vi "Omniax_mDrive_XYZR_2012.vi"() -> ()   [LabVIEW 2015]
uses:
  <vilib>/Utility/file.llb/Read From Spreadsheet File (I64).vi
  <vilib>/Utility/file.llb/Read From Spreadsheet File (string).vi
  <vilib>/Instr/_visa.llb/VISA Configure Serial Port (Instr).vi
  <vilib>/Utility/file.llb/Write To Spreadsheet File (I64).vi
  <vilib>/Utility/file.llb/Write To Spreadsheet File (string).vi
panel:
  in  "Submit":bool
  in  "ELOG":string
  out "Z max step":i32
  in  "V5 position 15360000":i32
  out "IV5CL":bool
  out "IV5OP":bool
  out "R Velocity MVdeg/sec":dbl format="%.3f"
  out "R Position MV deg":dbl
  out "Z Velocity MV mm/sec":dbl format="%.3f"
  out "Z Position MV mm":dbl
  out "Y Velocity MV mm/sec":dbl format="%.3f"
  out "Y Position MV mm":dbl
  out "X Velocity MV mm/sec":dbl format="%.3f"
  out "X Position MV mm":dbl
  out "Presets":i32[][](array[numeric])
  in  "stop":bool
  in  "Tab Control 3":enum32{"Status", "Reset"}(tab)
  out "Y in Range":bool
  out "Y Scan":bool
  out "Y in Motion":bool
  out "Y Backlash corr":bool
  out "X  in Range":bool
  out "X Scan":bool
  out "X  in Motion":bool
  out "X Backlash corr":bool
  out "Z in Range":bool
  out "Z Scan":bool
  out "Z in Motion":bool
  out "Z Backlash corr":bool
  out "R in Range":bool
  out "R Scan":bool
  out "R in Motion":bool
  out "R Backlash corr":bool
  out "X Ready":bool
  out "Y Ready":bool
  out "Z Ready":bool
  out "R Ready":bool
  in  "Reset Y Position mm":dbl
  out "Reset Y Motor Steps":i32
  in  "Reset X Position mm":dbl
  out "Reset X Motor Steps":i32
  in  "Reset Z Position mm":dbl
  out "Reset Z Motor Steps":i32
  in  "Reset R Position deg":dbl
  out "Reset R Motor Steps":i32
  in  "Reset":bool
  in  "Tab Control 2":enum32{"mm", "step"}(tab)
  in  "X Scan Length SP mm":dbl
  in  "X Scan Velocity SP mm/sec":dbl
  in  "X Scan set":bool
  in  "Y Scan Length SP mm":dbl
  in  "Y Scan Velocity SP mm/sec":dbl
  in  "Y Scan set":bool
  in  "Z Scan Length SP mm":dbl
  in  "Z Scan Velocity SP mm/sec":dbl
  in  "Z Scan set":bool
  in  "R Scan Length SP deg":dbl
  in  "R Scan Velocity SP deg/sec":dbl
  in  "R Scan set":bool
  in  "X Scan Velocity SP steps/sec":i32=1 min=1 max=102400 step=1
  in  "X Scan Length SP steps":i32 min=-2816000 max=1792000 step=100
  out "X Scan length MV mm":dbl
  out "X Scan velocity MV mm/sec":dbl format="%#_6f"
  in  "Y Scan Velocity SP steps/sec":i32=1 min=1 max=102400 step=1
  in  "Y Scan Length SP steps":i32 min=-1930240 max=2677760 step=100
  out "Y Scan length MV mm":dbl
  out "Y Scan velocity MV mm/sec":dbl format="%#_6f"
  in  "Z Scan Velocity SP steps/sec":i32=1 min=1 max=102400 step=1
  in  "Z Scan Length SP steps":i32 min=-91980800 max=10419200 step=100
  out "Z Scan length MV mm":dbl
  out "Z Scan velocity MV mm/sec":dbl format="%#_6f"
  in  "R Scan Velocity SP steps/sec":i32=1 min=1 max=102400 step=1
  in  "R Scan Length SP steps":i32 min=-1501867 max=10786133 step=100
  out "R Scan length MV deg":dbl
  out "R Scan velocity MV deg/sec":dbl format="%#_6f"
  out "atan Y/Z":dbl
  in  "Tab Control":enum32{"mm", "preset", "step"}(tab)
  in  "X Position SP mm":dbl
  in  "X Velocity SP mm/sec":dbl
  in  "X Move Set":bool
  in  "Y Move Set":bool
  in  "Y Position SP mm":dbl
  in  "Y Velocity SP mm/sec":dbl
  in  "Z Position SP mm":dbl
  in  "Z Velocity SP mm/sec":dbl
  in  "Z Move Set":bool
  in  "R Position SP deg":dbl
  in  "R Velocity SP deg/sec":dbl
  in  "R Move Set":bool
  in  "Add Button":bool
  in  "String":string
  in  "Delete Button":bool
  in  "Preset positions":i32(ring) items=["ZERO", "Default", "CDOSE", "QMS", "test", "test2", "test3", "yag position", "Sample Long Edge  ", "SPUTTER POS"]
  in  "Set Button":bool
  in  "X Velocity SP step/sec":i32 min=1 max=128000
  in  "Y Velocity SP step/sec":i32 min=1 max=128000
  in  "Z Velocity SP step/sec":i32 min=1 max=204800
  in  "R Velocity SP step/sec":i32 min=1 max=10000
  in  "Y Step SP":i32=-20000 min=-2304000 max=2304000 step=500
  in  "X Step SP":i32=-20000 min=-2304000 max=2304000 step=500
  in  "Z Step SP":i32=-20000 min=0 max=102400000 step=500
  in  "R Step SP":i32=-20000 min=-6144000 max=6144000 step=500
  out "X Step PV":i32 max=2000
  out "Y Step PV":i32 max=2000
  out "Z Step PV":i32 max=2000
  out "R Step PV":i32 max=2000
  in  "Clear ZY":bool
  out "ZY Graph":cluster{"Y":dbl[], "Y":dbl[]}[](graph)
  out "ZR Graph":cluster{"Y":dbl[], "Y":dbl[]}[](graph)
  out "XY Graph":cluster{"Y":dbl[], "Y":dbl[]}[](graph)
  out "X Scan Duration":dbl
  out "Y Scan Duration":dbl
  out "Z Scan Duration":dbl
  out "R Scan Duration":dbl
  out "R Backlash steps/sec":i32
  out "R Backlash":i32
  out "R Holding Current %":i32
  out "R Run Current %":i32
  out "R offset deg":dbl
  out "R deg/rev":dbl
  out "R steps/rev":u32
  out "R velocity PV step/sec":i32
  out "R MINPOS":i32=-94296
  out "R MAXPOS":i32=-34296
  out "R COM PORT":refnum<visa-resource-name>="COM5"
  in  "R Scan OK":bool
  in  "R Go":bool
  out "R Position deg PV":dbl
  out "Z COM PORT":refnum<visa-resource-name>="COM5"
  out "Z Backlash steps/sec":i32
  out "Z Backlash":i32
  out "Z Holding Current %":i32
  out "Z Run Current %":i32
  out "Z offset mm":dbl
  out "Z mm/rev":dbl
  out "Z steps/rev":u32
  out "Z  velocity PV step/sec":i32
  out "Z MINPOS":i32=-94296
  out "Z MAXPOS":i32=-34296
  in  "Z Scan OK":bool
  in  "Z Go":bool
  out "Z Position mm PV":dbl
  out "X Position mm PV":dbl
  out "X velocity PV step/sec":i32
  in  "X Scan OK":bool
  in  "X Go":bool
  out "X Backlash steps/sec":i32
  out "X Backlash":i32
  out "X Holding Current %":i32
  out "X Run Current %":i32
  out "X offset mm":dbl
  out "X mm/rev":dbl
  out "X steps/rev":u32
  out "X MAXPOS":i32=-34296
  out "X MINPOS":i32=-94296
  out "X COM PORT":refnum<visa-resource-name>="COM5"
  out "Y Backlash steps/sec":i32
  out "Y Backlash":i32
  out "Y Holding Current %":i32
  out "Y Run Current %":i32
  in  "Scan Cancel":bool
  out "Y Position mm PV":dbl
  out "Y offset mm":dbl
  out "Y mm/rev":dbl
  out "Y steps/rev":u32
  out "Y velocity PV step/sec":i32
  in  "Y Scan OK":bool
  in  "Scan Go":bool
  in  "Stop":bool
  in  "Y Go":bool
  out "Y MINPOS":i32=-94296
  out "Y MAXPOS":i32=-34296
  out "Y COM PORT":refnum<visa-resource-name>="COM5"
  # "12-15"
  # "Current position"
  # "Goto position"
  # "MX"
  # "MY"
  # "V5"
  # "MZ"
  # "MR"
  # "L"
  # "M"
  # "B"
  # "S"
  # "R"
  # "Preset position"
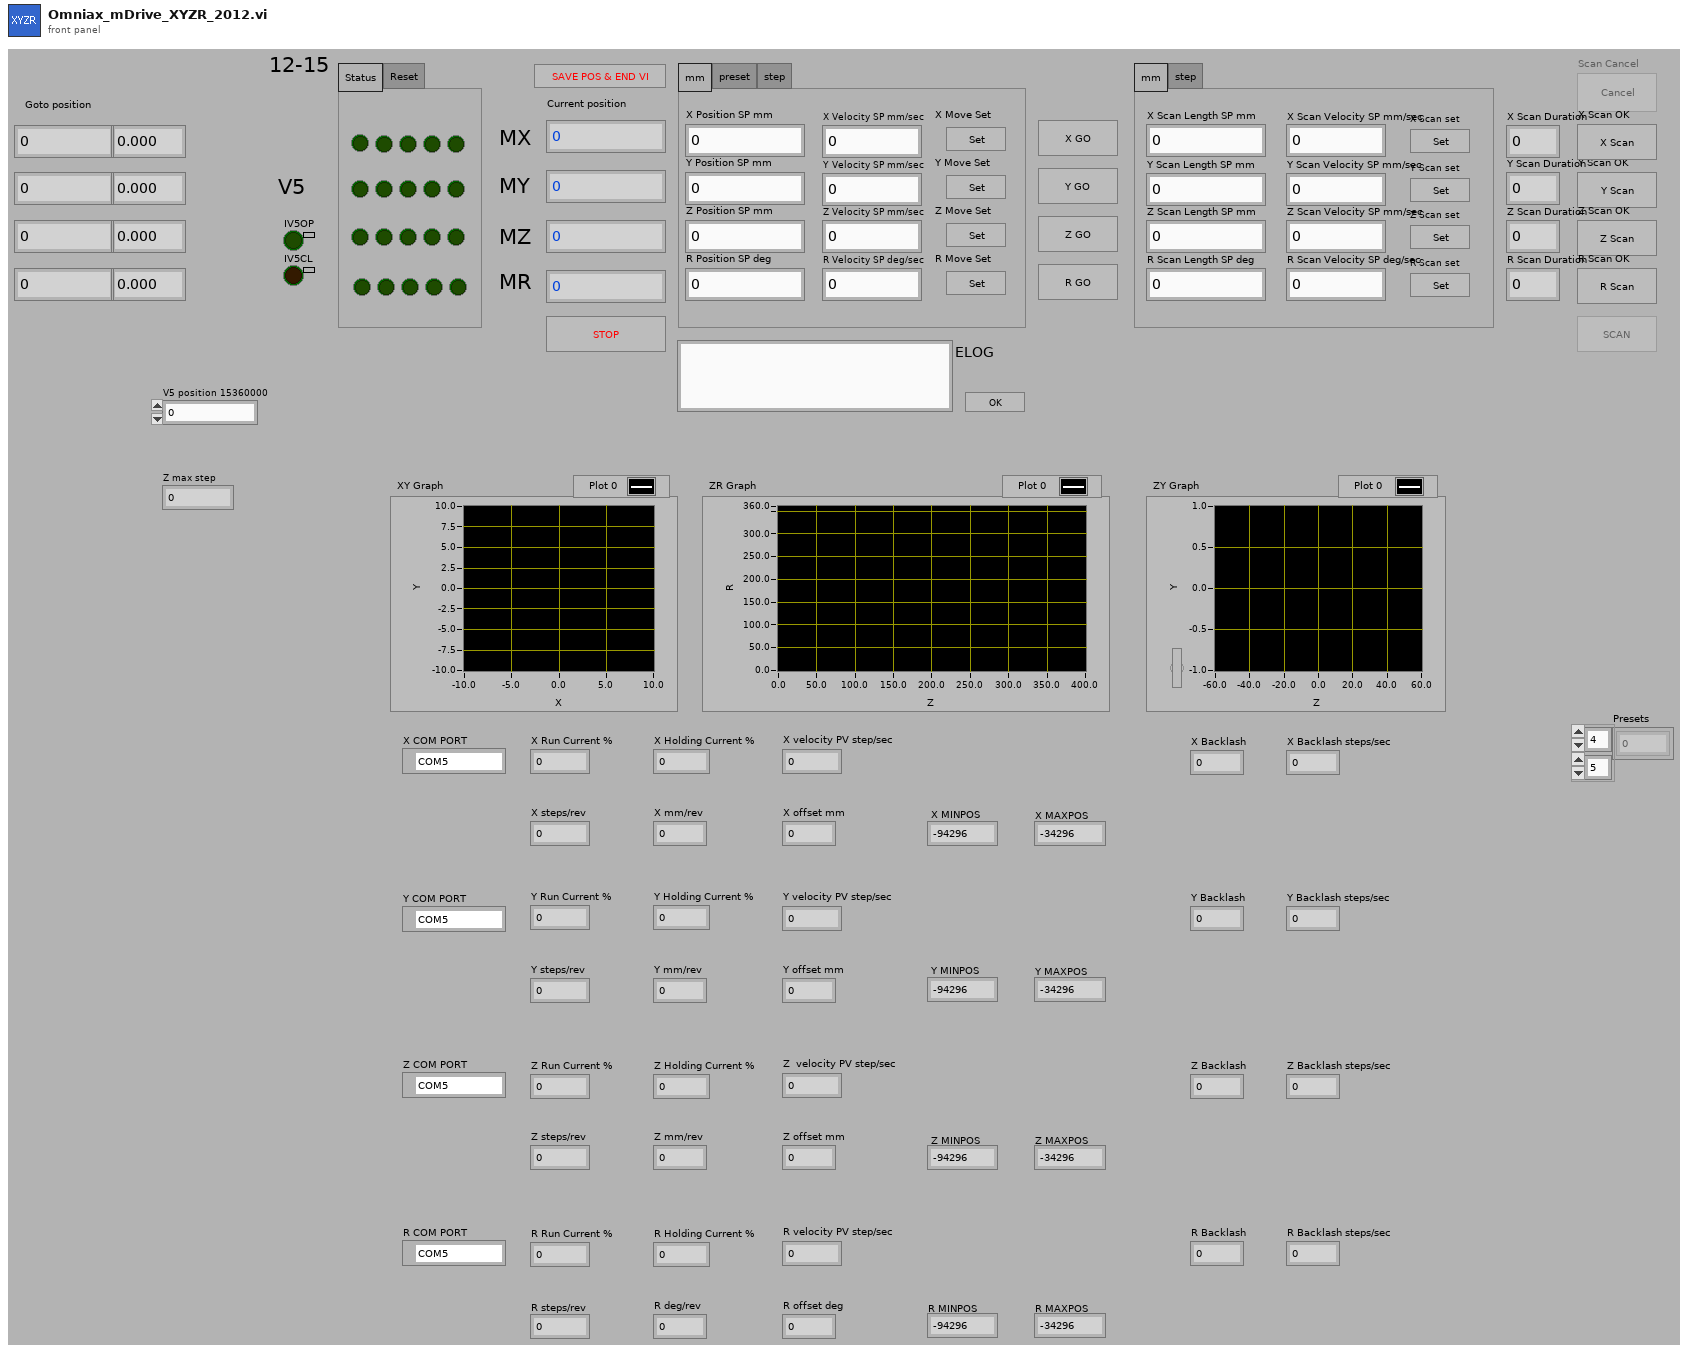
[diagram p1: front panel]
types:
  T1 = enum16{"Stop", "Reset", "Run Current", "Holding Current", "Accel Rate", "Decel Rate", "Move to Relative Position", "Move to Absolute Position", "Echo Mode", "Print Parameter", "Send String", "Microstep Resolution", "Set Current Position", "Max Velocity"}
  T2 = enum8{"Enabled", "Disabled", "Disabled and Grayed Out"}
  T3 = cluster{"first row[0]":i64, "first row[1]":i64, "first row[2]":i64, "first row[3]":i64, "first row[4]":i64, "first row[5]":i64, "first row[6]":i64, "first row[7]":i64, "first row[8]":i64}
  T4 = enum16{"open", "replace", "create", "open or create", "replace or create", "replace or create with confirmation"}
  T5 = cluster{"Value[0]":i32, "Value[1]":i32, "Value[2]":i32, "Value[3]":i32, "Value[4]":i32, "Value[5]":i32, "Value[6]":i32, "Value[7]":i32, "Value[8]":i32}
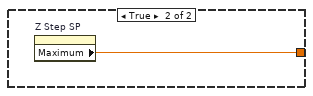
[diagram p6: hidden frame]
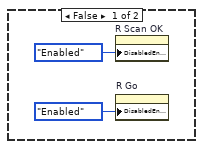
[diagram p7: hidden frame]
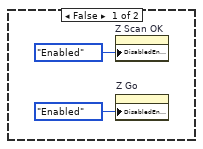
[diagram p10: hidden frame]
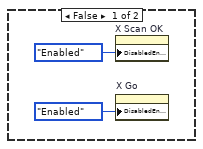
[diagram p13: hidden frame]
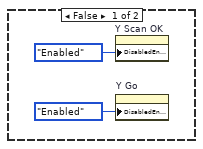
[diagram p16: hidden frame]
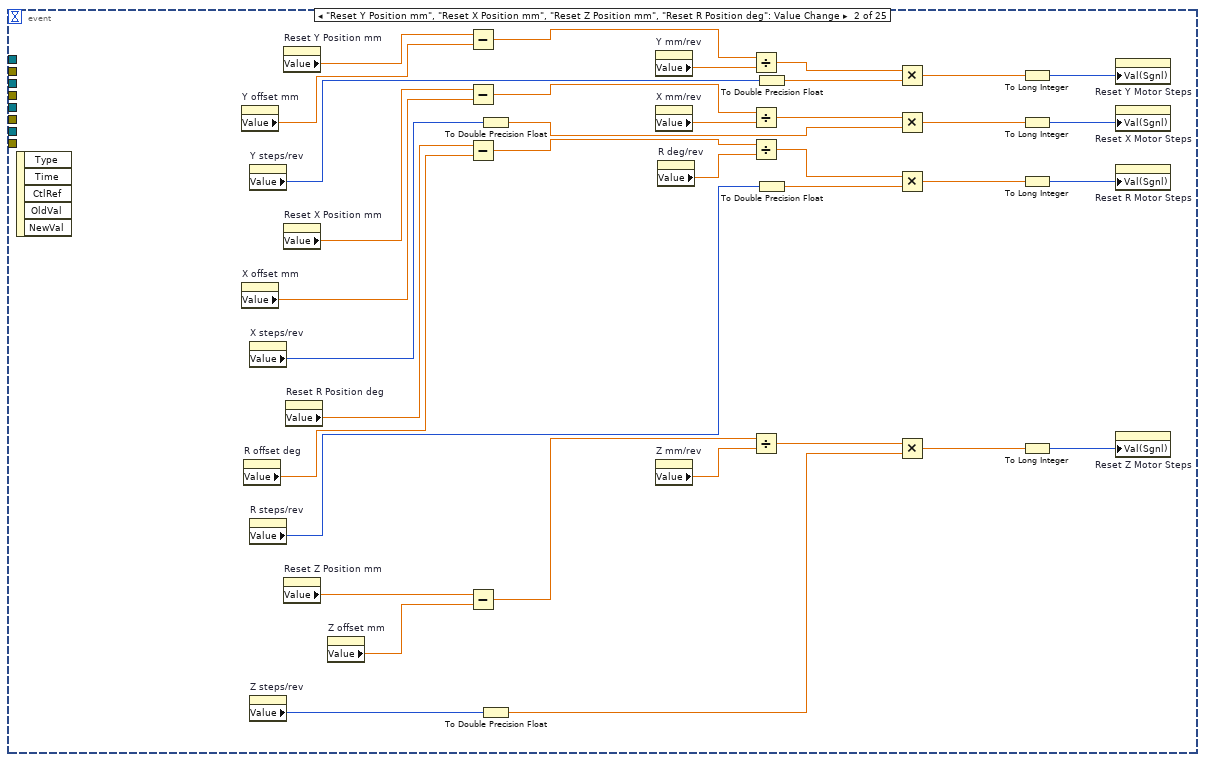
[diagram p19: hidden frame]
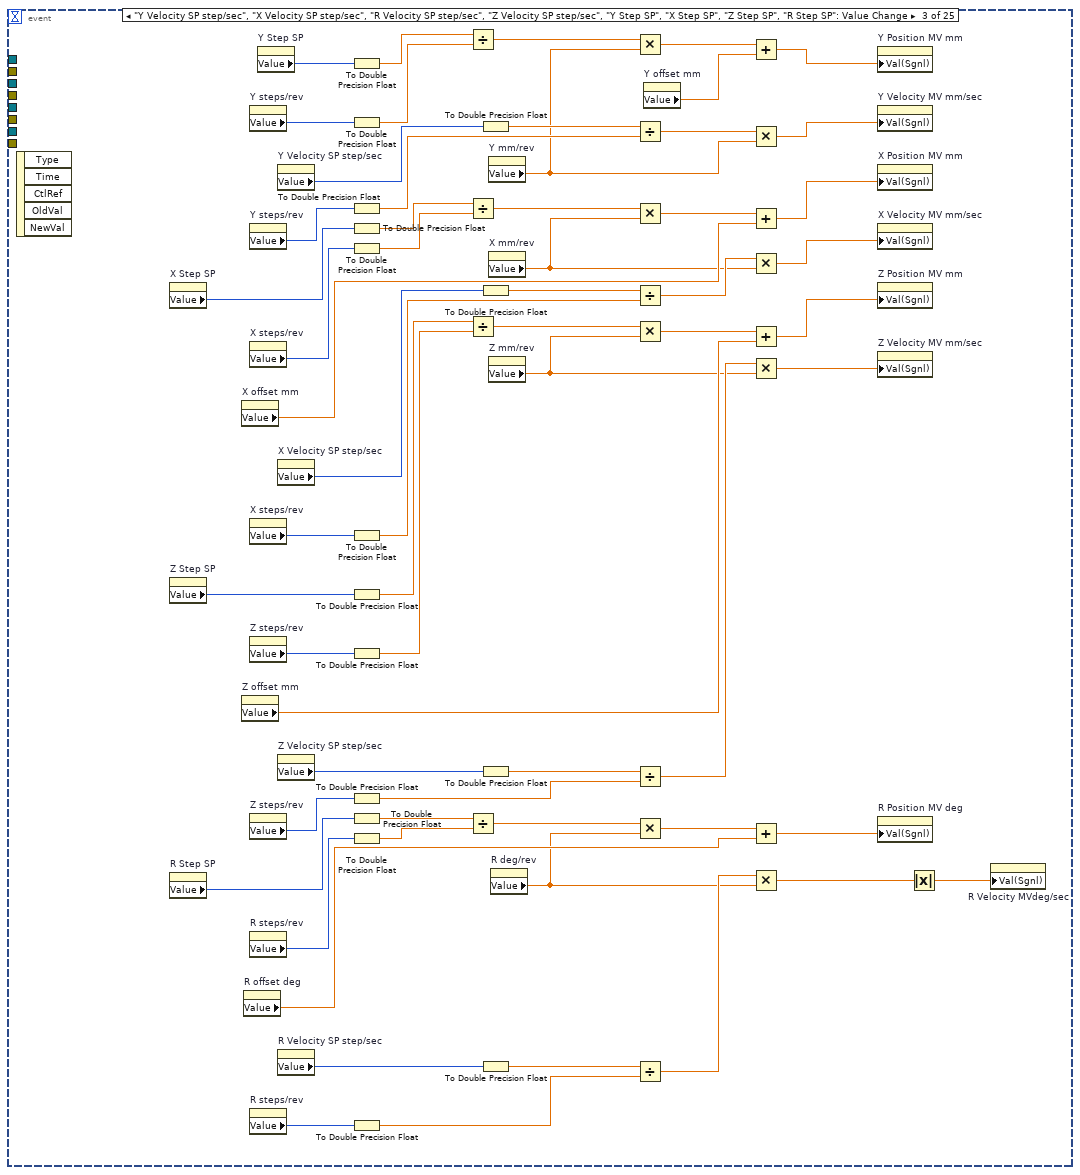
[diagram p20: hidden frame]
diagram:
  w4 = 0 ("dimension size")
  n1 = call "DigitalIO_sub_V5_MON.vi"() -> ("CL"=→"IV5CL":bool, "OP"=→"IV5OP":bool)  [unwired: 8 in]
  n2 = flat-sequence {
    tunnel: [w108] -> w36
    tunnel: [w107] -> w35
    tunnel: [w118] -> w52
    tunnel: [w116] -> w50
    tunnel: w36 -> [w119]
    tunnel: w35 -> [w117]
    tunnel: w52 -> [w125]
    tunnel: [w126] -> w51
    tunnel: w50 -> [w122]
    tunnel: [w124] -> w49
    tunnel: [w135] -> w102
    tunnel: [w137] -> w100
    tunnel: w51 -> [w136]
    tunnel: w49 -> [w138]
    tunnel: w102 -> [w145]
    tunnel: [w144] -> w101
    tunnel: w100 -> [w142]
    tunnel: [w143] -> w99
    tunnel: [w155] -> w104
    tunnel: [w156] -> w103
    tunnel: w101 -> [w154]
    tunnel: w99 -> [w153]
    tunnel: w104 -> [w166]
    tunnel: w103 -> [w165]
    tunnel: [w168] -> w88
    tunnel: [w167] -> w87
    tunnel: [w162] -> w86
    tunnel: [w173] -> w105
    tunnel: [w174] -> w106
    tunnel: w88 -> [w174]
    tunnel: w87 -> [w173]
    tunnel: w86 -> [w169]
    frame #0 {
      w115 = refnum<visa-resource-name> "COM13" ("COM PORT")
      w113 = u16 0 items=["None", "XON/XOFF", "RTS/CTS", "XON/XOFF & RTS/CTS", "DTR/DSR", "XON/XOFF & DTR/DSR"] ("flow control (0:none)")
      w112 = u16 10 items=["1.0"=10, "1.5"=15, "2.0"=20] ("stop bits (10: 1 bit)")
      # "Stop bits"
      n3 = call-poly "VISA Configure Serial Port"("VISA resource name"=w115, "timeout (10sec)"=u32 10000, "baud rate (9600)"=u32 9600, "data bits (8)"=u16 8, "parity (0:none)"=enum16{"None", "Odd", "Even", "Mark", "Space"}."None", "stop bits (10: 1 bit)"=w112, "flow control (0:none)"=w113) -> ("VISA resource name out"=w108:refnum<visa-resource-name>, "error out"=w107:errorcluster)  [unwired: 7 in]
      "Y COM PORT" <- w115
    }
    frame #1 {
      n4 = call "mDrive Send Command.vi"("error in (no error)"=w117, "Extra"="EM=2", "Command"=T1."Send String", "VISA resource name"=w119) -> ("error out"=w116:errorcluster, "VISA resource name out"=w118:refnum<visa-resource-name>)  [unwired: 3 in, 1 out]
    }
    frame #2 {
      n5 = Number To Decimal String(number=1000000) -> (decimal integer string=w127:string)  [unwired: 1 in]
      n6 = call "mDrive Send Command.vi"("error in (no error)"=w122, "Extra"=w127, "Command"=T1."Accel Rate", "VISA resource name"=w125) -> ("error out"=w123:errorcluster, "VISA resource name out"=w131:refnum<visa-resource-name>)  [unwired: 3 in, 1 out]
      n7 = call "mDrive Send Command.vi"("error in (no error)"=w123, "Extra"=w127, "Command"=T1."Decel Rate", "VISA resource name"=w131) -> ("error out"=w124:errorcluster, "VISA resource name out"=w126:refnum<visa-resource-name>)  [unwired: 3 in, 1 out]
    }
    frame #3 {
      # "Run Current %"
      n8 = property on="Y Run Current %" class="DigNum (strict)"() -> ("Value"=w133:i32)  [unwired: 2 in, 2 out]
      n9 = Number To Decimal String(number=w133) -> (decimal integer string=w134:string)  [unwired: 1 in]
      n10 = call "mDrive Send Command.vi"("error in (no error)"=w138, "Extra"=w134, "Command"=T1."Run Current", "VISA resource name"=w136) -> ("error out"=w137:errorcluster, "VISA resource name out"=w135:refnum<visa-resource-name>)  [unwired: 3 in, 1 out]
    }
    frame #4 {
      # "Holding Current %"
      n11 = property on="Y Holding Current %" class="DigNum (strict)"() -> ("Value"=w140:i32)  [unwired: 2 in, 2 out]
      n12 = Number To Decimal String(number=w140) -> (decimal integer string=w141:string)  [unwired: 1 in]
      n13 = call "mDrive Send Command.vi"("error in (no error)"=w142, "Extra"=w141, "Command"=T1."Holding Current", "VISA resource name"=w145) -> ("error out"=w143:errorcluster, "VISA resource name out"=w144:refnum<visa-resource-name>)  [unwired: 3 in, 1 out]
    }
    frame #5 {
      # "Velocity Max"
      n14 = property on="Y Velocity SP step/sec" class="DigNum (strict)"() -> ("Value"=w152:i32)  [unwired: 2 in, 2 out]
      n15 = Number To Decimal String(number=w152) -> (decimal integer string=w151:string)  [unwired: 1 in]
      n16 = call "mDrive Send Command.vi"("error in (no error)"=w153, "Extra"=w151, "Command"=T1."Max Velocity", "VISA resource name"=w154) -> ("error out"=w149:errorcluster, "VISA resource name out"=w159:refnum<visa-resource-name>)  [unwired: 3 in, 1 out]
      n17 = call "mDrive Send Command.vi"("error in (no error)"=w149, "Extra"="VM", "Command"=T1."Print Parameter", "VISA resource name"=w159) -> ("error out"=w156:errorcluster, "read buffer"=w157:string, "VISA resource name out"=w155:refnum<visa-resource-name>)  [unwired: 3 in]
      n18 = Decimal String To Number(string=w157, offset=0) -> (number=w150:i32)  [unwired: 1 in, 1 out]
      n19 = property on="Y scan velocity MV step/sec" class="DigNum (strict)"("Val(Sgnl)"=w150) -> ()  [unwired: 2 in, 2 out]
    }
    frame #6 {
      # "PRINT POSITION"
      n20 = call "mDrive Send Command.vi"("error in (no error)"=w165, "Extra"="P", "Command"=T1."Print Parameter", "VISA resource name"=w166) -> ("error out"=w167:errorcluster, "read buffer"=w164:string, "VISA resource name out"=w168:refnum<visa-resource-name>)  [unwired: 3 in]
      n21 = Decimal String To Number(string=w164, offset=0) -> (number=w162:i32)  [unwired: 1 in, 1 out]
    }
    frame #7 {
      w171 = -2304000 ("lower limit")
      w172 = 2304000 ("upper limit")
      n22 = property on="Y Step SP" class="DigNum (strict)"("Val(Sgnl)"=w169) -> ()  [unwired: 2 in, 2 out]
      n23 = property on="Y Step SP" class="DigNum (strict)"("Maximum"=w172) -> ()  [unwired: 2 in, 2 out]
      n24 = In Range and Coerce(upper limit=w172, x=w169, lower limit=w171) -> (In Range?=w170:bool)  [unwired: 1 out]
      n25 = property on="Y Step SP" class="DigNum (strict)"("Minimum"=w171) -> ()  [unwired: 2 in, 2 out]
      n26 = property on="Y in Range" class="Bool (strict)"("Val(Sgnl)"=w170) -> ()  [unwired: 2 in, 2 out]
      "Y MINPOS" <- w171
      "Y MAXPOS" <- w172
    }
  }
  n27 = flat-sequence {
    tunnel: [w176] -> w38
    tunnel: [w175] -> w37
    tunnel: [w184] -> w56
    tunnel: [w186] -> w54
    tunnel: w38 -> [w185]
    tunnel: w37 -> [w187]
    tunnel: w56 -> [w191]
    tunnel: [w192] -> w55
    tunnel: w54 -> [w190]
    tunnel: [w193] -> w53
    tunnel: [w204] -> w73
    tunnel: [w206] -> w72
    tunnel: w55 -> [w205]
    tunnel: w53 -> [w200]
    tunnel: w73 -> [w213]
    tunnel: [w212] -> w71
    tunnel: w72 -> [w210]
    tunnel: [w211] -> w70
    tunnel: [w223] -> w69
    tunnel: [w224] -> w68
    tunnel: w71 -> [w222]
    tunnel: w70 -> [w221]
    tunnel: w69 -> [w234]
    tunnel: w68 -> [w233]
    tunnel: [w236] -> w67
    tunnel: [w235] -> w66
    tunnel: [w230] -> w65
    tunnel: [w243] -> w61
    tunnel: [w244] -> w62
    tunnel: w67 -> [w244]
    tunnel: w66 -> [w243]
    tunnel: w65 -> [w241]
    frame #0 {
      w183 = refnum<visa-resource-name> "COM15" ("COM PORT")
      w181 = u16 0 items=["None", "XON/XOFF", "RTS/CTS", "XON/XOFF & RTS/CTS", "DTR/DSR", "XON/XOFF & DTR/DSR"] ("flow control (0:none)")
      w180 = u16 10 items=["1.0"=10, "1.5"=15, "2.0"=20] ("stop bits (10: 1 bit)")
      # "Stop bits"
      n28 = call-poly "VISA Configure Serial Port"("VISA resource name"=w183, "timeout (10sec)"=u32 10000, "baud rate (9600)"=u32 9600, "data bits (8)"=u16 8, "parity (0:none)"=enum16{"None", "Odd", "Even", "Mark", "Space"}."None", "stop bits (10: 1 bit)"=w180, "flow control (0:none)"=w181) -> ("VISA resource name out"=w176:refnum<visa-resource-name>, "error out"=w175:errorcluster)  [unwired: 7 in]
      "R COM PORT" <- w183
    }
    frame #1 {
      n29 = call "mDrive Send Command.vi"("error in (no error)"=w187, "Extra"="EM=2", "Command"=T1."Send String", "VISA resource name"=w185) -> ("error out"=w186:errorcluster, "VISA resource name out"=w184:refnum<visa-resource-name>)  [unwired: 3 in, 1 out]
    }
    frame #2 {
      # "pr=1000000"
      n30 = Number To Decimal String(number=100000) -> (decimal integer string=w195:string)  [unwired: 1 in]
      n31 = call "mDrive Send Command.vi"("error in (no error)"=w190, "Extra"=w195, "Command"=T1."Accel Rate", "VISA resource name"=w191) -> ("error out"=w194:errorcluster, "VISA resource name out"=w199:refnum<visa-resource-name>)  [unwired: 3 in, 1 out]
      n32 = call "mDrive Send Command.vi"("error in (no error)"=w194, "Extra"=w195, "Command"=T1."Decel Rate", "VISA resource name"=w199) -> ("error out"=w193:errorcluster, "VISA resource name out"=w192:refnum<visa-resource-name>)  [unwired: 3 in, 1 out]
    }
    frame #3 {
      # "Run Current %"
      n33 = property on="R Run Current %" class="DigNum (strict)"() -> ("Value"=w202:i32)  [unwired: 2 in, 2 out]
      n34 = Number To Decimal String(number=w202) -> (decimal integer string=w203:string)  [unwired: 1 in]
      n35 = call "mDrive Send Command.vi"("error in (no error)"=w200, "Extra"=w203, "Command"=T1."Run Current", "VISA resource name"=w205) -> ("error out"=w206:errorcluster, "VISA resource name out"=w204:refnum<visa-resource-name>)  [unwired: 3 in, 1 out]
    }
    frame #4 {
      # "Holding Current %"
      n36 = property on="R Holding Current %" class="DigNum (strict)"() -> ("Value"=w208:i32)  [unwired: 2 in, 2 out]
      n37 = Number To Decimal String(number=w208) -> (decimal integer string=w209:string)  [unwired: 1 in]
      n38 = call "mDrive Send Command.vi"("error in (no error)"=w210, "Extra"=w209, "Command"=T1."Holding Current", "VISA resource name"=w213) -> ("error out"=w211:errorcluster, "VISA resource name out"=w212:refnum<visa-resource-name>)  [unwired: 3 in, 1 out]
    }
    frame #5 {
      # "Print Velocity Max"
      # "Velocity Max"
      n39 = property on="R Velocity SP step/sec" class="DigNum (strict)"() -> ("Value"=w220:i32)  [unwired: 2 in, 2 out]
      n40 = Number To Decimal String(number=w220) -> (decimal integer string=w219:string)  [unwired: 1 in]
      n41 = call "mDrive Send Command.vi"("error in (no error)"=w221, "Extra"=w219, "Command"=T1."Max Velocity", "VISA resource name"=w222) -> ("error out"=w217:errorcluster, "VISA resource name out"=w227:refnum<visa-resource-name>)  [unwired: 3 in, 1 out]
      n42 = call "mDrive Send Command.vi"("error in (no error)"=w217, "Extra"="VM", "Command"=T1."Print Parameter", "VISA resource name"=w227) -> ("error out"=w224:errorcluster, "read buffer"=w225:string, "VISA resource name out"=w223:refnum<visa-resource-name>)  [unwired: 3 in]
      n43 = Decimal String To Number(string=w225, offset=0) -> (number=w218:i32)  [unwired: 1 in, 1 out]
      n44 = property on="R velocity PV step/sec" class="DigNum (strict)"("Val(Sgnl)"=w218) -> ()  [unwired: 2 in, 2 out]
    }
    frame #6 {
      # "PRINT POSITION"
      n45 = call "mDrive Send Command.vi"("error in (no error)"=w233, "Extra"="P", "Command"=T1."Print Parameter", "VISA resource name"=w234) -> ("error out"=w235:errorcluster, "read buffer"=w232:string, "VISA resource name out"=w236:refnum<visa-resource-name>)  [unwired: 3 in]
      n46 = Decimal String To Number(string=w232, offset=0) -> (number=w230:i32)  [unwired: 1 in, 1 out]
    }
    frame #7 {
      n47 = property on="R Step SP" class="DigNum (strict)"("Val(Sgnl)"=w241) -> ()  [unwired: 2 in, 2 out]
      n48 = property on="R Step SP" class="DigNum (strict)"() -> ("Maximum"=w240:dbl)  [unwired: 2 in, 2 out]
      n49 = property on="R Step SP" class="DigNum (strict)"() -> ("Minimum"=w239:dbl)  [unwired: 2 in, 2 out]
      n50 = To Long Integer(number=w240) -> (32bit integer=w237:i32)
      "R MAXPOS" <- w237
      n51 = To Long Integer(number=w239) -> (32bit integer=w238:i32)
      "R MINPOS" <- w238
      n52 = In Range and Coerce(upper limit=w237, x=w241, lower limit=w238) -> (In Range?=w242:bool)  [unwired: 1 out]
      n53 = property on="R in Range" class="Bool (strict)"("Val(Sgnl)"=w242) -> ()  [unwired: 2 in, 2 out]
    }
  }
  n54 = flat-sequence {
    frame #0 {
      w250 = -3.0 ("R deg/rev")
      w248 = u32 51200 ("step/rev")
      w252 = 10000 ("Value (Signaling)")
      n55 = To Double Precision Float(number=w252) -> (double precision float=w254:dbl)
      n56 = To Double Precision Float(number=w248) -> (double precision float=w249:dbl)
      n57 = property on="R Velocity SP step/sec" class="DigNum (strict)"("Val(Sgnl)"=w252) -> ()  [unwired: 2 in, 2 out]
      n58 = property on="R Velocity SP step/sec" class="DigNum (strict)"("Minimum"=1.0 ("Data Entry Limits:Minimum")) -> ()  [unwired: 2 in, 2 out]
      n59 = Divide(x=w254, y=w249) -> (x/y=w253:dbl)
      n60 = property on="R Velocity SP step/sec" class="DigNum (strict)"("Maximum"=w254) -> ()  [unwired: 2 in, 2 out]
      n61 = Multiply(x=w253, y=w250) -> (x*y=w251:dbl)
      n62 = Absolute Value(x=w251) -> (abs(x)=w245:dbl)
      n63 = property on="R Velocity SP deg/sec" class="DigNum (strict)"("Val(Sgnl)"=w245) -> ()  [unwired: 2 in, 2 out]
      "R offset deg" <- 0.0 ("R offset deg")
      "R deg/rev" <- w250
      "R steps/rev" <- w248
    }
  }
  n64 = flat-sequence {
    frame #0 {
      w256 = 0.2 ("Z mm/rev")
      w255 = u32 51200 ("step/rev")
      w257 = 204800 ("Value (Signaling)")
      n65 = To Double Precision Float(number=w257) -> (double precision float=w261:dbl)
      n66 = To Double Precision Float(number=w255) -> (double precision float=w260:dbl)
      n67 = property on="Z Velocity SP step/sec" class="DigNum (strict)"("Val(Sgnl)"=w257) -> ()  [unwired: 2 in, 2 out]
      n68 = property on="Z Velocity SP step/sec" class="DigNum (strict)"("Minimum"=1.0 ("Data Entry Limits:Minimum")) -> ()  [unwired: 2 in, 2 out]
      n69 = Divide(x=w261, y=w260) -> (x/y=w258:dbl)
      n70 = property on="Z Velocity SP step/sec" class="DigNum (strict)"("Maximum"=w261) -> ()  [unwired: 2 in, 2 out]
      n71 = Multiply(x=w258, y=w256) -> (x*y=w259:dbl)
      n72 = property on="Z Velocity SP mm/sec" class="DigNum (strict)"("Val(Sgnl)"=w259) -> ()  [unwired: 2 in, 2 out]
      "Z offset mm" <- 0.0 ("Z offset mm")
      "Z mm/rev" <- w256
      "Z steps/rev" <- w255
    }
  }
  n73 = flat-sequence {
    frame #0 {
      n74 = property on="X Backlash corr" class="Bool (strict)"("Val(Sgnl)"=FALSE ("Value (Signaling)")) -> ()  [unwired: 2 in, 2 out]
      n75 = property on="Z Backlash corr" class="Bool (strict)"("Val(Sgnl)"=FALSE ("Value (Signaling)")) -> ()  [unwired: 2 in, 2 out]
      n76 = property on="R Backlash corr" class="Bool (strict)"("Val(Sgnl)"=FALSE ("Value (Signaling)")) -> ()  [unwired: 2 in, 2 out]
      n77 = property on="Y Backlash corr" class="Bool (strict)"("Val(Sgnl)"=FALSE ("Value (Signaling)")) -> ()  [unwired: 2 in, 2 out]
      "Z Backlash steps/sec" <- 25600 ("Z Backlash steps/sec")
      "Z Backlash" <- -51200 ("Z Backlash")
      "X Backlash steps/sec" <- 25600 ("Value (Signaling)")
      "X Backlash" <- 10240 ("Backlash2")
      "Y Backlash" <- -10240 ("Backlash2")
      "Y Backlash steps/sec" <- 25600 ("Value (Signaling)")
      "R Backlash steps/sec" <- 6400 ("R Backlash steps/sec")
      "R Backlash" <- -12800 ("R Backlash")
    }
  }
  n78 = flat-sequence {
    frame #0 {
      "Z Holding Current %" <- 20 ("Z Holding Current %")
      "Z Run Current %" <- 40 ("Z Run Current %")
      "X Run Current %" <- 40 ("Run Current %")
      "X Holding Current %" <- 20 ("Holding Current %")
      "Y Run Current %" <- 40 ("Run Current %")
      "Y Holding Current %" <- 20 ("Holding Current %")
      "R Holding Current %" <- 15 ("R Holding Current %")
      "R Run Current %" <- 80 ("R Run Current %")
    }
  }
  n79 = flat-sequence {
    frame #0 {
      n80 = property on="X Scan" class="Bool (strict)"("Val(Sgnl)"=FALSE ("Value (Signaling)")) -> ()  [unwired: 2 in, 2 out]
      n81 = property on="Y Scan Velocity SP mm/sec" class="DigNum (strict)"("Val(Sgnl)"=0.1 ("Value (Signaling)")) -> ()  [unwired: 2 in, 2 out]
      n82 = property on="Z Scan" class="Bool (strict)"("Val(Sgnl)"=FALSE ("Value (Signaling)")) -> ()  [unwired: 2 in, 2 out]
      n83 = property on="R Scan" class="Bool (strict)"("Val(Sgnl)"=FALSE ("Value (Signaling)")) -> ()  [unwired: 2 in, 2 out]
      n84 = property on="R Velocity SP deg/sec" class="DigNum (strict)"("Val(Sgnl)"=0.1 ("Value (Signaling)")) -> ()  [unwired: 2 in, 2 out]
      n85 = property on="Z Scan Velocity SP mm/sec" class="DigNum (strict)"("Val(Sgnl)"=0.1 ("Value (Signaling)")) -> ()  [unwired: 2 in, 2 out]
      n86 = property on="Y Scan" class="Bool (strict)"("Val(Sgnl)"=FALSE ("Value (Signaling)")) -> ()  [unwired: 2 in, 2 out]
      n87 = property on="X Scan Velocity SP mm/sec" class="DigNum (strict)"("Val(Sgnl)"=0.1 ("Value (Signaling)")) -> ()  [unwired: 2 in, 2 out]
      n88 = property on="Scan Cancel" class="Bool"("DisabledEnum"=T2."Disabled and Grayed Out" ("Disabled")) -> ()  [unwired: 2 in, 2 out]
      n89 = property on="Scan Go" class="Bool"("DisabledEnum"=T2."Disabled and Grayed Out" ("Disabled")) -> ()  [unwired: 2 in, 2 out]
    }
  }
  n90 = flat-sequence {
    frame #0 {
      w296 = 0.2 ("MM/rev")
      w299 = u32 51200 ("step/rev")
      w294 = 128000 ("Value (Signaling)")
      # "a=1000000"
      n91 = property on="X Velocity SP step/sec" class="DigNum (strict)"("Minimum"=1.0 ("Data Entry Limits:Minimum")) -> ()  [unwired: 2 in, 2 out]
      n92 = To Double Precision Float(number=w294) -> (double precision float=w300:dbl)
      n93 = To Double Precision Float(number=w299) -> (double precision float=w298:dbl)
      n94 = property on="X Velocity SP step/sec" class="DigNum (strict)"("Val(Sgnl)"=w294) -> ()  [unwired: 2 in, 2 out]
      n95 = property on="X Velocity SP step/sec" class="DigNum (strict)"("Maximum"=w300) -> ()  [unwired: 2 in, 2 out]
      n96 = Divide(x=w300, y=w298) -> (x/y=w295:dbl)
      n97 = Multiply(x=w295, y=w296) -> (x*y=w297:dbl)
      n98 = property on="X Velocity SP mm/sec" class="DigNum (strict)"("Val(Sgnl)"=w297) -> ()  [unwired: 2 in, 2 out]
      "X offset mm" <- 0.0 ("offset")
      "X steps/rev" <- w299
      "X mm/rev" <- w296
    }
  }
  n99 = flat-sequence {
    frame #0 {
      w305 = 0.2 ("MM/rev")
      w308 = u32 51200 ("step/rev")
      w303 = 128000 ("Value (Signaling)")
      n100 = To Double Precision Float(number=w303) -> (double precision float=w309:dbl)
      n101 = To Double Precision Float(number=w308) -> (double precision float=w307:dbl)
      n102 = property on="Y Velocity SP step/sec" class="DigNum (strict)"("Val(Sgnl)"=w303) -> ()  [unwired: 2 in, 2 out]
      n103 = property on="Y Velocity SP step/sec" class="DigNum (strict)"("Minimum"=1.0 ("Data Entry Limits:Minimum")) -> ()  [unwired: 2 in, 2 out]
      n104 = Divide(x=w309, y=w307) -> (x/y=w304:dbl)
      n105 = property on="Y Velocity SP step/sec" class="DigNum (strict)"("Maximum"=w309) -> ()  [unwired: 2 in, 2 out]
      n106 = Multiply(x=w304, y=w305) -> (x*y=w306:dbl)
      n107 = property on="Y Velocity SP mm/sec" class="DigNum (strict)"("Val(Sgnl)"=w306) -> ()  [unwired: 2 in, 2 out]
      "Y offset mm" <- 0.0 ("offset")
      "Y steps/rev" <- w308
      "Y mm/rev" <- w305
    }
  }
  n108 = property on="Z Step SP" class="DigNum (strict)"("Minimum"=0 ("lower limit")) -> ()  [unwired: 2 in, 2 out]
  n109 = flat-sequence {
    tunnel: [w312] -> w42
    tunnel: [w313] -> w41
    tunnel: [w323] -> w48
    tunnel: [w322] -> w46
    tunnel: w42 -> [w324]
    tunnel: w41 -> [w321]
    tunnel: w48 -> [w334]
    tunnel: [w329] -> w47
    tunnel: w46 -> [w333]
    tunnel: [w333] -> w45
    tunnel: [w338] -> w82
    tunnel: [w340] -> w81
    tunnel: w47 -> [w339]
    tunnel: w45 -> [w341]
    tunnel: w82 -> [w348]
    tunnel: [w347] -> w80
    tunnel: w81 -> [w345]
    tunnel: [w346] -> w79
    tunnel: [w358] -> w78
    tunnel: [w359] -> w77
    tunnel: w80 -> [w357]
    tunnel: w79 -> [w356]
    tunnel: w78 -> [w369]
    tunnel: w77 -> [w368]
    tunnel: [w371] -> w76
    tunnel: [w370] -> w75
    tunnel: [w365] -> w74
    tunnel: [w378] -> w63
    tunnel: [w379] -> w64
    tunnel: w76 -> [w379]
    tunnel: w75 -> [w378]
    tunnel: w74 -> [w376]
    frame #0 {
      w320 = refnum<visa-resource-name> "COM14" ("COM PORT")
      w318 = u16 0 items=["None", "XON/XOFF", "RTS/CTS", "XON/XOFF & RTS/CTS", "DTR/DSR", "XON/XOFF & DTR/DSR"] ("flow control (0:none)")
      w317 = u16 10 items=["1.0"=10, "1.5"=15, "2.0"=20] ("stop bits (10: 1 bit)")
      # "Stop bits"
      n110 = call-poly "VISA Configure Serial Port"("VISA resource name"=w320, "timeout (10sec)"=u32 10000, "baud rate (9600)"=u32 9600, "data bits (8)"=u16 8, "parity (0:none)"=enum16{"None", "Odd", "Even", "Mark", "Space"}."None", "stop bits (10: 1 bit)"=w317, "flow control (0:none)"=w318) -> ("VISA resource name out"=w312:refnum<visa-resource-name>, "error out"=w313:errorcluster)  [unwired: 7 in]
      "Z COM PORT" <- w320
    }
    frame #1 {
      n111 = call "mDrive Send Command.vi"("error in (no error)"=w321, "Extra"="EM=2", "Command"=T1."Send String", "VISA resource name"=w324) -> ("error out"=w322:errorcluster, "VISA resource name out"=w323:refnum<visa-resource-name>)  [unwired: 3 in, 1 out]
    }
    frame #2 {
      n112 = Number To Decimal String(number=1000000) -> (decimal integer string=w327:string)  [unwired: 1 in]
      n113 = call "mDrive Send Command.vi"("Extra"=w327, "Command"=T1."Accel Rate", "VISA resource name"=w334) -> ("VISA resource name out"=w332:refnum<visa-resource-name>)  [unwired: 4 in, 2 out]
      n114 = call "mDrive Send Command.vi"("Extra"=w327, "Command"=T1."Decel Rate", "VISA resource name"=w332) -> ("VISA resource name out"=w329:refnum<visa-resource-name>)  [unwired: 4 in, 2 out]
    }
    frame #3 {
      # "Run Current %"
      n115 = property on="Z Run Current %" class="DigNum (strict)"() -> ("Value"=w336:i32)  [unwired: 2 in, 2 out]
      n116 = Number To Decimal String(number=w336) -> (decimal integer string=w337:string)  [unwired: 1 in]
      n117 = call "mDrive Send Command.vi"("error in (no error)"=w341, "Extra"=w337, "Command"=T1."Run Current", "VISA resource name"=w339) -> ("error out"=w340:errorcluster, "VISA resource name out"=w338:refnum<visa-resource-name>)  [unwired: 3 in, 1 out]
    }
    frame #4 {
      # "Holding Current %"
      n118 = property on="Z Run Current %" class="DigNum (strict)"() -> ("Value"=w343:i32)  [unwired: 2 in, 2 out]
      n119 = Number To Decimal String(number=w343) -> (decimal integer string=w344:string)  [unwired: 1 in]
      n120 = call "mDrive Send Command.vi"("error in (no error)"=w345, "Extra"=w344, "Command"=T1."Holding Current", "VISA resource name"=w348) -> ("error out"=w346:errorcluster, "VISA resource name out"=w347:refnum<visa-resource-name>)  [unwired: 3 in, 1 out]
    }
    frame #5 {
      # "Velocity Max"
      n121 = property on="Z Velocity SP step/sec" class="DigNum (strict)"() -> ("Value"=w355:i32)  [unwired: 2 in, 2 out]
      n122 = Number To Decimal String(number=w355) -> (decimal integer string=w354:string)  [unwired: 1 in]
      n123 = call "mDrive Send Command.vi"("error in (no error)"=w356, "Extra"=w354, "Command"=T1."Max Velocity", "VISA resource name"=w357) -> ("error out"=w352:errorcluster, "VISA resource name out"=w362:refnum<visa-resource-name>)  [unwired: 3 in, 1 out]
      n124 = call "mDrive Send Command.vi"("error in (no error)"=w352, "Extra"="VM", "Command"=T1."Print Parameter", "VISA resource name"=w362) -> ("error out"=w359:errorcluster, "read buffer"=w360:string, "VISA resource name out"=w358:refnum<visa-resource-name>)  [unwired: 3 in]
      n125 = Decimal String To Number(string=w360, offset=0) -> (number=w353:i32)  [unwired: 1 in, 1 out]
      n126 = property on="Z  velocity PV step/sec" class="DigNum (strict)"("Val(Sgnl)"=w353) -> ()  [unwired: 2 in, 2 out]
    }
    frame #6 {
      # "PRINT POSITION"
      n127 = call "mDrive Send Command.vi"("error in (no error)"=w368, "Extra"="P", "Command"=T1."Print Parameter", "VISA resource name"=w369) -> ("error out"=w370:errorcluster, "read buffer"=w367:string, "VISA resource name out"=w371:refnum<visa-resource-name>)  [unwired: 3 in]
      n128 = Decimal String To Number(string=w367, offset=0) -> (number=w365:i32)  [unwired: 1 in, 1 out]
    }
    frame #7 {
      n129 = property on="Z Step SP" class="DigNum (strict)"("Val(Sgnl)"=w376) -> ()  [unwired: 2 in, 2 out]
      n130 = property on="Z Step SP" class="DigNum (strict)"() -> ("Maximum"=w373:dbl)  [unwired: 2 in, 2 out]
      n131 = property on="Z Step SP" class="DigNum (strict)"() -> ("Minimum"=w375:dbl)  [unwired: 2 in, 2 out]
      n132 = To Long Integer(number=w373) -> (32bit integer=w374:i32)
      "Z MAXPOS" <- w374
      n133 = To Long Integer(number=w375) -> (32bit integer=w372:i32)
      "Z MINPOS" <- w372
      n134 = In Range and Coerce(upper limit=w374, x=w376, lower limit=w372) -> (In Range?=w377:bool)  [unwired: 1 out]
      n135 = property on="Z in Range" class="Bool (strict)"("Val(Sgnl)"=w377) -> ()  [unwired: 2 in, 2 out]
    }
  }
  n136 = property on="R Step SP" class="DigNum (strict)"("Maximum"=6144000 ("upper limit")) -> ()  [unwired: 2 in, 2 out]
  n137 = property on="R Step SP" class="DigNum (strict)"("Minimum"=-6144000 ("lower limit")) -> ()  [unwired: 2 in, 2 out]
  n138 = property on="V5 position 15360000" class="DigNum (strict)"("Value"=15360000 ("V5 position 15360000")) -> ()  [unwired: 2 in, 2 out]
  n139 = property on="Z Step SP" class="DigNum (strict)"("Maximum"=102400000 ("upper limit")) -> ()  [unwired: 2 in, 2 out]
  n140 = flat-sequence {
    tunnel: [w381] -> w40
    tunnel: [w380] -> w39
    tunnel: [w391] -> w60
    tunnel: [w389] -> w58
    tunnel: w40 -> [w392]
    tunnel: w39 -> [w390]
    tunnel: w60 -> [w396]
    tunnel: [w395] -> w59
    tunnel: w58 -> [w397]
    tunnel: [w399] -> w57
    tunnel: [w408] -> w98
    tunnel: [w410] -> w97
    tunnel: w59 -> [w409]
    tunnel: w57 -> [w411]
    tunnel: w98 -> [w418]
    tunnel: [w417] -> w96
    tunnel: w97 -> [w415]
    tunnel: [w416] -> w95
    tunnel: [w428] -> w94
    tunnel: [w429] -> w93
    tunnel: w96 -> [w427]
    tunnel: w95 -> [w426]
    tunnel: w94 -> [w439]
    tunnel: w93 -> [w438]
    tunnel: [w441] -> w85
    tunnel: [w440] -> w84
    tunnel: [w435] -> w83
    tunnel: [w446] -> w91
    tunnel: [w447] -> w92
    tunnel: w85 -> [w447]
    tunnel: w84 -> [w446]
    tunnel: w83 -> [w442]
    frame #0 {
      w388 = refnum<visa-resource-name> "COM12" ("COM PORT")
      w386 = u16 0 items=["None", "XON/XOFF", "RTS/CTS", "XON/XOFF & RTS/CTS", "DTR/DSR", "XON/XOFF & DTR/DSR"] ("flow control (0:none)")
      w385 = u16 10 items=["1.0"=10, "1.5"=15, "2.0"=20] ("stop bits (10: 1 bit)")
      # "Stop bits"
      n141 = call-poly "VISA Configure Serial Port"("VISA resource name"=w388, "timeout (10sec)"=u32 10000, "baud rate (9600)"=u32 9600, "data bits (8)"=u16 8, "parity (0:none)"=enum16{"None", "Odd", "Even", "Mark", "Space"}."None", "stop bits (10: 1 bit)"=w385, "flow control (0:none)"=w386) -> ("VISA resource name out"=w381:refnum<visa-resource-name>, "error out"=w380:errorcluster)  [unwired: 7 in]
      "X COM PORT" <- w388
    }
    frame #1 {
      n142 = call "mDrive Send Command.vi"("error in (no error)"=w390, "Extra"="EM=2", "Command"=T1."Send String", "VISA resource name"=w392) -> ("error out"=w389:errorcluster, "VISA resource name out"=w391:refnum<visa-resource-name>)  [unwired: 3 in, 1 out]
    }
    frame #2 {
      n143 = Number To Decimal String(number=1000000) -> (decimal integer string=w400:string)  [unwired: 1 in]
      n144 = call "mDrive Send Command.vi"("error in (no error)"=w397, "Extra"=w400, "Command"=T1."Accel Rate", "VISA resource name"=w396) -> ("error out"=w398:errorcluster, "VISA resource name out"=w404:refnum<visa-resource-name>)  [unwired: 3 in, 1 out]
      n145 = call "mDrive Send Command.vi"("error in (no error)"=w398, "Extra"=w400, "Command"=T1."Decel Rate", "VISA resource name"=w404) -> ("error out"=w399:errorcluster, "VISA resource name out"=w395:refnum<visa-resource-name>)  [unwired: 3 in, 1 out]
    }
    frame #3 {
      # "Run Current %"
      n146 = property on="X Run Current %" class="DigNum (strict)"() -> ("Value"=w406:i32)  [unwired: 2 in, 2 out]
      n147 = Number To Decimal String(number=w406) -> (decimal integer string=w407:string)  [unwired: 1 in]
      n148 = call "mDrive Send Command.vi"("error in (no error)"=w411, "Extra"=w407, "Command"=T1."Run Current", "VISA resource name"=w409) -> ("error out"=w410:errorcluster, "VISA resource name out"=w408:refnum<visa-resource-name>)  [unwired: 3 in, 1 out]
    }
    frame #4 {
      # "Holding Current %"
      n149 = property on="X Holding Current %" class="DigNum (strict)"() -> ("Value"=w413:i32)  [unwired: 2 in, 2 out]
      n150 = Number To Decimal String(number=w413) -> (decimal integer string=w414:string)  [unwired: 1 in]
      n151 = call "mDrive Send Command.vi"("error in (no error)"=w415, "Extra"=w414, "Command"=T1."Holding Current", "VISA resource name"=w418) -> ("error out"=w416:errorcluster, "VISA resource name out"=w417:refnum<visa-resource-name>)  [unwired: 3 in, 1 out]
    }
    frame #5 {
      # "Velocity Max"
      n152 = property on="X Velocity SP step/sec" class="DigNum (strict)"() -> ("Value"=w425:i32)  [unwired: 2 in, 2 out]
      n153 = Number To Decimal String(number=w425) -> (decimal integer string=w424:string)  [unwired: 1 in]
      n154 = call "mDrive Send Command.vi"("error in (no error)"=w426, "Extra"=w424, "Command"=T1."Max Velocity", "VISA resource name"=w427) -> ("error out"=w422:errorcluster, "VISA resource name out"=w432:refnum<visa-resource-name>)  [unwired: 3 in, 1 out]
      n155 = call "mDrive Send Command.vi"("error in (no error)"=w422, "Extra"="VM", "Command"=T1."Print Parameter", "VISA resource name"=w432) -> ("error out"=w429:errorcluster, "read buffer"=w430:string, "VISA resource name out"=w428:refnum<visa-resource-name>)  [unwired: 3 in]
      n156 = Decimal String To Number(string=w430, offset=0) -> (number=w423:i32)  [unwired: 1 in, 1 out]
      n157 = property on="X velocity PV step/sec" class="DigNum (strict)"("Val(Sgnl)"=w423) -> ()  [unwired: 2 in, 2 out]
    }
    frame #6 {
      # "PRINT POSITION"
      n158 = call "mDrive Send Command.vi"("error in (no error)"=w438, "Extra"="P", "Command"=T1."Print Parameter", "VISA resource name"=w439) -> ("error out"=w440:errorcluster, "read buffer"=w437:string, "VISA resource name out"=w441:refnum<visa-resource-name>)  [unwired: 3 in]
      n159 = Decimal String To Number(string=w437, offset=0) -> (number=w435:i32)  [unwired: 1 in, 1 out]
    }
    frame #7 {
      w444 = -2304000 ("lower limit")
      w445 = 2304000 ("upper limit")
      n160 = property on="X Step SP" class="DigNum (strict)"("Val(Sgnl)"=w442) -> ()  [unwired: 2 in, 2 out]
      n161 = property on="X Step SP" class="DigNum (strict)"("Maximum"=w445) -> ()  [unwired: 2 in, 2 out]
      n162 = property on="X Step SP" class="DigNum (strict)"("Minimum"=w444) -> ()  [unwired: 2 in, 2 out]
      n163 = In Range and Coerce(upper limit=w445, x=w442, lower limit=w444) -> (In Range?=w443:bool)  [unwired: 1 out]
      n164 = property on="X  in Range" class="Bool (strict)"("Val(Sgnl)"=w443) -> ()  [unwired: 2 in, 2 out]
      "X MINPOS" <- w444
      "X MAXPOS" <- w445
    }
  }
  n165 = call-poly <vilib>:"Read From Spreadsheet File.vi"("file path (dialog if empty)"=path "S:/SSE/IMS/POS.TXT") -> ("first row"=w22:i64[])  [unwired: 6 in, 4 out]
  n166 = call-poly <vilib>:"Read From Spreadsheet File.vi"("file path (dialog if empty)"=path "S:/SSE/IMS/PRESET.TXT") -> ("all rows"=w10:string[][])  [unwired: 6 in, 4 out]
  n167 = Array To Cluster(array=w22) -> (cluster=w21:T3)
  n168 = Transpose 2D Array(2D array=w10) -> (transposed array=w11:string[][])
  n169 = Unbundle(w21) -> ("first row[0]"=w19:i64, "first row[1]"=w18:i64, "first row[2]"=w17:i64, "first row[3]"=w16:i64)  [unwired: 5 out]
  n170 = Delete From Array(array=w11, index (row)=0) -> (deleted portion=w12:string[], array with subset deleted=w14:string[][])  [unwired: 2 in]
  n171 = property on="Reset X Motor Steps" class="DigNum (strict)"("Val(Sgnl)"=w19) -> ()  [unwired: 2 in, 2 out]
  n172 = property on="Reset Y Motor Steps" class="DigNum (strict)"("Val(Sgnl)"=w18) -> ()  [unwired: 2 in, 2 out]
  n173 = property on="Reset Z Motor Steps" class="DigNum (strict)"("Val(Sgnl)"=w17) -> ()  [unwired: 2 in, 2 out]
  n174 = property on="Reset R Motor Steps" class="DigNum (strict)"("Val(Sgnl)"=w16) -> ()  [unwired: 2 in, 2 out]
  n175 = Transpose 2D Array(2D array=w14) -> (transposed array=w15:string[][])
  n176 = property on="Preset positions" class="Ring (strict)"("Strings []"=w12) -> ()  [unwired: 2 in, 2 out]
  n177 = Decimal String To Number(string=w15) -> (number=w13:i32[][])  [unwired: 2 in, 1 out]
  n178 = Initialize Array(w4, w4, 4 ("dimension size")) -> (w7:i32[][])
  n179 = Build Array (concatenate)(w7, w13) -> (→"Presets":i32[][])
  n180 = while {
    tunnel: w106 -> [w470]
    tunnel: w105 -> [w473]
    tunnel: [w474] -> w29
    tunnel: [w472] -> w30
    tunnel: w92 -> [w469]
    tunnel: w91 -> [w468]
    tunnel: [w467] -> w90
    tunnel: [w466] -> w89
    tunnel: w64 -> [w465]
    tunnel: w63 -> [w464]
    tunnel: [w463] -> w32
    tunnel: [w462] -> w31
    tunnel: w62 -> [w461]
    tunnel: w61 -> [w460]
    tunnel: [w459] -> w28
    tunnel: [w458] -> w27
    stop <- "stop" stop-if-true
    n181 = case shown="True" "Submit" {
      tunnel: "ELOG" -> [_ w478]
      frame False {
      }
      frame True {
        n182 = Open/Create/Replace File(file path (use dialog)=path "S:/ELOG/SSE.LOG", operation (0:open)=T4."replace or create") -> (refnum out=w475:refnum<file>)  [unwired: 4 in, 2 out]
        n183 = flat-sequence {
          tunnel: w475 -> [w495]
          tunnel: w478 -> [w482]
          frame #0 {
            n184 = property on="X Position mm PV" class="DigNum (strict)"() -> ("Value"=w492:dbl)  [unwired: 2 in, 2 out]
            n185 = property on="Y Position mm PV" class="DigNum (strict)"() -> ("Value"=w491:dbl)  [unwired: 2 in, 2 out]
            n186 = property on="Z Position mm PV" class="DigNum (strict)"() -> ("Value"=w490:dbl)  [unwired: 2 in, 2 out]
            n187 = property on="R Position deg PV" class="DigNum (strict)"() -> ("Value"=w480:dbl)  [unwired: 2 in, 2 out]
            n188 = Number To Fractional String(number=w492) -> (F-format string=w488:string)  [unwired: 3 in]
            n189 = Number To Fractional String(number=w491) -> (F-format string=w486:string)  [unwired: 3 in]
            n190 = Number To Fractional String(number=w490) -> (F-format string=w484:string)  [unwired: 3 in]
            n191 = Number To Fractional String(number=w480) -> (F-format string=w479:string)  [unwired: 3 in]
            n192 = Concatenate Strings("MX=" ("string"), w488, " MY=" ("string"), w486, " MZ=" ("string"), w484, " MR= " ("string"), w479, " > " ("string"), w482) -> (w494:string)
            n193 = Write to Text File(file (use dialog)=w495, text=w494) -> (refnum out=w493:refnum<file>)  [unwired: 2 in, 2 out]
            n194 = Close File(refnum=w493) -> ()  [unwired: 1 in, 2 out]
          }
          frame #1 {
            n195 = call <vilib>:"System Exec.vi"("working directory"=path "S:/ELOG", "command line"="S:\\elog\\elog.exe -h bl132pc -p 8080 -l \"BL13-2 SSE\" -w beam$2012 -s -a Type=\"Log ES setting\" -a Author=\"Omniax L\" -a Subject=\"Note\" -m SSE.LOG") -> ()  [unwired: 6 in, 4 out]
          }
        }
      }
    }
    n196 = event shown="[0] Timeout" {
      selector: _ -> [_ _ _ _ _ _ _ _ _ _ _ _ _ _ _ _ _ _ _ _ _ _ _ _ _]
      dyn-events: _ -> [_ _ _ _ _ _ _ _ _ _ _ _ _ _ _ _ _ _ _ _ _ _ _ _ _]
      timeout: 100 -> [_ _ _ _ _ _ _ _ _ _ _ _ _ _ _ _ _ _ _ _ _ _ _ _ _]
      tunnel: w473 -> [w600 _ _ _ _ _ _ _ _ _ _ _ w1443 _ _ _ _ w1692 _ _ w1787 w1803 w1847 w1924 w2168]
      tunnel: [w599 _ _ _ _ _ _ _ _ _ _ _ w1449 _ _ _ _ w1690 _ _ w1787 w1801 w1849 w1913 w2166] -> w474
      tunnel: w470 -> [w538 _ _ _ _ _ _ _ _ _ _ _ w1444 _ _ _ _ w1691 _ _ w1788 w1804 w1848 w1926 w2169]
      tunnel: [w598 _ _ _ _ _ _ _ _ _ _ _ w1450 _ _ _ _ w1687 _ _ w1788 w1802 w1850 w1914 w2167] -> w472
      tunnel: w469 -> [w537 _ _ _ _ _ _ _ _ _ _ _ _ _ _ w1601 w1656 _ _ _ _ w1798 w1840 w1930 w2165]
      tunnel: w468 -> [w575 _ _ _ _ _ _ _ _ _ _ _ _ _ _ w1600 w1655 _ _ _ _ w1797 w1839 w1928 w2164]
      tunnel: [w574 _ _ _ _ _ _ _ _ _ _ _ _ _ _ w1599 w1654 _ _ _ _ w1800 w1838 w1906 w2163] -> w467
      tunnel: [w573 _ _ _ _ _ _ _ _ _ _ _ _ _ _ w1598 w1653 _ _ _ _ w1799 w1837 w1904 w2162] -> w466
      tunnel: w465 -> [w547 _ _ _ _ _ _ _ _ _ _ _ _ w1495 _ _ _ _ w1722 _ _ w1796 w1834 w1922 w2161]
      tunnel: w464 -> [w550 _ _ _ _ _ _ _ _ _ _ _ _ w1494 _ _ _ _ w1721 _ _ w1795 w1833 w1920 w2160]
      tunnel: [w549 _ _ _ _ _ _ _ _ _ _ _ _ w1492 _ _ _ _ w1719 _ _ w1794 w1832 w1912 w2157] -> w463
      tunnel: [w548 _ _ _ _ _ _ _ _ _ _ _ _ w1493 _ _ _ _ w1720 _ _ w1793 w1831 w1911 w2156] -> w462
      tunnel: w461 -> [w546 _ _ _ _ _ _ _ _ _ _ _ _ _ w1548 _ _ _ _ w1756 _ w1792 w1828 w1917 w2159]
      tunnel: w460 -> [w545 _ _ _ _ _ _ _ _ _ _ _ _ _ w1547 _ _ _ _ w1755 _ w1791 w1827 w1915 w2158]
      tunnel: [w544 _ _ _ _ _ _ _ _ _ _ _ _ _ w1545 _ _ _ _ w1754 _ w1790 w1826 w1909 w2155] -> w459
      tunnel: [w543 _ _ _ _ _ _ _ _ _ _ _ _ _ w1546 _ _ _ _ w1753 _ w1789 w1825 w1908 w2154] -> w458
      event Timeout {
        n197 = event-data() -> ()  [unwired: 1 in, 2 out]
        n198 = flat-sequence {
          tunnel: [w898] -> w586
          tunnel: [w876] -> w585
          tunnel: [w887] -> w584
          tunnel: [w867] -> w583
          tunnel: w537 -> [w866]
          tunnel: w575 -> [w865]
          tunnel: w586 -> [w904]
          tunnel: [w904] -> w582
          tunnel: w585 -> [w903]
          tunnel: [w903] -> w581
          tunnel: w584 -> [w902]
          tunnel: [w902] -> w580
          tunnel: w583 -> [w899]
          tunnel: [w899] -> w579
          tunnel: w582 -> [w911]
          tunnel: [w912] -> w578
          tunnel: w581 -> [w914]
          tunnel: [w913] -> w577
          tunnel: w580 -> [w910]
          tunnel: [w909] -> w576
          tunnel: w579 -> [w909]
          tunnel: w578 -> [w924]
          tunnel: w577 -> [w925]
          tunnel: w576 -> [w927]
          tunnel: [w923] -> w573
          tunnel: [w922] -> w574
          frame #0 {
            w871 = 0.1 ("Delay Time (s)")
            n199 = property on="X offset mm" class="DigNum (strict)"() -> ("Value"=w881:dbl)  [unwired: 2 in, 2 out]
            n200 = property on="X Step SP" class="DigNum (strict)"() -> ("Maximum"=w889:dbl)  [unwired: 2 in, 2 out]
            n201 = property on="X Step SP" class="DigNum (strict)"() -> ("Minimum"=w891:dbl)  [unwired: 2 in, 2 out]
            n202 = property on="X steps/rev" class="DigNum (strict)"() -> ("Value"=w885:u32)  [unwired: 2 in, 2 out]
            n203 = To Long Integer(number=w889) -> (32bit integer=w888:i32)
            n204 = To Long Integer(number=w891) -> (32bit integer=w890:i32)
            n205 = call "mDrive Send Command.vi"("error in (no error)"=w865, "Extra"="P", "Command"=T1."Print Parameter", "VISA resource name"=w866) -> ("error out"=w893:errorcluster, "read buffer"=w897:string, "VISA resource name out"=w895:refnum<visa-resource-name>)  [unwired: 3 in]
            n206 = call "Time Delay12"("error in (no error)"=w893, "Delay Time (s)"=w871) -> ("error out"=w892:errorcluster)  [unwired: 9 in]
            n207 = Decimal String To Number(string=w897, offset=0) -> (number=w878:i32)  [unwired: 1 in, 1 out]
            n208 = To Double Precision Float(number=w885) -> (double precision float=w886:dbl)
            n209 = To Long Integer(number=w878) -> (32bit integer=w879:i32)
            n210 = property on="X Step PV" class="DigNum (strict)"("Val(Sgnl)"=w879) -> ()  [unwired: 2 in, 2 out]
            n211 = call "mDrive Send Command.vi"("error in (no error)"=w892, "Extra"="MV", "Command"=T1."Print Parameter", "VISA resource name"=w895) -> ("error out"=w894:errorcluster, "read buffer"=w864:string, "VISA resource name out"=w898:refnum<visa-resource-name>)  [unwired: 3 in]
            n212 = call "Time Delay11"("error in (no error)"=w894, "Delay Time (s)"=w871) -> ("error out"=w876:errorcluster)  [unwired: 9 in]
            n213 = In Range and Coerce(upper limit=w888, x=w879, lower limit=w890) -> (In Range?=w887:bool)  [unwired: 1 out]
            n214 = To Double Precision Float(number=w879) -> (double precision float=w880:dbl)
            n215 = Decimal String To Number(string=w864, offset=0 ("offset (0)")) -> (number=w870:i32)  [unwired: 1 in, 1 out]
            n216 = Not Equal?(x=w864, y="") -> (x != y?=w862:bool)
            n217 = property on="X  in Range" class="Bool (strict)"("Val(Sgnl)"=w887) -> ()  [unwired: 2 in, 2 out]
            n218 = property on="X Ready" class="Bool (strict)"("Val(Sgnl)"=w862) -> ()  [unwired: 2 in, 2 out]
            n219 = Divide(x=w880, y=w886) -> (x/y=w884:dbl)
            n220 = Number To Boolean Array(number=w870) -> (Boolean array=w869:bool[])
            n221 = property on="X mm/rev" class="DigNum (strict)"() -> ("Value"=w883:dbl)  [unwired: 2 in, 2 out]
            n222 = Index Array(array=w869, index=0) -> (element=w867:bool)
            n223 = property on="X  in Motion" class="Bool (strict)"("Val(Sgnl)"=w867) -> ()  [unwired: 2 in, 2 out]
            n224 = Multiply(x=w884, y=w883) -> (x*y=w882:dbl)
            n225 = Add(x=w882, y=w881) -> (x+y=w861:dbl)
            n226 = property on="X Position mm PV" class="DigNum (strict)"("Val(Sgnl)"=w861) -> ()  [unwired: 2 in, 2 out]
          }
          frame #1 {
            n227 = property on="X Scan" class="Bool (strict)"() -> ("Value"=w900:bool)  [unwired: 2 in, 2 out]
            n228 = Or(x=w899, y=w900) -> (x .or. y?=w901:bool)
            n229 = case shown="True" w901 {
              frame False {
                n230 = property on="X Scan OK" class="Bool"("DisabledEnum"=T2."Enabled" ("Disabled")) -> ()  [unwired: 2 in, 2 out]
                n231 = property on="X Go" class="Bool"("DisabledEnum"=T2."Enabled" ("Disabled")) -> ()  [unwired: 2 in, 2 out]
              }
              frame True {
                n232 = property on="X Scan OK" class="Bool"("DisabledEnum"=T2."Disabled and Grayed Out" ("Disabled")) -> ()  [unwired: 2 in, 2 out]
                n233 = property on="X Go" class="Bool"("DisabledEnum"=T2."Disabled and Grayed Out" ("Disabled")) -> ()  [unwired: 2 in, 2 out]
              }
            }
          }
          frame #2 {
            n234 = case shown="False" w910 {
              tunnel: w911 -> [w917 w921]
              tunnel: [w918 w921] -> w912
              tunnel: [w919 w920] -> w913
              tunnel: w914 -> [w916 w920]
              frame False {
                n235 = call "mDrive Send Command.vi"("error in (no error)"=w916, "Command"=T1."Stop", "VISA resource name"=w917) -> ("error out"=w919:errorcluster, "VISA resource name out"=w918:refnum<visa-resource-name>)  [unwired: 4 in, 1 out]
              }
              frame True {
              }
            }
          }
          frame #3 {
            n236 = property on="X Backlash corr" class="Bool (strict)"() -> ("Value"=w928:bool)  [unwired: 2 in, 2 out]
            n237 = Implies(1:w927, 2:w928) -> (0:w926:bool)
            n238 = case shown="False" w926 {
              tunnel: w925 -> [w935 w988]
              tunnel: w924 -> [w934 w989]
              tunnel: [w933 w988] -> w923
              tunnel: [w932 w989] -> w922
              frame False {
                # "Backlash"
                n239 = flat-sequence {
                  tunnel: [w950] -> w947
                  tunnel: [w952] -> w946
                  tunnel: [w951] -> w945
                  tunnel: w935 -> [w949]
                  tunnel: w934 -> [w948]
                  tunnel: w947 -> [w960]
                  tunnel: [w960] -> w944
                  tunnel: w946 -> [w959]
                  tunnel: w945 -> [w958]
                  tunnel: [w957] -> w943
                  tunnel: [w956] -> w942
                  tunnel: [w955] -> w931
                  tunnel: w944 -> [w970]
                  tunnel: w943 -> [w969]
                  tunnel: w942 -> [w967]
                  tunnel: [w968] -> w941
                  tunnel: [w967] -> w940
                  tunnel: [w966] -> w937
                  tunnel: [w965] -> w936
                  tunnel: w931 -> [w965]
                  tunnel: w941 -> [w981]
                  tunnel: w940 -> [w974]
                  tunnel: [w981] -> w939
                  tunnel: [w980] -> w938
                  tunnel: w937 -> [w980]
                  tunnel: w936 -> [w976]
                  tunnel: [w975] -> w929
                  tunnel: w939 -> [w985]
                  tunnel: w938 -> [w984]
                  tunnel: [w983] -> w933
                  tunnel: [w982] -> w930
                  tunnel: w929 -> [w982]
                  tunnel: [w987] -> w932
                  tunnel: w930 -> [w987]
                  frame #0 {
                    n240 = property on="X Backlash steps/sec" class="DigNum (strict)"() -> ("Value"=w950:i32)  [unwired: 2 in, 2 out]
                    n241 = Number To Decimal String(number=w950) -> (decimal integer string=w953:string)  [unwired: 1 in]
                    n242 = call "mDrive Send Command.vi"("error in (no error)"=w949, "Extra"=w953, "Command"=T1."Max Velocity", "VISA resource name"=w948) -> ("error out"=w951:errorcluster, "VISA resource name out"=w952:refnum<visa-resource-name>)  [unwired: 3 in, 1 out]
                  }
                  frame #1 {
                    n243 = property on="X Backlash" class="DigNum (strict)"() -> ("Value"=w955:i32)  [unwired: 2 in, 2 out]
                    n244 = Number To Decimal String(number=w955) -> (decimal integer string=w961:string)  [unwired: 1 in]
                    n245 = call "mDrive Send Command.vi"("error in (no error)"=w958, "Extra"=w961, "Command"=T1."Move to Relative Position", "VISA resource name"=w959) -> ("error out"=w957:errorcluster, "VISA resource name out"=w956:refnum<visa-resource-name>)  [unwired: 3 in, 1 out]
                  }
                  frame #2 {
                    n246 = To Double Precision Float(number=w965) -> (double precision float=w963:dbl)
                    n247 = To Double Precision Float(number=w970) -> (double precision float=w972:dbl)
                    n248 = Absolute Value(x=w963) -> (abs(x)=w964:dbl)
                    n249 = Divide(x=w964, y=w972) -> (x/y=w973:dbl)
                    n250 = Add(x=w973, y=0.3) -> (x+y=w966:dbl)
                    n251 = call "Time Delay13"("error in (no error)"=w969, "Delay Time (s)"=w966) -> ("error out"=w968:errorcluster)  [unwired: 9 in]
                  }
                  frame #3 {
                    n252 = Negate(x=w976) -> (-x=w977:i32)
                    n253 = Number To Decimal String(number=w977) -> (decimal integer string=w978:string)  [unwired: 1 in]
                    n254 = call "mDrive Send Command.vi"("Extra"=w978, "Command"=T1."Move to Relative Position", "VISA resource name"=w974) -> ("VISA resource name out"=w975:refnum<visa-resource-name>)  [unwired: 4 in, 2 out]
                  }
                  frame #4 {
                    n255 = call "Time Delay14"("error in (no error)"=w985, "Delay Time (s)"=w984) -> ("error out"=w983:errorcluster)  [unwired: 9 in]
                  }
                  frame #5 {
                    n256 = property on="X Backlash corr" class="Bool (strict)"("Val(Sgnl)"=FALSE ("Value (Signaling)")) -> ()  [unwired: 2 in, 2 out]
                  }
                }
              }
              frame True {
              }
            }
          }
        }
        n257 = flat-sequence {
          tunnel: w600 -> [w1022]
          tunnel: w538 -> [w1021]
          tunnel: [w1027] -> w597
          tunnel: [w1003] -> w595
          tunnel: [w1014] -> w593
          tunnel: [w994] -> w591
          tunnel: w597 -> [w1033]
          tunnel: [w1033] -> w596
          tunnel: w595 -> [w1032]
          tunnel: [w1032] -> w594
          tunnel: w593 -> [w1031]
          tunnel: [w1031] -> w592
          tunnel: w591 -> [w1028]
          tunnel: [w1028] -> w587
          tunnel: w596 -> [w1040]
          tunnel: [w1041] -> w590
          tunnel: w594 -> [w1043]
          tunnel: [w1042] -> w589
          tunnel: w592 -> [w1039]
          tunnel: [w1038] -> w588
          tunnel: w587 -> [w1038]
          tunnel: w590 -> [w1053]
          tunnel: w589 -> [w1054]
          tunnel: w588 -> [w1056]
          tunnel: [w1052] -> w599
          tunnel: [w1051] -> w598
          frame #0 {
            w998 = 0.1 ("Delay Time (s)")
            n258 = property on="Y offset mm" class="DigNum (strict)"() -> ("Value"=w1008:dbl)  [unwired: 2 in, 2 out]
            n259 = property on="Y steps/rev" class="DigNum (strict)"() -> ("Value"=w1012:u32)  [unwired: 2 in, 2 out]
            n260 = property on="Y Step SP" class="DigNum (strict)"() -> ("Maximum"=w1016:dbl)  [unwired: 2 in, 2 out]
            n261 = property on="Y Step SP" class="DigNum (strict)"() -> ("Minimum"=w1018:dbl)  [unwired: 2 in, 2 out]
            n262 = To Long Integer(number=w1016) -> (32bit integer=w1015:i32)
            n263 = To Long Integer(number=w1018) -> (32bit integer=w1017:i32)
            n264 = call "mDrive Send Command.vi"("error in (no error)"=w1022, "Extra"="P", "Command"=T1."Print Parameter", "VISA resource name"=w1021) -> ("error out"=w1020:errorcluster, "read buffer"=w1026:string, "VISA resource name out"=w1024:refnum<visa-resource-name>)  [unwired: 3 in]
            n265 = call "Time Delay4"("error in (no error)"=w1020, "Delay Time (s)"=w998) -> ("error out"=w1019:errorcluster)  [unwired: 9 in]
            n266 = Decimal String To Number(string=w1026, offset=0) -> (number=w1005:i32)  [unwired: 1 in, 1 out]
            n267 = To Double Precision Float(number=w1012) -> (double precision float=w1013:dbl)
            n268 = To Long Integer(number=w1005) -> (32bit integer=w1006:i32)
            n269 = property on="Y Step PV" class="DigNum (strict)"("Val(Sgnl)"=w1006) -> ()  [unwired: 2 in, 2 out]
            n270 = call "mDrive Send Command.vi"("error in (no error)"=w1019, "Extra"="MV", "Command"=T1."Print Parameter", "VISA resource name"=w1024) -> ("error out"=w1023:errorcluster, "read buffer"=w991:string, "VISA resource name out"=w1027:refnum<visa-resource-name>)  [unwired: 3 in]
            n271 = call "Time Delay3"("error in (no error)"=w1023, "Delay Time (s)"=w998) -> ("error out"=w1003:errorcluster)  [unwired: 9 in]
            n272 = In Range and Coerce(upper limit=w1015, x=w1006, lower limit=w1017) -> (In Range?=w1014:bool)  [unwired: 1 out]
            n273 = To Double Precision Float(number=w1006) -> (double precision float=w1007:dbl)
            n274 = Decimal String To Number(string=w991, offset=0 ("offset (0)")) -> (number=w997:i32)  [unwired: 1 in, 1 out]
            n275 = Not Equal?(x=w991, y="") -> (x != y?=w992:bool)
            n276 = property on="Y in Range" class="Bool (strict)"("Val(Sgnl)"=w1014) -> ()  [unwired: 2 in, 2 out]
            n277 = property on="Y Ready" class="Bool (strict)"("Val(Sgnl)"=w992) -> ()  [unwired: 2 in, 2 out]
            n278 = Divide(x=w1007, y=w1013) -> (x/y=w1011:dbl)
            n279 = Number To Boolean Array(number=w997) -> (Boolean array=w996:bool[])
            n280 = property on="Y mm/rev" class="DigNum (strict)"() -> ("Value"=w1010:dbl)  [unwired: 2 in, 2 out]
            n281 = Index Array(array=w996, index=0) -> (element=w994:bool)
            n282 = property on="Y in Motion" class="Bool (strict)"("Val(Sgnl)"=w994) -> ()  [unwired: 2 in, 2 out]
            n283 = Multiply(x=w1011, y=w1010) -> (x*y=w1009:dbl)
            n284 = Add(x=w1009, y=w1008) -> (x+y=w990:dbl)
            n285 = property on="Y Position mm PV" class="DigNum (strict)"("Val(Sgnl)"=w990) -> ()  [unwired: 2 in, 2 out]
          }
          frame #1 {
            n286 = property on="Y Scan" class="Bool (strict)"() -> ("Value"=w1029:bool)  [unwired: 2 in, 2 out]
            n287 = Or(x=w1028, y=w1029) -> (x .or. y?=w1030:bool)
            n288 = case shown="True" w1030 {
              frame False {
                n289 = property on="Y Scan OK" class="Bool"("DisabledEnum"=T2."Enabled" ("Disabled")) -> ()  [unwired: 2 in, 2 out]
                n290 = property on="Y Go" class="Bool"("DisabledEnum"=T2."Enabled" ("Disabled")) -> ()  [unwired: 2 in, 2 out]
              }
              frame True {
                n291 = property on="Y Scan OK" class="Bool"("DisabledEnum"=T2."Disabled and Grayed Out" ("Disabled")) -> ()  [unwired: 2 in, 2 out]
                n292 = property on="Y Go" class="Bool"("DisabledEnum"=T2."Disabled and Grayed Out" ("Disabled")) -> ()  [unwired: 2 in, 2 out]
              }
            }
          }
          frame #2 {
            n293 = case shown="False" w1039 {
              tunnel: w1040 -> [w1046 w1050]
              tunnel: [w1047 w1050] -> w1041
              tunnel: [w1048 w1049] -> w1042
              tunnel: w1043 -> [w1045 w1049]
              frame False {
                n294 = call "mDrive Send Command.vi"("error in (no error)"=w1045, "Command"=T1."Stop", "VISA resource name"=w1046) -> ("error out"=w1048:errorcluster, "VISA resource name out"=w1047:refnum<visa-resource-name>)  [unwired: 4 in, 1 out]
              }
              frame True {
              }
            }
          }
          frame #3 {
            n295 = property on="Y Backlash corr" class="Bool (strict)"() -> ("Value"=w1057:bool)  [unwired: 2 in, 2 out]
            n296 = Implies(1:w1056, 2:w1057) -> (0:w1055:bool)
            n297 = case shown="False" w1055 {
              tunnel: w1054 -> [w1064 w1117]
              tunnel: w1053 -> [w1063 w1118]
              tunnel: [w1062 w1117] -> w1052
              tunnel: [w1061 w1118] -> w1051
              frame False {
                # "Backlash"
                n298 = flat-sequence {
                  tunnel: [w1079] -> w1076
                  tunnel: [w1081] -> w1075
                  tunnel: [w1080] -> w1074
                  tunnel: w1064 -> [w1078]
                  tunnel: w1063 -> [w1077]
                  tunnel: w1076 -> [w1089]
                  tunnel: [w1089] -> w1073
                  tunnel: w1075 -> [w1088]
                  tunnel: w1074 -> [w1087]
                  tunnel: [w1086] -> w1072
                  tunnel: [w1085] -> w1071
                  tunnel: [w1084] -> w1060
                  tunnel: w1073 -> [w1099]
                  tunnel: w1072 -> [w1098]
                  tunnel: w1071 -> [w1096]
                  tunnel: [w1097] -> w1070
                  tunnel: [w1096] -> w1069
                  tunnel: [w1095] -> w1066
                  tunnel: [w1094] -> w1065
                  tunnel: w1060 -> [w1094]
                  tunnel: w1070 -> [w1110]
                  tunnel: w1069 -> [w1103]
                  tunnel: [w1110] -> w1068
                  tunnel: [w1109] -> w1067
                  tunnel: w1066 -> [w1109]
                  tunnel: w1065 -> [w1105]
                  tunnel: [w1104] -> w1058
                  tunnel: w1068 -> [w1114]
                  tunnel: w1067 -> [w1113]
                  tunnel: [w1112] -> w1062
                  tunnel: [w1111] -> w1059
                  tunnel: w1058 -> [w1111]
                  tunnel: [w1116] -> w1061
                  tunnel: w1059 -> [w1116]
                  frame #0 {
                    n299 = property on="Y Backlash steps/sec" class="DigNum (strict)"() -> ("Value"=w1079:i32)  [unwired: 2 in, 2 out]
                    n300 = Number To Decimal String(number=w1079) -> (decimal integer string=w1082:string)  [unwired: 1 in]
                    n301 = call "mDrive Send Command.vi"("error in (no error)"=w1078, "Extra"=w1082, "Command"=T1."Max Velocity", "VISA resource name"=w1077) -> ("error out"=w1080:errorcluster, "VISA resource name out"=w1081:refnum<visa-resource-name>)  [unwired: 3 in, 1 out]
                  }
                  frame #1 {
                    n302 = property on="Y Backlash" class="DigNum (strict)"() -> ("Value"=w1084:i32)  [unwired: 2 in, 2 out]
                    n303 = Number To Decimal String(number=w1084) -> (decimal integer string=w1090:string)  [unwired: 1 in]
                    n304 = call "mDrive Send Command.vi"("error in (no error)"=w1087, "Extra"=w1090, "Command"=T1."Move to Relative Position", "VISA resource name"=w1088) -> ("error out"=w1086:errorcluster, "VISA resource name out"=w1085:refnum<visa-resource-name>)  [unwired: 3 in, 1 out]
                  }
                  frame #2 {
                    n305 = To Double Precision Float(number=w1094) -> (double precision float=w1092:dbl)
                    n306 = To Double Precision Float(number=w1099) -> (double precision float=w1101:dbl)
                    n307 = Absolute Value(x=w1092) -> (abs(x)=w1093:dbl)
                    n308 = Divide(x=w1093, y=w1101) -> (x/y=w1102:dbl)
                    n309 = Add(x=w1102, y=0.3) -> (x+y=w1095:dbl)
                    n310 = call "Time Delay8"("error in (no error)"=w1098, "Delay Time (s)"=w1095) -> ("error out"=w1097:errorcluster)  [unwired: 9 in]
                  }
                  frame #3 {
                    n311 = Negate(x=w1105) -> (-x=w1106:i32)
                    n312 = Number To Decimal String(number=w1106) -> (decimal integer string=w1107:string)  [unwired: 1 in]
                    n313 = call "mDrive Send Command.vi"("Extra"=w1107, "Command"=T1."Move to Relative Position", "VISA resource name"=w1103) -> ("VISA resource name out"=w1104:refnum<visa-resource-name>)  [unwired: 4 in, 2 out]
                  }
                  frame #4 {
                    n314 = call "Time Delay2"("error in (no error)"=w1114, "Delay Time (s)"=w1113) -> ("error out"=w1112:errorcluster)  [unwired: 9 in]
                  }
                  frame #5 {
                    n315 = property on="Y Backlash corr" class="Bool (strict)"("Val(Sgnl)"=FALSE ("Value (Signaling)")) -> ()  [unwired: 2 in, 2 out]
                  }
                }
              }
              frame True {
              }
            }
          }
        }
        n316 = flat-sequence {
          tunnel: [w769] -> w572
          tunnel: [w748] -> w571
          tunnel: [w759] -> w570
          tunnel: [w739] -> w569
          tunnel: w547 -> [w738]
          tunnel: w550 -> [w737]
          tunnel: w572 -> [w775]
          tunnel: [w775] -> w568
          tunnel: w571 -> [w774]
          tunnel: [w774] -> w567
          tunnel: w570 -> [w773]
          tunnel: [w773] -> w566
          tunnel: w569 -> [w770]
          tunnel: [w770] -> w565
          tunnel: w568 -> [w782]
          tunnel: [w783] -> w564
          tunnel: w567 -> [w785]
          tunnel: [w784] -> w563
          tunnel: w566 -> [w781]
          tunnel: [w780] -> w562
          tunnel: w565 -> [w780]
          tunnel: w564 -> [w795]
          tunnel: w563 -> [w796]
          tunnel: w562 -> [w798]
          tunnel: [w794] -> w548
          tunnel: [w793] -> w549
          frame #0 {
            w743 = 0.1 ("Delay Time (s)")
            n317 = property on="Z Step SP" class="DigNum (strict)" props=["Maximum"]() -> ()  [unwired: 2 in, 3 out]
            n318 = property on="Z offset mm" class="DigNum (strict)"() -> ("Value"=w753:dbl)  [unwired: 2 in, 2 out]
            n319 = property on="Z steps/rev" class="DigNum (strict)"() -> ("Value"=w757:u32)  [unwired: 2 in, 2 out]
            n320 = property on="Z Step SP" class="DigNum (strict)"() -> ("Minimum"=w762:dbl)  [unwired: 2 in, 2 out]
            n321 = property on="Z max step" class="DigNum (strict)"() -> ("Value"=w733:i32)  [unwired: 2 in, 2 out]
            n322 = To Long Integer(number=w733) -> (32bit integer=w760:i32)
            n323 = To Long Integer(number=w762) -> (32bit integer=w761:i32)
            n324 = call "mDrive Send Command.vi"("error in (no error)"=w737, "Extra"="P", "Command"=T1."Print Parameter", "VISA resource name"=w738) -> ("error out"=w764:errorcluster, "read buffer"=w768:string, "VISA resource name out"=w766:refnum<visa-resource-name>)  [unwired: 3 in]
            n325 = call "Time Delay17"("error in (no error)"=w764, "Delay Time (s)"=w743) -> ("error out"=w763:errorcluster)  [unwired: 9 in]
            n326 = Decimal String To Number(string=w768, offset=0) -> (number=w750:i32)  [unwired: 1 in, 1 out]
            n327 = To Double Precision Float(number=w757) -> (double precision float=w758:dbl)
            n328 = To Long Integer(number=w750) -> (32bit integer=w751:i32)
            n329 = property on="Z Step PV" class="DigNum (strict)"("Val(Sgnl)"=w751) -> ()  [unwired: 2 in, 2 out]
            n330 = call "mDrive Send Command.vi"("error in (no error)"=w763, "Extra"="MV", "Command"=T1."Print Parameter", "VISA resource name"=w766) -> ("error out"=w765:errorcluster, "read buffer"=w734:string, "VISA resource name out"=w769:refnum<visa-resource-name>)  [unwired: 3 in]
            n331 = call "Time Delay16"("error in (no error)"=w765, "Delay Time (s)"=w743) -> ("error out"=w748:errorcluster)  [unwired: 9 in]
            n332 = In Range and Coerce(upper limit=w760, x=w751, lower limit=w761) -> (In Range?=w759:bool)  [unwired: 1 out]
            n333 = To Double Precision Float(number=w751) -> (double precision float=w752:dbl)
            n334 = Decimal String To Number(string=w734, offset=0 ("offset (0)")) -> (number=w742:i32)  [unwired: 1 in, 1 out]
            n335 = Not Equal?(x=w734, y="") -> (x != y?=w735:bool)
            n336 = property on="Z in Range" class="Bool (strict)"("Val(Sgnl)"=w759) -> ()  [unwired: 2 in, 2 out]
            n337 = property on="Z Ready" class="Bool (strict)"("Val(Sgnl)"=w735) -> ()  [unwired: 2 in, 2 out]
            n338 = Divide(x=w752, y=w758) -> (x/y=w756:dbl)
            n339 = Number To Boolean Array(number=w742) -> (Boolean array=w741:bool[])
            n340 = property on="Z mm/rev" class="DigNum (strict)"() -> ("Value"=w755:dbl)  [unwired: 2 in, 2 out]
            n341 = Index Array(array=w741, index=0) -> (element=w739:bool)
            n342 = property on="Z in Motion" class="Bool (strict)"("Val(Sgnl)"=w739) -> ()  [unwired: 2 in, 2 out]
            n343 = Multiply(x=w756, y=w755) -> (x*y=w754:dbl)
            n344 = Add(x=w754, y=w753) -> (x+y=w732:dbl)
            n345 = property on="Z Position mm PV" class="DigNum (strict)"("Val(Sgnl)"=w732) -> ()  [unwired: 2 in, 2 out]
          }
          frame #1 {
            n346 = property on="Z Scan" class="Bool (strict)"() -> ("Value"=w771:bool)  [unwired: 2 in, 2 out]
            n347 = Or(x=w770, y=w771) -> (x .or. y?=w772:bool)
            n348 = case shown="True" w772 {
              frame False {
                n349 = property on="Z Scan OK" class="Bool"("DisabledEnum"=T2."Enabled" ("Disabled")) -> ()  [unwired: 2 in, 2 out]
                n350 = property on="Z Go" class="Bool"("DisabledEnum"=T2."Enabled" ("Disabled")) -> ()  [unwired: 2 in, 2 out]
              }
              frame True {
                n351 = property on="Z Scan OK" class="Bool"("DisabledEnum"=T2."Disabled and Grayed Out" ("Disabled")) -> ()  [unwired: 2 in, 2 out]
                n352 = property on="Z Go" class="Bool"("DisabledEnum"=T2."Disabled and Grayed Out" ("Disabled")) -> ()  [unwired: 2 in, 2 out]
              }
            }
          }
          frame #2 {
            n353 = case shown="False" w781 {
              tunnel: w782 -> [w788 w792]
              tunnel: [w789 w792] -> w783
              tunnel: [w790 w791] -> w784
              tunnel: w785 -> [w787 w791]
              frame False {
                n354 = call "mDrive Send Command.vi"("error in (no error)"=w787, "Command"=T1."Stop", "VISA resource name"=w788) -> ("error out"=w790:errorcluster, "VISA resource name out"=w789:refnum<visa-resource-name>)  [unwired: 4 in, 1 out]
              }
              frame True {
              }
            }
          }
          frame #3 {
            n355 = property on="Z Backlash corr" class="Bool (strict)"() -> ("Value"=w799:bool)  [unwired: 2 in, 2 out]
            n356 = Implies(1:w798, 2:w799) -> (0:w797:bool)
            n357 = case shown="False" w797 {
              tunnel: w796 -> [w806 w859]
              tunnel: w795 -> [w805 w860]
              tunnel: [w804 w859] -> w794
              tunnel: [w803 w860] -> w793
              frame False {
                # "Backlash"
                n358 = flat-sequence {
                  tunnel: [w821] -> w818
                  tunnel: [w823] -> w817
                  tunnel: [w822] -> w816
                  tunnel: w806 -> [w820]
                  tunnel: w805 -> [w819]
                  tunnel: w818 -> [w831]
                  tunnel: [w831] -> w815
                  tunnel: w817 -> [w830]
                  tunnel: w816 -> [w829]
                  tunnel: [w828] -> w814
                  tunnel: [w827] -> w813
                  tunnel: [w826] -> w802
                  tunnel: w815 -> [w841]
                  tunnel: w814 -> [w840]
                  tunnel: w813 -> [w838]
                  tunnel: [w839] -> w812
                  tunnel: [w838] -> w811
                  tunnel: [w837] -> w808
                  tunnel: [w836] -> w807
                  tunnel: w802 -> [w836]
                  tunnel: w812 -> [w852]
                  tunnel: w811 -> [w845]
                  tunnel: [w852] -> w810
                  tunnel: [w851] -> w809
                  tunnel: w808 -> [w851]
                  tunnel: w807 -> [w847]
                  tunnel: [w846] -> w800
                  tunnel: w810 -> [w856]
                  tunnel: w809 -> [w855]
                  tunnel: [w854] -> w804
                  tunnel: [w853] -> w801
                  tunnel: w800 -> [w853]
                  tunnel: [w858] -> w803
                  tunnel: w801 -> [w858]
                  frame #0 {
                    n359 = property on="Z Backlash steps/sec" class="DigNum (strict)"() -> ("Value"=w821:i32)  [unwired: 2 in, 2 out]
                    n360 = Number To Decimal String(number=w821) -> (decimal integer string=w824:string)  [unwired: 1 in]
                    n361 = call "mDrive Send Command.vi"("error in (no error)"=w820, "Extra"=w824, "Command"=T1."Max Velocity", "VISA resource name"=w819) -> ("error out"=w822:errorcluster, "VISA resource name out"=w823:refnum<visa-resource-name>)  [unwired: 3 in, 1 out]
                  }
                  frame #1 {
                    n362 = property on="Z Backlash" class="DigNum (strict)"() -> ("Value"=w826:i32)  [unwired: 2 in, 2 out]
                    n363 = Number To Decimal String(number=w826) -> (decimal integer string=w832:string)  [unwired: 1 in]
                    n364 = call "mDrive Send Command.vi"("error in (no error)"=w829, "Extra"=w832, "Command"=T1."Move to Relative Position", "VISA resource name"=w830) -> ("error out"=w828:errorcluster, "VISA resource name out"=w827:refnum<visa-resource-name>)  [unwired: 3 in, 1 out]
                  }
                  frame #2 {
                    n365 = To Double Precision Float(number=w836) -> (double precision float=w834:dbl)
                    n366 = To Double Precision Float(number=w841) -> (double precision float=w843:dbl)
                    n367 = Absolute Value(x=w834) -> (abs(x)=w835:dbl)
                    n368 = Divide(x=w835, y=w843) -> (x/y=w844:dbl)
                    n369 = Add(x=w844, y=0.5) -> (x+y=w837:dbl)
                    n370 = call "Time Delay18"("error in (no error)"=w840, "Delay Time (s)"=w837) -> ("error out"=w839:errorcluster)  [unwired: 9 in]
                  }
                  frame #3 {
                    n371 = Negate(x=w847) -> (-x=w848:i32)
                    n372 = Number To Decimal String(number=w848) -> (decimal integer string=w849:string)  [unwired: 1 in]
                    n373 = call "mDrive Send Command.vi"("Extra"=w849, "Command"=T1."Move to Relative Position", "VISA resource name"=w845) -> ("VISA resource name out"=w846:refnum<visa-resource-name>)  [unwired: 4 in, 2 out]
                  }
                  frame #4 {
                    n374 = call "Time Delay19"("error in (no error)"=w856, "Delay Time (s)"=w855) -> ("error out"=w854:errorcluster)  [unwired: 9 in]
                  }
                  frame #5 {
                    n375 = property on="Z Backlash corr" class="Bool (strict)"("Val(Sgnl)"=FALSE ("Value (Signaling)")) -> ()  [unwired: 2 in, 2 out]
                  }
                }
              }
              frame True {
              }
            }
          }
        }
        n376 = flat-sequence {
          tunnel: [w640] -> w561
          tunnel: [w618] -> w560
          tunnel: [w629] -> w559
          tunnel: [w609] -> w558
          tunnel: w546 -> [w608]
          tunnel: w545 -> [w607]
          tunnel: w561 -> [w646]
          tunnel: [w646] -> w557
          tunnel: w560 -> [w645]
          tunnel: [w645] -> w556
          tunnel: w559 -> [w644]
          tunnel: [w644] -> w555
          tunnel: w558 -> [w641]
          tunnel: [w641] -> w554
          tunnel: w557 -> [w653]
          tunnel: [w654] -> w553
          tunnel: w556 -> [w656]
          tunnel: [w655] -> w552
          tunnel: w555 -> [w652]
          tunnel: [w651] -> w551
          tunnel: w554 -> [w651]
          tunnel: w553 -> [w666]
          tunnel: w552 -> [w667]
          tunnel: w551 -> [w669]
          tunnel: [w665] -> w543
          tunnel: [w664] -> w544
          frame #0 {
            w613 = 0.1 ("Delay Time (s)")
            n377 = property on="R offset deg" class="DigNum (strict)"() -> ("Value"=w623:dbl)  [unwired: 2 in, 2 out]
            n378 = property on="R steps/rev" class="DigNum (strict)"() -> ("Value"=w627:u32)  [unwired: 2 in, 2 out]
            n379 = property on="R Step SP" class="DigNum (strict)"() -> ("Maximum"=w631:dbl)  [unwired: 2 in, 2 out]
            n380 = property on="R Step SP" class="DigNum (strict)"() -> ("Minimum"=w633:dbl)  [unwired: 2 in, 2 out]
            n381 = To Long Integer(number=w631) -> (32bit integer=w630:i32)
            n382 = To Long Integer(number=w633) -> (32bit integer=w632:i32)
            n383 = call "mDrive Send Command.vi"("error in (no error)"=w607, "Extra"="P", "Command"=T1."Print Parameter", "VISA resource name"=w608) -> ("error out"=w635:errorcluster, "read buffer"=w639:string, "VISA resource name out"=w637:refnum<visa-resource-name>)  [unwired: 3 in]
            n384 = call "Time Delay21"("error in (no error)"=w635, "Delay Time (s)"=w613) -> ("error out"=w634:errorcluster)  [unwired: 9 in]
            n385 = Decimal String To Number(string=w639, offset=0) -> (number=w620:i32)  [unwired: 1 in, 1 out]
            n386 = To Double Precision Float(number=w627) -> (double precision float=w628:dbl)
            n387 = To Long Integer(number=w620) -> (32bit integer=w621:i32)
            n388 = property on="R Step PV" class="DigNum (strict)"("Val(Sgnl)"=w621) -> ()  [unwired: 2 in, 2 out]
            n389 = call "mDrive Send Command.vi"("error in (no error)"=w634, "Extra"="MV", "Command"=T1."Print Parameter", "VISA resource name"=w637) -> ("error out"=w636:errorcluster, "read buffer"=w604:string, "VISA resource name out"=w640:refnum<visa-resource-name>)  [unwired: 3 in]
            n390 = call "Time Delay20"("error in (no error)"=w636, "Delay Time (s)"=w613) -> ("error out"=w618:errorcluster)  [unwired: 9 in]
            n391 = In Range and Coerce(upper limit=w630, x=w621, lower limit=w632) -> (In Range?=w629:bool)  [unwired: 1 out]
            n392 = To Double Precision Float(number=w621) -> (double precision float=w622:dbl)
            n393 = Decimal String To Number(string=w604, offset=0 ("offset (0)")) -> (number=w612:i32)  [unwired: 1 in, 1 out]
            n394 = Not Equal?(x=w604, y="") -> (x != y?=w605:bool)
            n395 = property on="R in Range" class="Bool (strict)"("Val(Sgnl)"=w629) -> ()  [unwired: 2 in, 2 out]
            n396 = property on="R Ready" class="Bool (strict)"("Val(Sgnl)"=w605) -> ()  [unwired: 2 in, 2 out]
            n397 = Divide(x=w622, y=w628) -> (x/y=w626:dbl)
            n398 = Number To Boolean Array(number=w612) -> (Boolean array=w611:bool[])
            n399 = property on="R deg/rev" class="DigNum (strict)"() -> ("Value"=w625:dbl)  [unwired: 2 in, 2 out]
            n400 = Index Array(array=w611, index=0) -> (element=w609:bool)
            n401 = property on="R in Motion" class="Bool (strict)"("Val(Sgnl)"=w609) -> ()  [unwired: 2 in, 2 out]
            n402 = Multiply(x=w626, y=w625) -> (x*y=w624:dbl)
            n403 = Add(x=w624, y=w623) -> (x+y=w603:dbl)
            n404 = property on="R Position deg PV" class="DigNum (strict)"("Val(Sgnl)"=w603) -> ()  [unwired: 2 in, 2 out]
          }
          frame #1 {
            n405 = property on="R Scan" class="Bool (strict)"() -> ("Value"=w642:bool)  [unwired: 2 in, 2 out]
            n406 = Or(x=w641, y=w642) -> (x .or. y?=w643:bool)
            n407 = case shown="True" w643 {
              frame False {
                n408 = property on="R Scan OK" class="Bool"("DisabledEnum"=T2."Enabled" ("Disabled")) -> ()  [unwired: 2 in, 2 out]
                n409 = property on="R Go" class="Bool"("DisabledEnum"=T2."Enabled" ("Disabled")) -> ()  [unwired: 2 in, 2 out]
              }
              frame True {
                n410 = property on="R Scan OK" class="Bool"("DisabledEnum"=T2."Disabled and Grayed Out" ("Disabled")) -> ()  [unwired: 2 in, 2 out]
                n411 = property on="R Go" class="Bool"("DisabledEnum"=T2."Disabled and Grayed Out" ("Disabled")) -> ()  [unwired: 2 in, 2 out]
              }
            }
          }
          frame #2 {
            n412 = case shown="False" w652 {
              tunnel: w653 -> [w659 w663]
              tunnel: [w660 w663] -> w654
              tunnel: [w661 w662] -> w655
              tunnel: w656 -> [w658 w662]
              frame False {
                n413 = call "mDrive Send Command.vi"("error in (no error)"=w658, "Command"=T1."Stop", "VISA resource name"=w659) -> ("error out"=w661:errorcluster, "VISA resource name out"=w660:refnum<visa-resource-name>)  [unwired: 4 in, 1 out]
              }
              frame True {
              }
            }
          }
          frame #3 {
            n414 = property on="R Backlash corr" class="Bool (strict)"() -> ("Value"=w670:bool)  [unwired: 2 in, 2 out]
            n415 = Implies(1:w669, 2:w670) -> (0:w668:bool)
            n416 = case shown="False" w668 {
              tunnel: w667 -> [w677 w730]
              tunnel: w666 -> [w676 w731]
              tunnel: [w675 w730] -> w665
              tunnel: [w674 w731] -> w664
              frame False {
                # "Backlash"
                n417 = flat-sequence {
                  tunnel: [w692] -> w689
                  tunnel: [w694] -> w688
                  tunnel: [w693] -> w687
                  tunnel: w677 -> [w691]
                  tunnel: w676 -> [w690]
                  tunnel: w689 -> [w702]
                  tunnel: [w702] -> w686
                  tunnel: w688 -> [w701]
                  tunnel: w687 -> [w700]
                  tunnel: [w699] -> w685
                  tunnel: [w698] -> w684
                  tunnel: [w697] -> w673
                  tunnel: w686 -> [w712]
                  tunnel: w685 -> [w711]
                  tunnel: w684 -> [w709]
                  tunnel: [w710] -> w683
                  tunnel: [w709] -> w682
                  tunnel: [w708] -> w679
                  tunnel: [w707] -> w678
                  tunnel: w673 -> [w707]
                  tunnel: w683 -> [w723]
                  tunnel: w682 -> [w716]
                  tunnel: [w723] -> w681
                  tunnel: [w722] -> w680
                  tunnel: w679 -> [w722]
                  tunnel: w678 -> [w718]
                  tunnel: [w717] -> w671
                  tunnel: w681 -> [w727]
                  tunnel: w680 -> [w726]
                  tunnel: [w725] -> w675
                  tunnel: [w724] -> w672
                  tunnel: w671 -> [w724]
                  tunnel: [w729] -> w674
                  tunnel: w672 -> [w729]
                  frame #0 {
                    n418 = property on="R Backlash steps/sec" class="DigNum (strict)"() -> ("Value"=w692:i32)  [unwired: 2 in, 2 out]
                    n419 = Number To Decimal String(number=w692) -> (decimal integer string=w695:string)  [unwired: 1 in]
                    n420 = call "mDrive Send Command.vi"("error in (no error)"=w691, "Extra"=w695, "Command"=T1."Max Velocity", "VISA resource name"=w690) -> ("error out"=w693:errorcluster, "VISA resource name out"=w694:refnum<visa-resource-name>)  [unwired: 3 in, 1 out]
                  }
                  frame #1 {
                    n421 = property on="R Backlash" class="DigNum (strict)"() -> ("Value"=w697:i32)  [unwired: 2 in, 2 out]
                    n422 = Number To Decimal String(number=w697) -> (decimal integer string=w703:string)  [unwired: 1 in]
                    n423 = call "mDrive Send Command.vi"("error in (no error)"=w700, "Extra"=w703, "Command"=T1."Move to Relative Position", "VISA resource name"=w701) -> ("error out"=w699:errorcluster, "VISA resource name out"=w698:refnum<visa-resource-name>)  [unwired: 3 in, 1 out]
                  }
                  frame #2 {
                    n424 = To Double Precision Float(number=w707) -> (double precision float=w705:dbl)
                    n425 = To Double Precision Float(number=w712) -> (double precision float=w714:dbl)
                    n426 = Absolute Value(x=w705) -> (abs(x)=w706:dbl)
                    n427 = Divide(x=w706, y=w714) -> (x/y=w715:dbl)
                    n428 = Add(x=w715, y=0.3) -> (x+y=w708:dbl)
                    n429 = call "Time Delay22"("error in (no error)"=w711, "Delay Time (s)"=w708) -> ("error out"=w710:errorcluster)  [unwired: 9 in]
                  }
                  frame #3 {
                    n430 = Negate(x=w718) -> (-x=w719:i32)
                    n431 = Number To Decimal String(number=w719) -> (decimal integer string=w720:string)  [unwired: 1 in]
                    n432 = call "mDrive Send Command.vi"("Extra"=w720, "Command"=T1."Move to Relative Position", "VISA resource name"=w716) -> ("VISA resource name out"=w717:refnum<visa-resource-name>)  [unwired: 4 in, 2 out]
                  }
                  frame #4 {
                    n433 = call "Time Delay23"("error in (no error)"=w727, "Delay Time (s)"=w726) -> ("error out"=w725:errorcluster)  [unwired: 9 in]
                  }
                  frame #5 {
                    n434 = property on="R Backlash corr" class="Bool (strict)"("Val(Sgnl)"=FALSE ("Value (Signaling)")) -> ()  [unwired: 2 in, 2 out]
                  }
                }
              }
              frame True {
              }
            }
          }
        }
        n435 = property on="IV5OP" class="Bool (strict)"() -> ("Value"=w522:bool)  [unwired: 2 in, 2 out]
        n436 = case shown="False" w522 {
          tunnel: [w601 w602] -> w521
          frame False {
            n437 = property on="V5 position 15360000" class="DigNum (strict)"() -> ("Value"=w601:i32)  [unwired: 2 in, 2 out]
          }
          frame True {
            n438 = property on="Z Step SP" class="DigNum (strict)"() -> ("Maximum"=w602:dbl)  [unwired: 2 in, 2 out]
          }
        }
        "Z max step" <- w521
        n439 = property on="Y Scan Length SP steps" class="DigNum (strict)"() -> ("Value"=w524:i32)  [unwired: 2 in, 2 out]
        n440 = property on="Z Scan Length SP steps" class="DigNum (strict)"() -> ("Value"=w525:i32)  [unwired: 2 in, 2 out]
        n441 = property on="Z Position mm PV" class="DigNum (strict)"() -> ("Value"=w533:dbl)  [unwired: 2 in, 2 out]
        n442 = property on="Y Position mm PV" class="DigNum (strict)"() -> ("Value"=w532:dbl)  [unwired: 2 in, 2 out]
        n443 = property on="X Position mm PV" class="DigNum (strict)"() -> ("Value"=w539:dbl)  [unwired: 2 in, 2 out]
        n444 = property on="R Position deg PV" class="DigNum (strict)"() -> ("Value"=w540:dbl)  [unwired: 2 in, 2 out]
        n445 = Divide(x=w524, y=w525) -> (x/y=w526:dbl)
        n446 = call "Build XY Graph2"("Reset"=TRUE, "Y Input"=w540, "X Input"=w533) -> ("XY Graph"=→"ZR Graph":cluster{"Y":dbl[], "Y":dbl[]}[])  [unwired: 7 in, 1 out]
        n447 = call "Build XY Graph"("Reset"=TRUE, "Y Input"=w532, "X Input"=w539) -> ("XY Graph"=→"XY Graph":cluster{"Y":dbl[], "Y":dbl[]}[])  [unwired: 7 in, 1 out]
        n448 = property on="Clear ZY" class="Bool (strict)"() -> ("Value"=w523:bool)  [unwired: 2 in, 2 out]
        n449 = call "Build XY Graph3"("Reset"=w523, "Y Input"=w532, "X Input"=w533) -> ("XY Graph"=→"ZY Graph":cluster{"Y":dbl[], "Y":dbl[]}[])  [unwired: 7 in, 1 out]
        n450 = Inverse Tangent(1:w526) -> (0:w527:dbl)
        n451 = Divide(x=w527, y=6.283185307179586) -> (x/y=w528:dbl)
        n452 = Multiply(x=360.0, y=w528) -> (x*y=w531:dbl)
        n453 = property on="atan Y/Z" class="DigNum (strict)"("Val(Sgnl)"=w531) -> ()  [unwired: 2 in, 2 out]
      }
      event "Reset Y Position mm", "Reset X Position mm", "Reset Z Position mm", "Reset R Position deg": Value Change {
        n454 = event-data() -> ()  [unwired: 1 in, 5 out]
        n455 = property on="Y offset mm" class="DigNum (strict)"() -> ("Value"=w1146:dbl)  [unwired: 2 in, 2 out]
        n456 = property on="X offset mm" class="DigNum (strict)"() -> ("Value"=w1137:dbl)  [unwired: 2 in, 2 out]
        n457 = property on="R offset deg" class="DigNum (strict)"() -> ("Value"=w1119:dbl)  [unwired: 2 in, 2 out]
        n458 = property on="Y steps/rev" class="DigNum (strict)"() -> ("Value"=w1148:u32)  [unwired: 2 in, 2 out]
        n459 = property on="X steps/rev" class="DigNum (strict)"() -> ("Value"=w1139:u32)  [unwired: 2 in, 2 out]
        n460 = property on="R steps/rev" class="DigNum (strict)"() -> ("Value"=w1121:u32)  [unwired: 2 in, 2 out]
        n461 = property on="Z steps/rev" class="DigNum (strict)"() -> ("Value"=w1130:u32)  [unwired: 2 in, 2 out]
        n462 = property on="Reset Y Position mm" class="DigNum (strict)"() -> ("Value"=w1154:dbl)  [unwired: 2 in, 2 out]
        n463 = property on="Reset X Position mm" class="DigNum (strict)"() -> ("Value"=w1145:dbl)  [unwired: 2 in, 2 out]
        n464 = property on="Reset Z Position mm" class="DigNum (strict)"() -> ("Value"=w1136:dbl)  [unwired: 2 in, 2 out]
        n465 = property on="Reset R Position deg" class="DigNum (strict)"() -> ("Value"=w1127:dbl)  [unwired: 2 in, 2 out]
        n466 = property on="Z offset mm" class="DigNum (strict)"() -> ("Value"=w1128:dbl)  [unwired: 2 in, 2 out]
        n467 = Subtract(x=w1154, y=w1146) -> (x-y=w1153:dbl)
        n468 = Subtract(x=w1145, y=w1137) -> (x-y=w1144:dbl)
        n469 = Subtract(x=w1127, y=w1119) -> (x-y=w1126:dbl)
        n470 = Subtract(x=w1136, y=w1128) -> (x-y=w1135:dbl)
        n471 = To Double Precision Float(number=w1139) -> (double precision float=w1142:dbl)
        n472 = To Double Precision Float(number=w1130) -> (double precision float=w1133:dbl)
        n473 = property on="Y mm/rev" class="DigNum (strict)"() -> ("Value"=w1147:dbl)  [unwired: 2 in, 2 out]
        n474 = property on="X mm/rev" class="DigNum (strict)"() -> ("Value"=w1138:dbl)  [unwired: 2 in, 2 out]
        n475 = property on="Z mm/rev" class="DigNum (strict)"() -> ("Value"=w1129:dbl)  [unwired: 2 in, 2 out]
        n476 = property on="R deg/rev" class="DigNum (strict)"() -> ("Value"=w1120:dbl)  [unwired: 2 in, 2 out]
        n477 = Divide(x=w1153, y=w1147) -> (x/y=w1152:dbl)
        n478 = Divide(x=w1144, y=w1138) -> (x/y=w1143:dbl)
        n479 = Divide(x=w1126, y=w1120) -> (x/y=w1125:dbl)
        n480 = Divide(x=w1135, y=w1129) -> (x/y=w1134:dbl)
        n481 = To Double Precision Float(number=w1148) -> (double precision float=w1151:dbl)
        n482 = To Double Precision Float(number=w1121) -> (double precision float=w1124:dbl)
        n483 = Multiply(x=w1152, y=w1151) -> (x*y=w1150:dbl)
        n484 = Multiply(x=w1143, y=w1142) -> (x*y=w1141:dbl)
        n485 = Multiply(x=w1125, y=w1124) -> (x*y=w1123:dbl)
        n486 = Multiply(x=w1134, y=w1133) -> (x*y=w1132:dbl)
        n487 = To Long Integer(number=w1150) -> (32bit integer=w1149:i32)
        n488 = To Long Integer(number=w1141) -> (32bit integer=w1140:i32)
        n489 = To Long Integer(number=w1123) -> (32bit integer=w1122:i32)
        n490 = To Long Integer(number=w1132) -> (32bit integer=w1131:i32)
        n491 = property on="Reset Y Motor Steps" class="DigNum (strict)"("Val(Sgnl)"=w1149) -> ()  [unwired: 2 in, 2 out]
        n492 = property on="Reset X Motor Steps" class="DigNum (strict)"("Val(Sgnl)"=w1140) -> ()  [unwired: 2 in, 2 out]
        n493 = property on="Reset R Motor Steps" class="DigNum (strict)"("Val(Sgnl)"=w1122) -> ()  [unwired: 2 in, 2 out]
        n494 = property on="Reset Z Motor Steps" class="DigNum (strict)"("Val(Sgnl)"=w1131) -> ()  [unwired: 2 in, 2 out]
      }
      event "Y Velocity SP step/sec", "X Velocity SP step/sec", "R Velocity SP step/sec", "Z Velocity SP step/sec", "Y Step SP", "X Step SP", "Z Step SP", "R Step SP": Value Change {
        n495 = event-data() -> ()  [unwired: 1 in, 5 out]
        n496 = property on="X Step SP" class="DigNum (strict)"() -> ("Value"=w1179:i32)  [unwired: 2 in, 2 out]
        n497 = property on="Z Step SP" class="DigNum (strict)"() -> ("Value"=w1171:i32)  [unwired: 2 in, 2 out]
        n498 = property on="R Step SP" class="DigNum (strict)"() -> ("Value"=w1163:i32)  [unwired: 2 in, 2 out]
        n499 = property on="X offset mm" class="DigNum (strict)"() -> ("Value"=w1176:dbl)  [unwired: 2 in, 2 out]
        n500 = property on="Z offset mm" class="DigNum (strict)"() -> ("Value"=w1168:dbl)  [unwired: 2 in, 2 out]
        n501 = property on="R offset deg" class="DigNum (strict)"() -> ("Value"=w1160:dbl)  [unwired: 2 in, 2 out]
        n502 = property on="Y steps/rev" class="DigNum (strict)"() -> ("Value"=w1185:u32)  [unwired: 2 in, 2 out]
        n503 = property on="Y steps/rev" class="DigNum (strict)"() -> ("Value"=w1210:u32)  [unwired: 2 in, 2 out]
        n504 = property on="X steps/rev" class="DigNum (strict)"() -> ("Value"=w1177:u32)  [unwired: 2 in, 2 out]
        n505 = property on="X steps/rev" class="DigNum (strict)"() -> ("Value"=w1204:u32)  [unwired: 2 in, 2 out]
        n506 = property on="Z steps/rev" class="DigNum (strict)"() -> ("Value"=w1169:u32)  [unwired: 2 in, 2 out]
        n507 = property on="Z steps/rev" class="DigNum (strict)"() -> ("Value"=w1198:u32)  [unwired: 2 in, 2 out]
        n508 = property on="R steps/rev" class="DigNum (strict)"() -> ("Value"=w1161:u32)  [unwired: 2 in, 2 out]
        n509 = property on="R steps/rev" class="DigNum (strict)"() -> ("Value"=w1192:u32)  [unwired: 2 in, 2 out]
        n510 = property on="Y Step SP" class="DigNum (strict)"() -> ("Value"=w1187:i32)  [unwired: 2 in, 2 out]
        n511 = property on="Y Velocity SP step/sec" class="DigNum (strict)"() -> ("Value"=w1212:i32)  [unwired: 2 in, 2 out]
        n512 = property on="X Velocity SP step/sec" class="DigNum (strict)"() -> ("Value"=w1206:i32)  [unwired: 2 in, 2 out]
        n513 = property on="Z Velocity SP step/sec" class="DigNum (strict)"() -> ("Value"=w1200:i32)  [unwired: 2 in, 2 out]
        n514 = property on="R Velocity SP step/sec" class="DigNum (strict)"() -> ("Value"=w1194:i32)  [unwired: 2 in, 2 out]
        n515 = To Double Precision Float(number=w1187) -> (double precision float=w1188:dbl)
        n516 = To Double Precision Float(number=w1185) -> (double precision float=w1191:dbl)
        n517 = To Double Precision Float(number=w1210) -> (double precision float=w1215:dbl)
        n518 = To Double Precision Float(number=w1179) -> (double precision float=w1180:dbl)
        n519 = To Double Precision Float(number=w1177) -> (double precision float=w1183:dbl)
        n520 = To Double Precision Float(number=w1204) -> (double precision float=w1209:dbl)
        n521 = To Double Precision Float(number=w1171) -> (double precision float=w1172:dbl)
        n522 = To Double Precision Float(number=w1169) -> (double precision float=w1175:dbl)
        n523 = To Double Precision Float(number=w1198) -> (double precision float=w1203:dbl)
        n524 = To Double Precision Float(number=w1163) -> (double precision float=w1164:dbl)
        n525 = To Double Precision Float(number=w1161) -> (double precision float=w1167:dbl)
        n526 = To Double Precision Float(number=w1192) -> (double precision float=w1197:dbl)
        n527 = Divide(x=w1188, y=w1191) -> (x/y=w1190:dbl)
        n528 = Divide(x=w1180, y=w1183) -> (x/y=w1182:dbl)
        n529 = Divide(x=w1172, y=w1175) -> (x/y=w1174:dbl)
        n530 = Divide(x=w1164, y=w1167) -> (x/y=w1166:dbl)
        n531 = To Double Precision Float(number=w1212) -> (double precision float=w1213:dbl)
        n532 = To Double Precision Float(number=w1206) -> (double precision float=w1207:dbl)
        n533 = To Double Precision Float(number=w1200) -> (double precision float=w1201:dbl)
        n534 = To Double Precision Float(number=w1194) -> (double precision float=w1195:dbl)
        n535 = property on="Y mm/rev" class="DigNum (strict)"() -> ("Value"=w1156:dbl)  [unwired: 2 in, 2 out]
        n536 = property on="X mm/rev" class="DigNum (strict)"() -> ("Value"=w1157:dbl)  [unwired: 2 in, 2 out]
        n537 = property on="Z mm/rev" class="DigNum (strict)"() -> ("Value"=w1158:dbl)  [unwired: 2 in, 2 out]
        n538 = property on="R deg/rev" class="DigNum (strict)"() -> ("Value"=w1159:dbl)  [unwired: 2 in, 2 out]
        n539 = Multiply(x=w1190, y=w1156) -> (x*y=w1189:dbl)
        n540 = Divide(x=w1213, y=w1215) -> (x/y=w1214:dbl)
        n541 = Multiply(x=w1182, y=w1157) -> (x*y=w1181:dbl)
        n542 = Divide(x=w1207, y=w1209) -> (x/y=w1208:dbl)
        n543 = Multiply(x=w1174, y=w1158) -> (x*y=w1173:dbl)
        n544 = Divide(x=w1201, y=w1203) -> (x/y=w1202:dbl)
        n545 = Multiply(x=w1166, y=w1159) -> (x*y=w1165:dbl)
        n546 = Divide(x=w1195, y=w1197) -> (x/y=w1196:dbl)
        n547 = property on="Y offset mm" class="DigNum (strict)"() -> ("Value"=w1184:dbl)  [unwired: 2 in, 2 out]
        n548 = Add(x=w1189, y=w1184) -> (x+y=w1186:dbl)
        n549 = Multiply(x=w1214, y=w1156) -> (x*y=w1211:dbl)
        n550 = Add(x=w1181, y=w1176) -> (x+y=w1178:dbl)
        n551 = Multiply(x=w1208, y=w1157) -> (x*y=w1205:dbl)
        n552 = Add(x=w1173, y=w1168) -> (x+y=w1170:dbl)
        n553 = Multiply(x=w1202, y=w1158) -> (x*y=w1199:dbl)
        n554 = Add(x=w1165, y=w1160) -> (x+y=w1162:dbl)
        n555 = Multiply(x=w1196, y=w1159) -> (x*y=w1193:dbl)
        n556 = property on="Y Position MV mm" class="DigNum (strict)"("Val(Sgnl)"=w1186) -> ()  [unwired: 2 in, 2 out]
        n557 = property on="Y Velocity MV mm/sec" class="DigNum (strict)"("Val(Sgnl)"=w1211) -> ()  [unwired: 2 in, 2 out]
        n558 = property on="X Position MV mm" class="DigNum (strict)"("Val(Sgnl)"=w1178) -> ()  [unwired: 2 in, 2 out]
        n559 = property on="X Velocity MV mm/sec" class="DigNum (strict)"("Val(Sgnl)"=w1205) -> ()  [unwired: 2 in, 2 out]
        n560 = property on="Z Position MV mm" class="DigNum (strict)"("Val(Sgnl)"=w1170) -> ()  [unwired: 2 in, 2 out]
        n561 = property on="Z Velocity MV mm/sec" class="DigNum (strict)"("Val(Sgnl)"=w1199) -> ()  [unwired: 2 in, 2 out]
        n562 = property on="R Position MV deg" class="DigNum (strict)"("Val(Sgnl)"=w1162) -> ()  [unwired: 2 in, 2 out]
        n563 = Absolute Value(x=w1193) -> (abs(x)=w1155:dbl)
        n564 = property on="R Velocity MVdeg/sec" class="DigNum (strict)"("Val(Sgnl)"=w1155) -> ()  [unwired: 2 in, 2 out]
      }
      event "Y Scan Length SP steps", "Y Scan Velocity SP steps/sec", "X Scan Velocity SP steps/sec", "X Scan Length SP steps", "Z Scan Velocity SP steps/sec", "Z Scan Length SP steps", "R Scan Velocity SP steps/sec", "R Scan Length SP steps": Value Change {
        n565 = event-data() -> ()  [unwired: 1 in, 5 out]
        n566 = property on="X Step PV" class="DigNum (strict)"() -> ("Value"=w1284:i32)  [unwired: 2 in, 2 out]
        n567 = property on="Y Step PV" class="DigNum (strict)"() -> ("Value"=w1270:i32)  [unwired: 2 in, 2 out]
        n568 = property on="Z Step PV" class="DigNum (strict)"() -> ("Value"=w1257:i32)  [unwired: 2 in, 2 out]
        n569 = property on="R Step PV" class="DigNum (strict)"() -> ("Value"=w1243:i32)  [unwired: 2 in, 2 out]
        n570 = property on="X Step SP" class="DigNum (strict)"() -> ("Minimum"=w1291:dbl)  [unwired: 2 in, 2 out]
        n571 = property on="X Step SP" class="DigNum (strict)"() -> ("Maximum"=w1290:dbl)  [unwired: 2 in, 2 out]
        n572 = property on="Y Step SP" class="DigNum (strict)"() -> ("Maximum"=w1276:dbl)  [unwired: 2 in, 2 out]
        n573 = property on="Y Step SP" class="DigNum (strict)"() -> ("Minimum"=w1277:dbl)  [unwired: 2 in, 2 out]
        n574 = property on="Z Step SP" class="DigNum (strict)"() -> ("Maximum"=w1263:dbl)  [unwired: 2 in, 2 out]
        n575 = property on="Z Step SP" class="DigNum (strict)"() -> ("Minimum"=w1264:dbl)  [unwired: 2 in, 2 out]
        n576 = property on="R Step SP" class="DigNum (strict)"() -> ("Maximum"=w1251:dbl)  [unwired: 2 in, 2 out]
        n577 = property on="R Step SP" class="DigNum (strict)"() -> ("Minimum"=w1248:dbl)  [unwired: 2 in, 2 out]
        n578 = property on="X steps/rev" class="DigNum (strict)"() -> ("Value"=w1286:u32)  [unwired: 2 in, 2 out]
        n579 = property on="R steps/rev" class="DigNum (strict)"() -> ("Value"=w1245:u32)  [unwired: 2 in, 2 out]
        n580 = property on="Z steps/rev" class="DigNum (strict)"() -> ("Value"=w1259:u32)  [unwired: 2 in, 2 out]
        n581 = property on="Y steps/rev" class="DigNum (strict)"() -> ("Value"=w1272:u32)  [unwired: 2 in, 2 out]
        n582 = To Double Precision Float(number=w1284) -> (double precision float=w1237:dbl)
        n583 = To Double Precision Float(number=w1270) -> (double precision float=w1236:dbl)
        n584 = To Double Precision Float(number=w1257) -> (double precision float=w1235:dbl)
        n585 = To Double Precision Float(number=w1243) -> (double precision float=w1234:dbl)
        n586 = property on="X Scan Length SP steps" class="DigNum (strict)"() -> ("Value"=w1282:i32)  [unwired: 2 in, 2 out]
        n587 = property on="R Scan Length SP steps" class="DigNum (strict)"() -> ("Value"=w1246:i32)  [unwired: 2 in, 2 out]
        n588 = property on="Z Scan Length SP steps" class="DigNum (strict)"() -> ("Value"=w1260:i32)  [unwired: 2 in, 2 out]
        n589 = property on="Y Scan Length SP steps" class="DigNum (strict)"() -> ("Value"=w1273:i32)  [unwired: 2 in, 2 out]
        n590 = Subtract(x=w1291, y=w1237) -> (x-y=w1292:dbl)
        n591 = Subtract(x=w1290, y=w1237) -> (x-y=w1289:dbl)
        n592 = Subtract(x=w1276, y=w1236) -> (x-y=w1275:dbl)
        n593 = Subtract(x=w1277, y=w1236) -> (x-y=w1278:dbl)
        n594 = Subtract(x=w1263, y=w1235) -> (x-y=w1262:dbl)
        n595 = Subtract(x=w1264, y=w1235) -> (x-y=w1265:dbl)
        n596 = Subtract(x=w1251, y=w1234) -> (x-y=w1250:dbl)
        n597 = Subtract(x=w1248, y=w1234) -> (x-y=w1249:dbl)
        n598 = property on="X Scan Velocity SP steps/sec" class="DigNum (strict)"() -> ("Value"=w1287:i32)  [unwired: 2 in, 2 out]
        n599 = property on="Y Scan Velocity SP steps/sec" class="DigNum (strict)"() -> ("Value"=w1269:i32)  [unwired: 2 in, 2 out]
        n600 = property on="R Scan Velocity SP steps/sec" class="DigNum (strict)"() -> ("Value"=w1241:i32)  [unwired: 2 in, 2 out]
        n601 = property on="Z Scan Velocity SP steps/sec" class="DigNum (strict)"() -> ("Value"=w1255:i32)  [unwired: 2 in, 2 out]
        n602 = property on="X Scan Length SP steps" class="DigNum (strict)"("Minimum"=w1292) -> ()  [unwired: 2 in, 2 out]
        n603 = property on="X Scan Length SP steps" class="DigNum (strict)"("Maximum"=w1289) -> ()  [unwired: 2 in, 2 out]
        n604 = property on="Y Scan Length SP steps" class="DigNum (strict)"("Maximum"=w1275) -> ()  [unwired: 2 in, 2 out]
        n605 = property on="Y Scan Length SP steps" class="DigNum (strict)"("Minimum"=w1278) -> ()  [unwired: 2 in, 2 out]
        n606 = property on="Z Scan Length SP steps" class="DigNum (strict)"("Maximum"=w1262) -> ()  [unwired: 2 in, 2 out]
        n607 = property on="Z Scan Length SP steps" class="DigNum (strict)"("Minimum"=w1265) -> ()  [unwired: 2 in, 2 out]
        n608 = property on="R Scan Length SP steps" class="DigNum (strict)"("Maximum"=w1250) -> ()  [unwired: 2 in, 2 out]
        n609 = property on="R Scan Length SP steps" class="DigNum (strict)"("Minimum"=w1249) -> ()  [unwired: 2 in, 2 out]
        n610 = To Double Precision Float(number=w1286) -> (double precision float=w1283:dbl)
        n611 = To Double Precision Float(number=w1282) -> (double precision float=w1222:dbl)
        n612 = To Double Precision Float(number=w1245) -> (double precision float=w1242:dbl)
        n613 = To Double Precision Float(number=w1246) -> (double precision float=w1231:dbl)
        n614 = To Double Precision Float(number=w1259) -> (double precision float=w1256:dbl)
        n615 = To Double Precision Float(number=w1260) -> (double precision float=w1233:dbl)
        n616 = To Double Precision Float(number=w1272) -> (double precision float=w1227:dbl)
        n617 = To Double Precision Float(number=w1273) -> (double precision float=w1226:dbl)
        n618 = Divide(x=w1222, y=w1283) -> (x/y=w1281:dbl)
        n619 = Divide(x=w1231, y=w1242) -> (x/y=w1247:dbl)
        n620 = Divide(x=w1233, y=w1256) -> (x/y=w1261:dbl)
        n621 = Divide(x=w1226, y=w1227) -> (x/y=w1274:dbl)
        n622 = property on="X mm/rev" class="DigNum (strict)"() -> ("Value"=w1285:dbl)  [unwired: 2 in, 2 out]
        n623 = property on="Z mm/rev" class="DigNum (strict)"() -> ("Value"=w1258:dbl)  [unwired: 2 in, 2 out]
        n624 = property on="Y mm/rev" class="DigNum (strict)"() -> ("Value"=w1271:dbl)  [unwired: 2 in, 2 out]
        n625 = property on="R deg/rev" class="DigNum (strict)"() -> ("Value"=w1244:dbl)  [unwired: 2 in, 2 out]
        n626 = To Double Precision Float(number=w1287) -> (double precision float=w1221:dbl)
        n627 = To Double Precision Float(number=w1241) -> (double precision float=w1230:dbl)
        n628 = To Double Precision Float(number=w1255) -> (double precision float=w1232:dbl)
        n629 = To Double Precision Float(number=w1269) -> (double precision float=w1225:dbl)
        n630 = Multiply(x=w1285, y=w1281) -> (x*y=w1279:dbl)
        n631 = Divide(x=w1221, y=w1283) -> (x/y=w1288:dbl)
        n632 = Divide(x=w1222, y=w1221) -> (x/y=w1223:dbl)
        n633 = Multiply(x=w1247, y=w1244) -> (x*y=w1239:dbl)
        n634 = Divide(x=w1230, y=w1242) -> (x/y=w1240:dbl)
        n635 = Divide(x=w1231, y=w1230) -> (x/y=w1229:dbl)
        n636 = Multiply(x=w1261, y=w1258) -> (x*y=w1253:dbl)
        n637 = Divide(x=w1232, y=w1256) -> (x/y=w1254:dbl)
        n638 = Divide(x=w1233, y=w1232) -> (x/y=w1228:dbl)
        n639 = Multiply(x=w1274, y=w1271) -> (x*y=w1267:dbl)
        n640 = Divide(x=w1225, y=w1227) -> (x/y=w1268:dbl)
        n641 = Divide(x=w1226, y=w1225) -> (x/y=w1224:dbl)
        n642 = property on="X Scan length MV mm" class="DigNum (strict)"("Val(Sgnl)"=w1279) -> ()  [unwired: 2 in, 2 out]
        n643 = property on="R Scan length MV deg" class="DigNum (strict)"("Value"=w1239) -> ()  [unwired: 2 in, 2 out]
        n644 = property on="Z Scan length MV mm" class="DigNum (strict)"("Value"=w1253) -> ()  [unwired: 2 in, 2 out]
        n645 = property on="Y Scan length MV mm" class="DigNum (strict)"("Value"=w1267) -> ()  [unwired: 2 in, 2 out]
        n646 = Multiply(x=w1288, y=w1285) -> (x*y=w1280:dbl)
        n647 = Multiply(x=w1244, y=w1240) -> (x*y=w1238:dbl)
        n648 = Multiply(x=w1258, y=w1254) -> (x*y=w1252:dbl)
        n649 = Multiply(x=w1271, y=w1268) -> (x*y=w1266:dbl)
        n650 = Absolute Value(x=w1223) -> (abs(x)=→"X Scan Duration":dbl)
        n651 = Absolute Value(x=w1229) -> (abs(x)=→"R Scan Duration":dbl)
        n652 = Absolute Value(x=w1228) -> (abs(x)=→"Z Scan Duration":dbl)
        n653 = Absolute Value(x=w1224) -> (abs(x)=→"Y Scan Duration":dbl)
        n654 = property on="X Scan velocity MV mm/sec" class="DigNum (strict)"("Value"=w1280) -> ()  [unwired: 2 in, 2 out]
        n655 = property on="Z Scan velocity MV mm/sec" class="DigNum (strict)"("Val(Sgnl)"=w1252) -> ()  [unwired: 2 in, 2 out]
        n656 = property on="Y Scan velocity MV mm/sec" class="DigNum (strict)"("Val(Sgnl)"=w1266) -> ()  [unwired: 2 in, 2 out]
        n657 = Absolute Value(x=w1238) -> (abs(x)=w1220:dbl)
        n658 = property on="R Scan Velocity SP deg/sec" class="DigNum (strict)"("Val(Sgnl)"=w1220) -> ()  [unwired: 2 in, 2 out]
      }
      event "Y Move Set": Mouse Down {
        n659 = event-data() -> ()  [unwired: 1 in, 7 out]
        n660 = property on="Y steps/rev" class="DigNum (strict)"() -> ("Value"=w1309:u32)  [unwired: 2 in, 2 out]
        n661 = property on="Y Velocity SP step/sec" class="DigNum (strict)"() -> ("Maximum"=w1296:dbl)  [unwired: 2 in, 2 out]
        n662 = property on="Y Velocity SP mm/sec" class="DigNum (strict)"() -> ("Value"=w1300:dbl)  [unwired: 2 in, 2 out]
        n663 = property on="Y Velocity SP step/sec" class="DigNum (strict)"() -> ("Minimum"=w1295:dbl)  [unwired: 2 in, 2 out]
        n664 = property on="Y Position SP mm" class="DigNum (strict)"() -> ("Value"=w1306:dbl)  [unwired: 2 in, 2 out]
        n665 = property on="Y offset mm" class="DigNum (strict)"() -> ("Value"=w1307:dbl)  [unwired: 2 in, 2 out]
        n666 = property on="Y mm/rev" class="DigNum (strict)"() -> ("Value"=w1293:dbl)  [unwired: 2 in, 2 out]
        n667 = Divide(x=w1300, y=w1293) -> (x/y=w1301:dbl)
        n668 = Subtract(x=w1306, y=w1307) -> (x-y=w1310:dbl)
        n669 = To Double Precision Float(number=w1309) -> (double precision float=w1294:dbl)
        n670 = Multiply(x=w1301, y=w1294) -> (x*y=w1298:dbl)
        n671 = Divide(x=w1310, y=w1293) -> (x/y=w1311:dbl)
        n672 = property on="Y Step SP" class="DigNum (strict)"() -> ("Maximum"=w1303:dbl)  [unwired: 2 in, 2 out]
        n673 = property on="Y Step SP" class="DigNum (strict)"() -> ("Minimum"=w1302:dbl)  [unwired: 2 in, 2 out]
        n674 = In Range and Coerce(upper limit=w1296, x=w1298, lower limit=w1295) -> (coerced(x)=w1297:dbl)  [unwired: 1 out]
        n675 = Multiply(x=w1311, y=w1294) -> (x*y=w1305:dbl)
        n676 = In Range and Coerce(upper limit=w1303, x=w1305, lower limit=w1302) -> (coerced(x)=w1304:dbl)  [unwired: 1 out]
        n677 = To Long Integer(number=w1297) -> (32bit integer=w1299:i32)
        n678 = property on="Y Velocity SP step/sec" class="DigNum (strict)"("Val(Sgnl)"=w1299) -> ()  [unwired: 2 in, 2 out]
        n679 = To Long Integer(number=w1304) -> (32bit integer=w1308:i32)
        n680 = property on="Y Step SP" class="DigNum (strict)"("Val(Sgnl)"=w1308) -> ()  [unwired: 2 in, 2 out]
      }
      event "X Move Set": Mouse Down {
        n681 = event-data() -> ()  [unwired: 1 in, 7 out]
        n682 = property on="X steps/rev" class="DigNum (strict)"() -> ("Value"=w1328:u32)  [unwired: 2 in, 2 out]
        n683 = property on="X Velocity SP step/sec" class="DigNum (strict)"() -> ("Maximum"=w1315:dbl)  [unwired: 2 in, 2 out]
        n684 = property on="X Velocity SP mm/sec" class="DigNum (strict)"() -> ("Value"=w1319:dbl)  [unwired: 2 in, 2 out]
        n685 = property on="X Velocity SP step/sec" class="DigNum (strict)"() -> ("Minimum"=w1314:dbl)  [unwired: 2 in, 2 out]
        n686 = property on="X Position SP mm" class="DigNum (strict)"() -> ("Value"=w1325:dbl)  [unwired: 2 in, 2 out]
        n687 = property on="X offset mm" class="DigNum (strict)"() -> ("Value"=w1326:dbl)  [unwired: 2 in, 2 out]
        n688 = property on="X mm/rev" class="DigNum (strict)"() -> ("Value"=w1312:dbl)  [unwired: 2 in, 2 out]
        n689 = Divide(x=w1319, y=w1312) -> (x/y=w1320:dbl)
        n690 = Subtract(x=w1325, y=w1326) -> (x-y=w1329:dbl)
        n691 = To Double Precision Float(number=w1328) -> (double precision float=w1313:dbl)
        n692 = Multiply(x=w1320, y=w1313) -> (x*y=w1317:dbl)
        n693 = Divide(x=w1329, y=w1312) -> (x/y=w1330:dbl)
        n694 = property on="X Step SP" class="DigNum (strict)"() -> ("Maximum"=w1322:dbl)  [unwired: 2 in, 2 out]
        n695 = property on="X Step SP" class="DigNum (strict)"() -> ("Minimum"=w1321:dbl)  [unwired: 2 in, 2 out]
        n696 = In Range and Coerce(upper limit=w1315, x=w1317, lower limit=w1314) -> (coerced(x)=w1316:dbl)  [unwired: 1 out]
        n697 = Multiply(x=w1330, y=w1313) -> (x*y=w1324:dbl)
        n698 = In Range and Coerce(upper limit=w1322, x=w1324, lower limit=w1321) -> (coerced(x)=w1323:dbl)  [unwired: 1 out]
        n699 = To Long Integer(number=w1316) -> (32bit integer=w1318:i32)
        n700 = property on="X Velocity SP step/sec" class="DigNum (strict)"("Val(Sgnl)"=w1318) -> ()  [unwired: 2 in, 2 out]
        n701 = To Long Integer(number=w1323) -> (32bit integer=w1327:i32)
        n702 = property on="X Step SP" class="DigNum (strict)"("Val(Sgnl)"=w1327) -> ()  [unwired: 2 in, 2 out]
      }
      event "Z Move Set": Mouse Down {
        n703 = event-data() -> ()  [unwired: 1 in, 7 out]
        n704 = property on="Z steps/rev" class="DigNum (strict)"() -> ("Value"=w1345:u32)  [unwired: 2 in, 2 out]
        n705 = property on="Z Velocity SP step/sec" class="DigNum (strict)"() -> ("Maximum"=w1332:dbl)  [unwired: 2 in, 2 out]
        n706 = property on="Z Velocity SP mm/sec" class="DigNum (strict)"() -> ("Value"=w1336:dbl)  [unwired: 2 in, 2 out]
        n707 = property on="Z Velocity SP step/sec" class="DigNum (strict)"() -> ("Minimum"=w1331:dbl)  [unwired: 2 in, 2 out]
        n708 = property on="Z Position SP mm" class="DigNum (strict)"() -> ("Value"=w1342:dbl)  [unwired: 2 in, 2 out]
        n709 = property on="Z offset mm" class="DigNum (strict)"() -> ("Value"=w1343:dbl)  [unwired: 2 in, 2 out]
        n710 = property on="Z mm/rev" class="DigNum (strict)"() -> ("Value"=w1348:dbl)  [unwired: 2 in, 2 out]
        n711 = Divide(x=w1336, y=w1348) -> (x/y=w1337:dbl)
        n712 = Subtract(x=w1342, y=w1343) -> (x-y=w1346:dbl)
        n713 = To Double Precision Float(number=w1345) -> (double precision float=w1349:dbl)
        n714 = Multiply(x=w1337, y=w1349) -> (x*y=w1334:dbl)
        n715 = Divide(x=w1346, y=w1348) -> (x/y=w1347:dbl)
        n716 = property on="Z Step SP" class="DigNum (strict)"() -> ("Maximum"=w1339:dbl)  [unwired: 2 in, 2 out]
        n717 = property on="Z Step SP" class="DigNum (strict)"() -> ("Minimum"=w1338:dbl)  [unwired: 2 in, 2 out]
        n718 = In Range and Coerce(upper limit=w1332, x=w1334, lower limit=w1331) -> (coerced(x)=w1333:dbl)  [unwired: 1 out]
        n719 = Multiply(x=w1347, y=w1349) -> (x*y=w1341:dbl)
        n720 = In Range and Coerce(upper limit=w1339, x=w1341, lower limit=w1338) -> (coerced(x)=w1340:dbl)  [unwired: 1 out]
        n721 = To Long Integer(number=w1333) -> (32bit integer=w1335:i32)
        n722 = property on="Z Velocity SP step/sec" class="DigNum (strict)"("Val(Sgnl)"=w1335) -> ()  [unwired: 2 in, 2 out]
        n723 = To Long Integer(number=w1340) -> (32bit integer=w1344:i32)
        n724 = property on="Z Step SP" class="DigNum (strict)"("Val(Sgnl)"=w1344) -> ()  [unwired: 2 in, 2 out]
      }
      event "R Move Set": Mouse Down {
        n725 = event-data() -> ()  [unwired: 1 in, 7 out]
        n726 = property on="R steps/rev" class="DigNum (strict)"() -> ("Value"=w1367:u32)  [unwired: 2 in, 2 out]
        n727 = property on="R Velocity SP step/sec" class="DigNum (strict)"() -> ("Maximum"=w1354:dbl)  [unwired: 2 in, 2 out]
        n728 = property on="R Velocity SP step/sec" class="DigNum (strict)"() -> ("Minimum"=w1353:dbl)  [unwired: 2 in, 2 out]
        n729 = property on="R Velocity SP deg/sec" class="DigNum (strict)"() -> ("Value"=w1358:dbl)  [unwired: 2 in, 2 out]
        n730 = property on="R Position SP deg" class="DigNum (strict)"() -> ("Value"=w1364:dbl)  [unwired: 2 in, 2 out]
        n731 = property on="R offset deg" class="DigNum (strict)"() -> ("Value"=w1365:dbl)  [unwired: 2 in, 2 out]
        n732 = property on="R deg/rev" class="DigNum (strict)"() -> ("Value"=w1351:dbl)  [unwired: 2 in, 2 out]
        n733 = Divide(x=w1358, y=w1351) -> (x/y=w1359:dbl)
        n734 = Subtract(x=w1364, y=w1365) -> (x-y=w1368:dbl)
        n735 = To Double Precision Float(number=w1367) -> (double precision float=w1352:dbl)
        n736 = Multiply(x=w1359, y=w1352) -> (x*y=w1356:dbl)
        n737 = Divide(x=w1368, y=w1351) -> (x/y=w1369:dbl)
        n738 = property on="R Step SP" class="DigNum (strict)"() -> ("Maximum"=w1361:dbl)  [unwired: 2 in, 2 out]
        n739 = property on="R Step SP" class="DigNum (strict)"() -> ("Minimum"=w1360:dbl)  [unwired: 2 in, 2 out]
        n740 = Multiply(x=w1369, y=w1352) -> (x*y=w1363:dbl)
        n741 = Absolute Value(x=w1356) -> (abs(x)=w1350:dbl)
        n742 = In Range and Coerce(upper limit=w1354, x=w1350, lower limit=w1353) -> (coerced(x)=w1355:dbl)  [unwired: 1 out]
        n743 = In Range and Coerce(upper limit=w1361, x=w1363, lower limit=w1360) -> (coerced(x)=w1362:dbl)  [unwired: 1 out]
        n744 = To Long Integer(number=w1355) -> (32bit integer=w1357:i32)
        n745 = To Long Integer(number=w1362) -> (32bit integer=w1366:i32)
        n746 = property on="R Velocity SP step/sec" class="DigNum (strict)"("Val(Sgnl)"=w1357) -> ()  [unwired: 2 in, 2 out]
        n747 = property on="R Step SP" class="DigNum (strict)"("Val(Sgnl)"=w1366) -> ()  [unwired: 2 in, 2 out]
      }
      event "Y Scan set": Mouse Down {
        n748 = event-data() -> ()  [unwired: 1 in, 7 out]
        n749 = property on="Y steps/rev" class="DigNum (strict)"() -> ("Value"=w1385:u32)  [unwired: 2 in, 2 out]
        n750 = property on="Y Scan Length SP mm" class="DigNum (strict)"() -> ("Value"=w1383:dbl)  [unwired: 2 in, 2 out]
        n751 = property on="Y mm/rev" class="DigNum (strict)"() -> ("Value"=w1370:dbl)  [unwired: 2 in, 2 out]
        n752 = property on="Y Scan Velocity SP steps/sec" class="DigNum (strict)"() -> ("Maximum"=w1373:dbl)  [unwired: 2 in, 2 out]
        n753 = property on="Y Scan Velocity SP steps/sec" class="DigNum (strict)"() -> ("Minimum"=w1372:dbl)  [unwired: 2 in, 2 out]
        n754 = property on="Y Scan Velocity SP mm/sec" class="DigNum (strict)"() -> ("Value"=w1377:dbl)  [unwired: 2 in, 2 out]
        n755 = Divide(x=w1383, y=w1370) -> (x/y=w1386:dbl)
        n756 = To Double Precision Float(number=w1385) -> (double precision float=w1371:dbl)
        n757 = Divide(x=w1377, y=w1370) -> (x/y=w1378:dbl)
        n758 = Multiply(x=w1386, y=w1371) -> (x*y=w1382:dbl)
        n759 = property on="Y Step SP" class="DigNum (strict)"() -> ("Maximum"=w1379:dbl)  [unwired: 2 in, 2 out]
        n760 = property on="Y Step SP" class="DigNum (strict)"() -> ("Minimum"=w1380:dbl)  [unwired: 2 in, 2 out]
        n761 = Multiply(x=w1378, y=w1371) -> (x*y=w1375:dbl)
        n762 = In Range and Coerce(upper limit=w1379, x=w1382, lower limit=w1380) -> (coerced(x)=w1381:dbl)  [unwired: 1 out]
        n763 = In Range and Coerce(upper limit=w1373, x=w1375, lower limit=w1372) -> (coerced(x)=w1374:dbl)  [unwired: 1 out]
        n764 = To Long Integer(number=w1381) -> (32bit integer=w1384:i32)
        n765 = property on="Y Scan Length SP steps" class="DigNum (strict)"("Val(Sgnl)"=w1384) -> ()  [unwired: 2 in, 2 out]
        n766 = To Long Integer(number=w1374) -> (32bit integer=w1376:i32)
        n767 = property on="Y Scan Velocity SP steps/sec" class="DigNum (strict)"("Val(Sgnl)"=w1376) -> ()  [unwired: 2 in, 2 out]
      }
      event "X Scan set": Mouse Down {
        n768 = event-data() -> ()  [unwired: 1 in, 7 out]
        n769 = property on="X Step SP" class="DigNum (strict)"() -> ("Minimum"=w1397:dbl)  [unwired: 2 in, 2 out]
        n770 = property on="X steps/rev" class="DigNum (strict)"() -> ("Value"=w1402:u32)  [unwired: 2 in, 2 out]
        n771 = property on="X Scan Length SP mm" class="DigNum (strict)"() -> ("Value"=w1400:dbl)  [unwired: 2 in, 2 out]
        n772 = property on="X mm/rev" class="DigNum (strict)"() -> ("Value"=w1387:dbl)  [unwired: 2 in, 2 out]
        n773 = property on="X Scan Velocity SP steps/sec" class="DigNum (strict)"() -> ("Maximum"=w1390:dbl)  [unwired: 2 in, 2 out]
        n774 = property on="X Scan Velocity SP steps/sec" class="DigNum (strict)"() -> ("Minimum"=w1389:dbl)  [unwired: 2 in, 2 out]
        n775 = property on="X Scan Velocity SP mm/sec" class="DigNum (strict)"() -> ("Value"=w1394:dbl)  [unwired: 2 in, 2 out]
        n776 = Divide(x=w1400, y=w1387) -> (x/y=w1403:dbl)
        n777 = To Double Precision Float(number=w1402) -> (double precision float=w1388:dbl)
        n778 = Divide(x=w1394, y=w1387) -> (x/y=w1395:dbl)
        n779 = Multiply(x=w1403, y=w1388) -> (x*y=w1399:dbl)
        n780 = property on="X Step SP" class="DigNum (strict)"() -> ("Maximum"=w1396:dbl)  [unwired: 2 in, 2 out]
        n781 = Multiply(x=w1395, y=w1388) -> (x*y=w1392:dbl)
        n782 = In Range and Coerce(upper limit=w1396, x=w1399, lower limit=w1397) -> (coerced(x)=w1398:dbl)  [unwired: 1 out]
        n783 = In Range and Coerce(upper limit=w1390, x=w1392, lower limit=w1389) -> (coerced(x)=w1391:dbl)  [unwired: 1 out]
        n784 = To Long Integer(number=w1398) -> (32bit integer=w1401:i32)
        n785 = property on="X Scan Length SP steps" class="DigNum (strict)"("Val(Sgnl)"=w1401) -> ()  [unwired: 2 in, 2 out]
        n786 = To Long Integer(number=w1391) -> (32bit integer=w1393:i32)
        n787 = property on="X Scan Velocity SP steps/sec" class="DigNum (strict)"("Val(Sgnl)"=w1393) -> ()  [unwired: 2 in, 2 out]
      }
      event "Z Scan set": Mouse Down {
        n788 = event-data() -> ()  [unwired: 1 in, 7 out]
        n789 = property on="Z steps/rev" class="DigNum (strict)"() -> ("Value"=w1419:u32)  [unwired: 2 in, 2 out]
        n790 = property on="Z Scan Length SP mm" class="DigNum (strict)"() -> ("Value"=w1417:dbl)  [unwired: 2 in, 2 out]
        n791 = property on="Z mm/rev" class="DigNum (strict)"() -> ("Value"=w1404:dbl)  [unwired: 2 in, 2 out]
        n792 = property on="Z Scan Velocity SP steps/sec" class="DigNum (strict)"() -> ("Maximum"=w1407:dbl)  [unwired: 2 in, 2 out]
        n793 = property on="Z Scan Velocity SP steps/sec" class="DigNum (strict)"() -> ("Minimum"=w1406:dbl)  [unwired: 2 in, 2 out]
        n794 = property on="Z Scan Velocity SP mm/sec" class="DigNum (strict)"() -> ("Value"=w1411:dbl)  [unwired: 2 in, 2 out]
        n795 = Divide(x=w1417, y=w1404) -> (x/y=w1420:dbl)
        n796 = To Double Precision Float(number=w1419) -> (double precision float=w1405:dbl)
        n797 = Divide(x=w1411, y=w1404) -> (x/y=w1412:dbl)
        n798 = Multiply(x=w1420, y=w1405) -> (x*y=w1416:dbl)
        n799 = property on="Z Step SP" class="DigNum (strict)"() -> ("Maximum"=w1413:dbl)  [unwired: 2 in, 2 out]
        n800 = property on="Z Step SP" class="DigNum (strict)"() -> ("Minimum"=w1414:dbl)  [unwired: 2 in, 2 out]
        n801 = Multiply(x=w1412, y=w1405) -> (x*y=w1409:dbl)
        n802 = In Range and Coerce(upper limit=w1413, x=w1416, lower limit=w1414) -> (coerced(x)=w1415:dbl)  [unwired: 1 out]
        n803 = In Range and Coerce(upper limit=w1407, x=w1409, lower limit=w1406) -> (coerced(x)=w1408:dbl)  [unwired: 1 out]
        n804 = To Long Integer(number=w1415) -> (32bit integer=w1418:i32)
        n805 = property on="Z Scan Length SP steps" class="DigNum (strict)"("Val(Sgnl)"=w1418) -> ()  [unwired: 2 in, 2 out]
        n806 = To Long Integer(number=w1408) -> (32bit integer=w1410:i32)
        n807 = property on="Z Scan Velocity SP steps/sec" class="DigNum (strict)"("Val(Sgnl)"=w1410) -> ()  [unwired: 2 in, 2 out]
      }
      event "R Scan set": Mouse Down {
        n808 = event-data() -> ()  [unwired: 1 in, 7 out]
        n809 = property on="R steps/rev" class="DigNum (strict)"() -> ("Value"=w1437:u32)  [unwired: 2 in, 2 out]
        n810 = property on="R Velocity SP step/sec" class="DigNum (strict)"() -> ("Maximum"=w1425:dbl)  [unwired: 2 in, 2 out]
        n811 = property on="R Scan Length SP deg" class="DigNum (strict)"() -> ("Value"=w1435:dbl)  [unwired: 2 in, 2 out]
        n812 = property on="R deg/rev" class="DigNum (strict)"() -> ("Value"=w1422:dbl)  [unwired: 2 in, 2 out]
        n813 = property on="R Scan Velocity SP steps/sec" class="DigNum (strict)"() -> ("Minimum"=w1424:dbl)  [unwired: 2 in, 2 out]
        n814 = property on="R Scan Velocity SP deg/sec" class="DigNum (strict)"() -> ("Value"=w1429:dbl)  [unwired: 2 in, 2 out]
        n815 = Divide(x=w1435, y=w1422) -> (x/y=w1438:dbl)
        n816 = To Double Precision Float(number=w1437) -> (double precision float=w1423:dbl)
        n817 = Divide(x=w1429, y=w1422) -> (x/y=w1430:dbl)
        n818 = Multiply(x=w1438, y=w1423) -> (x*y=w1434:dbl)
        n819 = property on="R Step SP" class="DigNum (strict)"() -> ("Maximum"=w1431:dbl)  [unwired: 2 in, 2 out]
        n820 = property on="R Step SP" class="DigNum (strict)"() -> ("Minimum"=w1432:dbl)  [unwired: 2 in, 2 out]
        n821 = Multiply(x=w1430, y=w1423) -> (x*y=w1427:dbl)
        n822 = In Range and Coerce(upper limit=w1431, x=w1434, lower limit=w1432) -> (coerced(x)=w1433:dbl)  [unwired: 1 out]
        n823 = Absolute Value(x=w1427) -> (abs(x)=w1421:dbl)
        n824 = To Long Integer(number=w1433) -> (32bit integer=w1436:i32)
        n825 = property on="R Scan Length SP steps" class="DigNum (strict)"("Val(Sgnl)"=w1436) -> ()  [unwired: 2 in, 2 out]
        n826 = In Range and Coerce(upper limit=w1425, x=w1421, lower limit=w1424) -> (coerced(x)=w1426:dbl)  [unwired: 1 out]
        n827 = To Long Integer(number=w1426) -> (32bit integer=w1428:i32)
        n828 = property on="R Scan Velocity SP steps/sec" class="DigNum (strict)"("Val(Sgnl)"=w1428) -> ()  [unwired: 2 in, 2 out]
      }
      event "Y Go": Mouse Up {
        n829 = event-data() -> ()  [unwired: 1 in, 7 out]
        n830 = flat-sequence {
          tunnel: w1443 -> [w1453]
          tunnel: w1444 -> [w1454]
          tunnel: [w1454] -> w1440
          tunnel: [w1453] -> w1439
          tunnel: [w1457] -> w1442
          tunnel: [w1456] -> w1441
          tunnel: w1440 -> [w1459]
          tunnel: w1439 -> [w1458]
          tunnel: [w1477] -> w1446
          tunnel: [w1476] -> w1445
          tunnel: w1442 -> [w1475]
          tunnel: w1441 -> [w1474]
          tunnel: [w1484] -> w1448
          tunnel: [w1483] -> w1447
          tunnel: w1446 -> [w1482]
          tunnel: w1445 -> [w1481]
          tunnel: [w1490] -> w1449
          tunnel: [w1491] -> w1450
          tunnel: w1448 -> [w1491]
          tunnel: w1447 -> [w1489]
          frame #0 {
            n831 = property on="Scan Go" class="Bool"("DisabledEnum"=T2."Disabled and Grayed Out" ("Disabled")) -> ()  [unwired: 2 in, 2 out]
            n832 = property on="Y Go" class="Bool"("DisabledEnum"=T2."Disabled and Grayed Out" ("Disabled")) -> ()  [unwired: 2 in, 2 out]
          }
          frame #1 {
            n833 = property on="Y Backlash" class="DigNum (strict)"() -> ("Value"=w1455:i32)  [unwired: 2 in, 2 out]
            n834 = property on="Y Step PV" class="DigNum (strict)"() -> ("Value"=w1466:i32)  [unwired: 2 in, 2 out]
            n835 = property on="Y Step SP" class="DigNum (strict)"() -> ("Value"=w1467:i32)  [unwired: 2 in, 2 out]
            n836 = Subtract(x=w1467, y=w1466) -> (x-y=w1465:i32)
            n837 = Sign(1:w1455) -> (0:w1463:i32)
            n838 = Sign(1:w1465) -> (0:w1464:i32)
            n839 = Multiply(x=w1464, y=w1463) -> (x*y=w1462:i32)
            n840 = Equal?(x=w1462, y=1) -> (x = y?=w1460:bool)
            n841 = case shown="False" w1460 {
              tunnel: w1459 -> [w1470 w1472]
              tunnel: w1458 -> [w1469 w1471]
              tunnel: [w1469 w1471] -> w1457
              tunnel: [w1470 w1472] -> w1456
              frame False {
                n842 = property on="Y Backlash corr" class="Bool (strict)"("Val(Sgnl)"=FALSE ("Value (Signaling)")) -> ()  [unwired: 2 in, 2 out]
              }
              frame True {
                n843 = property on="Y Backlash corr" class="Bool (strict)"("Val(Sgnl)"=TRUE ("Value (Signaling)")) -> ()  [unwired: 2 in, 2 out]
              }
            }
          }
          frame #2 {
            # "Velocity Setting"
            n844 = property on="Y Velocity SP step/sec" class="DigNum (strict)"() -> ("Value"=w1478:i32)  [unwired: 2 in, 2 out]
            n845 = Number To Decimal String(number=w1478) -> (decimal integer string=w1479:string)  [unwired: 1 in]
            n846 = call "mDrive Send Command.vi"("error in (no error)"=w1475, "Extra"=w1479, "Command"=T1."Max Velocity", "VISA resource name"=w1474) -> ("error out"=w1476:errorcluster, "VISA resource name out"=w1477:refnum<visa-resource-name>)  [unwired: 3 in, 1 out]
          }
          frame #3 {
            # "Move to Abs Position"
            n847 = property on="Y Step SP" class="DigNum (strict)"() -> ("Value"=w1487:i32)  [unwired: 2 in, 2 out]
            n848 = Number To Decimal String(number=w1487) -> (decimal integer string=w1486:string)  [unwired: 1 in]
            n849 = call "mDrive Send Command.vi"("error in (no error)"=w1481, "Extra"=w1486, "Command"=T1."Move to Absolute Position", "VISA resource name"=w1482) -> ("error out"=w1483:errorcluster, "VISA resource name out"=w1484:refnum<visa-resource-name>)  [unwired: 3 in, 1 out]
          }
          frame #4 {
            n850 = call "Time Delay"("error in (no error)"=w1489, "Delay Time (s)"=0.1) -> ("error out"=w1490:errorcluster)  [unwired: 9 in]
          }
        }
      }
      event "Z Go": Mouse Up {
        n851 = event-data() -> ()  [unwired: 1 in, 7 out]
        n852 = flat-sequence {
          tunnel: w1494 -> [w1506]
          tunnel: w1495 -> [w1507]
          tunnel: [w1507] -> w1497
          tunnel: [w1506] -> w1496
          tunnel: [w1510] -> w1499
          tunnel: [w1509] -> w1498
          tunnel: w1497 -> [w1512]
          tunnel: w1496 -> [w1511]
          tunnel: [w1530] -> w1501
          tunnel: [w1529] -> w1500
          tunnel: w1499 -> [w1528]
          tunnel: w1498 -> [w1527]
          tunnel: [w1537] -> w1503
          tunnel: [w1536] -> w1502
          tunnel: w1501 -> [w1535]
          tunnel: w1500 -> [w1534]
          tunnel: [w1543] -> w1493
          tunnel: [w1544] -> w1492
          tunnel: w1503 -> [w1544]
          tunnel: w1502 -> [w1542]
          frame #0 {
            n853 = property on="Scan Go" class="Bool"("DisabledEnum"=T2."Disabled and Grayed Out" ("Disabled")) -> ()  [unwired: 2 in, 2 out]
            n854 = property on="Z Go" class="Bool"("DisabledEnum"=T2."Disabled and Grayed Out" ("Disabled")) -> ()  [unwired: 2 in, 2 out]
          }
          frame #1 {
            n855 = property on="Z Backlash" class="DigNum (strict)"() -> ("Value"=w1508:i32)  [unwired: 2 in, 2 out]
            n856 = property on="Z Step PV" class="DigNum (strict)"() -> ("Value"=w1519:i32)  [unwired: 2 in, 2 out]
            n857 = property on="Z Step SP" class="DigNum (strict)"() -> ("Value"=w1520:i32)  [unwired: 2 in, 2 out]
            n858 = Subtract(x=w1520, y=w1519) -> (x-y=w1518:i32)
            n859 = Sign(1:w1508) -> (0:w1516:i32)
            n860 = Sign(1:w1518) -> (0:w1517:i32)
            n861 = Multiply(x=w1517, y=w1516) -> (x*y=w1515:i32)
            n862 = Equal?(x=w1515, y=1) -> (x = y?=w1513:bool)
            n863 = case shown="True" w1513 {
              tunnel: w1512 -> [w1523 w1525]
              tunnel: w1511 -> [w1522 w1524]
              tunnel: [w1522 w1524] -> w1510
              tunnel: [w1523 w1525] -> w1509
              frame False {
                n864 = property on="Z Backlash corr" class="Bool (strict)"("Val(Sgnl)"=FALSE ("Value (Signaling)")) -> ()  [unwired: 2 in, 2 out]
              }
              frame True {
                n865 = property on="Z Backlash corr" class="Bool (strict)"("Val(Sgnl)"=TRUE ("Value (Signaling)")) -> ()  [unwired: 2 in, 2 out]
              }
            }
          }
          frame #2 {
            # "Velocity Setting"
            n866 = property on="Z Velocity SP step/sec" class="DigNum (strict)"() -> ("Value"=w1531:i32)  [unwired: 2 in, 2 out]
            n867 = Number To Decimal String(number=w1531) -> (decimal integer string=w1532:string)  [unwired: 1 in]
            n868 = call "mDrive Send Command.vi"("error in (no error)"=w1528, "Extra"=w1532, "Command"=T1."Max Velocity", "VISA resource name"=w1527) -> ("error out"=w1529:errorcluster, "VISA resource name out"=w1530:refnum<visa-resource-name>)  [unwired: 3 in, 1 out]
          }
          frame #3 {
            # "Move to Abs Position"
            n869 = property on="Z Step SP" class="DigNum (strict)"() -> ("Value"=w1540:i32)  [unwired: 2 in, 2 out]
            n870 = Number To Decimal String(number=w1540) -> (decimal integer string=w1539:string)  [unwired: 1 in]
            n871 = call "mDrive Send Command.vi"("error in (no error)"=w1534, "Extra"=w1539, "Command"=T1."Move to Absolute Position", "VISA resource name"=w1535) -> ("error out"=w1536:errorcluster, "VISA resource name out"=w1537:refnum<visa-resource-name>)  [unwired: 3 in, 1 out]
          }
          frame #4 {
            n872 = call "Time Delay28"("error in (no error)"=w1542, "Delay Time (s)"=0.1) -> ("error out"=w1543:errorcluster)  [unwired: 9 in]
          }
        }
      }
      event "R Go": Mouse Up {
        n873 = event-data() -> ()  [unwired: 1 in, 7 out]
        n874 = flat-sequence {
          tunnel: w1547 -> [w1559]
          tunnel: w1548 -> [w1560]
          tunnel: [w1560] -> w1550
          tunnel: [w1559] -> w1549
          tunnel: [w1563] -> w1552
          tunnel: [w1562] -> w1551
          tunnel: w1550 -> [w1565]
          tunnel: w1549 -> [w1564]
          tunnel: [w1583] -> w1554
          tunnel: [w1582] -> w1553
          tunnel: w1552 -> [w1581]
          tunnel: w1551 -> [w1580]
          tunnel: [w1590] -> w1556
          tunnel: [w1589] -> w1555
          tunnel: w1554 -> [w1588]
          tunnel: w1553 -> [w1587]
          tunnel: [w1596] -> w1546
          tunnel: [w1597] -> w1545
          tunnel: w1556 -> [w1597]
          tunnel: w1555 -> [w1595]
          frame #0 {
            n875 = property on="Scan Go" class="Bool"("DisabledEnum"=T2."Disabled and Grayed Out" ("Disabled")) -> ()  [unwired: 2 in, 2 out]
            n876 = property on="R Go" class="Bool"("DisabledEnum"=T2."Disabled and Grayed Out" ("Disabled")) -> ()  [unwired: 2 in, 2 out]
          }
          frame #1 {
            n877 = property on="R Backlash" class="DigNum (strict)"() -> ("Value"=w1561:i32)  [unwired: 2 in, 2 out]
            n878 = property on="R Step PV" class="DigNum (strict)"() -> ("Value"=w1572:i32)  [unwired: 2 in, 2 out]
            n879 = property on="R Step SP" class="DigNum (strict)"() -> ("Value"=w1573:i32)  [unwired: 2 in, 2 out]
            n880 = Subtract(x=w1573, y=w1572) -> (x-y=w1571:i32)
            n881 = Sign(1:w1561) -> (0:w1569:i32)
            n882 = Sign(1:w1571) -> (0:w1570:i32)
            n883 = Multiply(x=w1570, y=w1569) -> (x*y=w1568:i32)
            n884 = Equal?(x=w1568, y=1) -> (x = y?=w1566:bool)
            n885 = case shown="True" w1566 {
              tunnel: w1565 -> [w1576 w1578]
              tunnel: w1564 -> [w1575 w1577]
              tunnel: [w1575 w1577] -> w1563
              tunnel: [w1576 w1578] -> w1562
              frame False {
                n886 = property on="R Backlash corr" class="Bool (strict)"("Val(Sgnl)"=FALSE ("Value (Signaling)")) -> ()  [unwired: 2 in, 2 out]
              }
              frame True {
                n887 = property on="R Backlash corr" class="Bool (strict)"("Val(Sgnl)"=TRUE ("Value (Signaling)")) -> ()  [unwired: 2 in, 2 out]
              }
            }
          }
          frame #2 {
            # "Velocity Setting"
            n888 = property on="R Velocity SP step/sec" class="DigNum (strict)"() -> ("Value"=w1584:i32)  [unwired: 2 in, 2 out]
            n889 = Number To Decimal String(number=w1584) -> (decimal integer string=w1585:string)  [unwired: 1 in]
            n890 = call "mDrive Send Command.vi"("error in (no error)"=w1581, "Extra"=w1585, "Command"=T1."Max Velocity", "VISA resource name"=w1580) -> ("error out"=w1582:errorcluster, "VISA resource name out"=w1583:refnum<visa-resource-name>)  [unwired: 3 in, 1 out]
          }
          frame #3 {
            # "Move to Abs Position"
            n891 = property on="R Step SP" class="DigNum (strict)"() -> ("Value"=w1593:i32)  [unwired: 2 in, 2 out]
            n892 = Number To Decimal String(number=w1593) -> (decimal integer string=w1592:string)  [unwired: 1 in]
            n893 = call "mDrive Send Command.vi"("error in (no error)"=w1587, "Extra"=w1592, "Command"=T1."Move to Absolute Position", "VISA resource name"=w1588) -> ("error out"=w1589:errorcluster, "VISA resource name out"=w1590:refnum<visa-resource-name>)  [unwired: 3 in, 1 out]
          }
          frame #4 {
            n894 = call "Time Delay29"("error in (no error)"=w1595, "Delay Time (s)"=0.1) -> ("error out"=w1596:errorcluster)  [unwired: 9 in]
          }
        }
      }
      event "X Go": Mouse Up {
        n895 = event-data() -> ()  [unwired: 1 in, 7 out]
        n896 = flat-sequence {
          tunnel: [w1611] -> w1603
          tunnel: [w1610] -> w1602
          tunnel: w1601 -> [w1611]
          tunnel: w1600 -> [w1610]
          tunnel: [w1616] -> w1605
          tunnel: [w1615] -> w1604
          tunnel: w1603 -> [w1618]
          tunnel: w1602 -> [w1617]
          tunnel: [w1636] -> w1607
          tunnel: [w1635] -> w1606
          tunnel: w1605 -> [w1634]
          tunnel: w1604 -> [w1633]
          tunnel: [w1643] -> w1609
          tunnel: [w1642] -> w1608
          tunnel: w1607 -> [w1641]
          tunnel: w1606 -> [w1640]
          tunnel: [w1649] -> w1598
          tunnel: [w1650] -> w1599
          tunnel: w1609 -> [w1650]
          tunnel: w1608 -> [w1648]
          frame #0 {
            n897 = property on="Scan Go" class="Bool"("DisabledEnum"=T2."Disabled and Grayed Out" ("Disabled")) -> ()  [unwired: 2 in, 2 out]
            n898 = property on="X Go" class="Bool"("DisabledEnum"=T2."Disabled and Grayed Out" ("Disabled")) -> ()  [unwired: 2 in, 2 out]
          }
          frame #1 {
            n899 = property on="X Backlash" class="DigNum (strict)"() -> ("Value"=w1614:i32)  [unwired: 2 in, 2 out]
            n900 = property on="X Step PV" class="DigNum (strict)"() -> ("Value"=w1625:i32)  [unwired: 2 in, 2 out]
            n901 = property on="X Step SP" class="DigNum (strict)"() -> ("Value"=w1626:i32)  [unwired: 2 in, 2 out]
            n902 = Subtract(x=w1626, y=w1625) -> (x-y=w1624:i32)
            n903 = Sign(1:w1614) -> (0:w1622:i32)
            n904 = Sign(1:w1624) -> (0:w1623:i32)
            n905 = Multiply(x=w1623, y=w1622) -> (x*y=w1621:i32)
            n906 = Equal?(x=w1621, y=1) -> (x = y?=w1619:bool)
            n907 = case shown="True" w1619 {
              tunnel: w1618 -> [w1629 w1631]
              tunnel: w1617 -> [w1628 w1630]
              tunnel: [w1628 w1630] -> w1616
              tunnel: [w1629 w1631] -> w1615
              frame False {
                n908 = property on="X Backlash corr" class="Bool (strict)"("Val(Sgnl)"=FALSE ("Value (Signaling)")) -> ()  [unwired: 2 in, 2 out]
              }
              frame True {
                n909 = property on="X Backlash corr" class="Bool (strict)"("Val(Sgnl)"=TRUE ("Value (Signaling)")) -> ()  [unwired: 2 in, 2 out]
              }
            }
          }
          frame #2 {
            # "Velocity Setting"
            n910 = property on="X Velocity SP step/sec" class="DigNum (strict)"() -> ("Value"=w1637:i32)  [unwired: 2 in, 2 out]
            n911 = Number To Decimal String(number=w1637) -> (decimal integer string=w1638:string)  [unwired: 1 in]
            n912 = call "mDrive Send Command.vi"("error in (no error)"=w1634, "Extra"=w1638, "Command"=T1."Max Velocity", "VISA resource name"=w1633) -> ("error out"=w1635:errorcluster, "VISA resource name out"=w1636:refnum<visa-resource-name>)  [unwired: 3 in, 1 out]
          }
          frame #3 {
            # "Move to Abs Position"
            n913 = property on="X Step SP" class="DigNum (strict)"() -> ("Value"=w1646:i32)  [unwired: 2 in, 2 out]
            n914 = Number To Decimal String(number=w1646) -> (decimal integer string=w1645:string)  [unwired: 1 in]
            n915 = call "mDrive Send Command.vi"("error in (no error)"=w1640, "Extra"=w1645, "Command"=T1."Move to Absolute Position", "VISA resource name"=w1641) -> ("error out"=w1642:errorcluster, "VISA resource name out"=w1643:refnum<visa-resource-name>)  [unwired: 3 in, 1 out]
          }
          frame #4 {
            n916 = call "Time Delay15"("error in (no error)"=w1648, "Delay Time (s)"=0.1) -> ("error out"=w1649:errorcluster)  [unwired: 9 in]
          }
        }
      }
      event "X Scan OK": Mouse Up {
        n917 = event-data() -> ()  [unwired: 1 in, 7 out]
        n918 = flat-sequence {
          tunnel: [w1666] -> w1658
          tunnel: [w1664] -> w1657
          tunnel: w1656 -> [w1660]
          tunnel: w1655 -> [w1659]
          tunnel: w1658 -> [w1681]
          tunnel: w1657 -> [w1680]
          tunnel: [w1681] -> w1652
          tunnel: [w1680] -> w1651
          tunnel: [w1683] -> w1653
          tunnel: [w1684] -> w1654
          tunnel: w1652 -> [w1684]
          tunnel: w1651 -> [w1683]
          frame #0 {
            # "VELOCITY"
            n919 = property on="X Scan Velocity SP steps/sec" class="DigNum (strict)"() -> ("Value"=w1667:i32)  [unwired: 2 in, 2 out]
            n920 = Number To Decimal String(number=w1667) -> (decimal integer string=w1668:string)  [unwired: 1 in]
            n921 = call "mDrive Send Command.vi"("error in (no error)"=w1659, "Extra"=w1668, "Command"=T1."Max Velocity", "VISA resource name"=w1660) -> ("error out"=w1669:errorcluster, "VISA resource name out"=w1674:refnum<visa-resource-name>)  [unwired: 3 in, 1 out]
            n922 = call "Time Delay9"("error in (no error)"=w1669) -> ("error out"=w1672:errorcluster)  [unwired: 10 in]
            n923 = call "mDrive Send Command.vi"("error in (no error)"=w1672, "Extra"="VM", "Command"=T1."Print Parameter", "VISA resource name"=w1674) -> ("error out"=w1665:errorcluster, "read buffer"=w1670:string, "VISA resource name out"=w1666:refnum<visa-resource-name>)  [unwired: 3 in]
            n924 = call "Time Delay10"("error in (no error)"=w1665) -> ("error out"=w1664:errorcluster)  [unwired: 10 in]
            n925 = Decimal String To Number(string=w1670, offset=0) -> (number=w1673:i32)  [unwired: 1 in, 1 out]
            n926 = property on="X velocity PV step/sec" class="DigNum (strict)"("Val(Sgnl)"=w1673) -> ()  [unwired: 2 in, 2 out]
          }
          frame #1 {
            n927 = property on="X Scan" class="Bool (strict)"("Val(Sgnl)"=TRUE ("Slew Ready 2")) -> ()  [unwired: 2 in, 2 out]
            n928 = property on="Scan Go" class="Bool"("DisabledEnum"=T2."Enabled" ("Disabled")) -> ()  [unwired: 2 in, 2 out]
            n929 = property on="Scan Cancel" class="Bool"("DisabledEnum"=T2."Enabled" ("Disabled")) -> ()  [unwired: 2 in, 2 out]
            n930 = property on="X Scan Velocity SP steps/sec" class="DigNum (strict)"("DisabledEnum"=T2."Disabled and Grayed Out" ("Disabled")) -> ()  [unwired: 2 in, 2 out]
            n931 = property on="X Scan Length SP steps" class="DigNum (strict)"("DisabledEnum"=T2."Disabled and Grayed Out" ("Disabled")) -> ()  [unwired: 2 in, 2 out]
          }
          frame #2 {
            n932 = property on="X Go" class="Bool"("DisabledEnum"=T2."Disabled and Grayed Out" ("Disabled")) -> ()  [unwired: 2 in, 2 out]
          }
        }
      }
      event "Y Scan OK": Mouse Up {
        n933 = event-data() -> ()  [unwired: 1 in, 7 out]
        n934 = flat-sequence {
          tunnel: w1692 -> [w1702]
          tunnel: w1691 -> [w1701]
          tunnel: [w1698] -> w1689
          tunnel: [w1696] -> w1688
          tunnel: w1689 -> [w1715]
          tunnel: w1688 -> [w1714]
          tunnel: [w1715] -> w1686
          tunnel: [w1714] -> w1685
          tunnel: [w1717] -> w1690
          tunnel: [w1718] -> w1687
          tunnel: w1686 -> [w1718]
          tunnel: w1685 -> [w1717]
          frame #0 {
            # "VELOCITY"
            n935 = property on="Y Scan Velocity SP steps/sec" class="DigNum (strict)"() -> ("Value"=w1699:i32)  [unwired: 2 in, 2 out]
            n936 = Number To Decimal String(number=w1699) -> (decimal integer string=w1700:string)  [unwired: 1 in]
            n937 = call "mDrive Send Command.vi"("error in (no error)"=w1702, "Extra"=w1700, "Command"=T1."Max Velocity", "VISA resource name"=w1701) -> ("error out"=w1703:errorcluster, "VISA resource name out"=w1708:refnum<visa-resource-name>)  [unwired: 3 in, 1 out]
            n938 = call "Time Delay5"("error in (no error)"=w1703) -> ("error out"=w1706:errorcluster)  [unwired: 10 in]
            n939 = call "mDrive Send Command.vi"("error in (no error)"=w1706, "Extra"="VM", "Command"=T1."Print Parameter", "VISA resource name"=w1708) -> ("error out"=w1697:errorcluster, "read buffer"=w1704:string, "VISA resource name out"=w1698:refnum<visa-resource-name>)  [unwired: 3 in]
            n940 = Decimal String To Number(string=w1704, offset=0) -> (number=w1707:i32)  [unwired: 1 in, 1 out]
            n941 = property on="Y velocity PV step/sec" class="DigNum (strict)"("Val(Sgnl)"=w1707) -> ()  [unwired: 2 in, 2 out]
            n942 = call "Time Delay6"("error in (no error)"=w1697) -> ("error out"=w1696:errorcluster)  [unwired: 10 in]
          }
          frame #1 {
            n943 = property on="Y Scan" class="Bool (strict)"("Val(Sgnl)"=TRUE ("Slew Ready 2")) -> ()  [unwired: 2 in, 2 out]
            n944 = property on="Scan Go" class="Bool"("DisabledEnum"=T2."Enabled" ("Disabled")) -> ()  [unwired: 2 in, 2 out]
            n945 = property on="Scan Cancel" class="Bool"("DisabledEnum"=T2."Enabled" ("Disabled")) -> ()  [unwired: 2 in, 2 out]
            n946 = property on="Y Scan Velocity SP steps/sec" class="DigNum (strict)"("DisabledEnum"=T2."Disabled and Grayed Out" ("Disabled")) -> ()  [unwired: 2 in, 2 out]
            n947 = property on="Y Scan Length SP steps" class="DigNum (strict)"("DisabledEnum"=T2."Disabled and Grayed Out" ("Disabled")) -> ()  [unwired: 2 in, 2 out]
          }
          frame #2 {
            n948 = property on="Y Go" class="Bool"("DisabledEnum"=T2."Disabled and Grayed Out" ("Disabled")) -> ()  [unwired: 2 in, 2 out]
          }
        }
      }
      event "Z Scan OK": Mouse Up {
        n949 = event-data() -> ()  [unwired: 1 in, 7 out]
        n950 = flat-sequence {
          tunnel: [w1734] -> w1726
          tunnel: [w1732] -> w1725
          tunnel: w1722 -> [w1728]
          tunnel: w1721 -> [w1727]
          tunnel: w1726 -> [w1749]
          tunnel: w1725 -> [w1748]
          tunnel: [w1749] -> w1724
          tunnel: [w1748] -> w1723
          tunnel: [w1751] -> w1720
          tunnel: [w1752] -> w1719
          tunnel: w1724 -> [w1752]
          tunnel: w1723 -> [w1751]
          frame #0 {
            # "VELOCITY"
            n951 = property on="Z Scan Velocity SP steps/sec" class="DigNum (strict)"() -> ("Value"=w1735:i32)  [unwired: 2 in, 2 out]
            n952 = Number To Decimal String(number=w1735) -> (decimal integer string=w1736:string)  [unwired: 1 in]
            n953 = call "mDrive Send Command.vi"("error in (no error)"=w1727, "Extra"=w1736, "Command"=T1."Max Velocity", "VISA resource name"=w1728) -> ("error out"=w1737:errorcluster, "VISA resource name out"=w1742:refnum<visa-resource-name>)  [unwired: 3 in, 1 out]
            n954 = call "Time Delay24"("error in (no error)"=w1737) -> ("error out"=w1740:errorcluster)  [unwired: 10 in]
            n955 = call "mDrive Send Command.vi"("error in (no error)"=w1740, "Extra"="VM", "Command"=T1."Print Parameter", "VISA resource name"=w1742) -> ("error out"=w1733:errorcluster, "read buffer"=w1738:string, "VISA resource name out"=w1734:refnum<visa-resource-name>)  [unwired: 3 in]
            n956 = Decimal String To Number(string=w1738, offset=0) -> (number=w1741:i32)  [unwired: 1 in, 1 out]
            n957 = property on="Z  velocity PV step/sec" class="DigNum (strict)"("Val(Sgnl)"=w1741) -> ()  [unwired: 2 in, 2 out]
            n958 = call "Time Delay25"("error in (no error)"=w1733) -> ("error out"=w1732:errorcluster)  [unwired: 10 in]
          }
          frame #1 {
            n959 = property on="Z Scan" class="Bool (strict)"("Val(Sgnl)"=TRUE ("Slew Ready 2")) -> ()  [unwired: 2 in, 2 out]
            n960 = property on="Scan Go" class="Bool"("DisabledEnum"=T2."Enabled" ("Disabled")) -> ()  [unwired: 2 in, 2 out]
            n961 = property on="Scan Cancel" class="Bool"("DisabledEnum"=T2."Enabled" ("Disabled")) -> ()  [unwired: 2 in, 2 out]
            n962 = property on="Z Scan Velocity SP steps/sec" class="DigNum (strict)"("DisabledEnum"=T2."Disabled and Grayed Out" ("Disabled")) -> ()  [unwired: 2 in, 2 out]
            n963 = property on="Z Scan Length SP steps" class="DigNum (strict)"("DisabledEnum"=T2."Disabled and Grayed Out" ("Disabled")) -> ()  [unwired: 2 in, 2 out]
          }
          frame #2 {
            n964 = property on="Z Go" class="Bool"("DisabledEnum"=T2."Disabled and Grayed Out" ("Disabled")) -> ()  [unwired: 2 in, 2 out]
          }
        }
      }
      event "R Scan OK": Mouse Up {
        n965 = event-data() -> ()  [unwired: 1 in, 7 out]
        n966 = flat-sequence {
          tunnel: [w1768] -> w1760
          tunnel: [w1766] -> w1759
          tunnel: w1756 -> [w1762]
          tunnel: w1755 -> [w1761]
          tunnel: w1760 -> [w1783]
          tunnel: w1759 -> [w1782]
          tunnel: [w1783] -> w1758
          tunnel: [w1782] -> w1757
          tunnel: [w1785] -> w1753
          tunnel: [w1786] -> w1754
          tunnel: w1758 -> [w1786]
          tunnel: w1757 -> [w1785]
          frame #0 {
            # "VELOCITY"
            n967 = property on="R Scan Velocity SP steps/sec" class="DigNum (strict)"() -> ("Value"=w1769:i32)  [unwired: 2 in, 2 out]
            n968 = Number To Decimal String(number=w1769) -> (decimal integer string=w1770:string)  [unwired: 1 in]
            n969 = call "mDrive Send Command.vi"("error in (no error)"=w1761, "Extra"=w1770, "Command"=T1."Max Velocity", "VISA resource name"=w1762) -> ("error out"=w1771:errorcluster, "VISA resource name out"=w1776:refnum<visa-resource-name>)  [unwired: 3 in, 1 out]
            n970 = call "Time Delay26"("error in (no error)"=w1771) -> ("error out"=w1774:errorcluster)  [unwired: 10 in]
            n971 = call "mDrive Send Command.vi"("error in (no error)"=w1774, "Extra"="VM", "Command"=T1."Print Parameter", "VISA resource name"=w1776) -> ("error out"=w1767:errorcluster, "read buffer"=w1772:string, "VISA resource name out"=w1768:refnum<visa-resource-name>)  [unwired: 3 in]
            n972 = Decimal String To Number(string=w1772, offset=0) -> (number=w1775:i32)  [unwired: 1 in, 1 out]
            n973 = property on="R velocity PV step/sec" class="DigNum (strict)"("Val(Sgnl)"=w1775) -> ()  [unwired: 2 in, 2 out]
            n974 = call "Time Delay27"("error in (no error)"=w1767) -> ("error out"=w1766:errorcluster)  [unwired: 10 in]
          }
          frame #1 {
            n975 = property on="R Scan" class="Bool (strict)"("Val(Sgnl)"=TRUE ("Slew Ready 2")) -> ()  [unwired: 2 in, 2 out]
            n976 = property on="Scan Go" class="Bool"("DisabledEnum"=T2."Enabled" ("Disabled")) -> ()  [unwired: 2 in, 2 out]
            n977 = property on="Scan Cancel" class="Bool"("DisabledEnum"=T2."Enabled" ("Disabled")) -> ()  [unwired: 2 in, 2 out]
            n978 = property on="R Scan Velocity SP steps/sec" class="DigNum (strict)"("DisabledEnum"=T2."Disabled and Grayed Out" ("Disabled")) -> ()  [unwired: 2 in, 2 out]
            n979 = property on="R Scan Length SP steps" class="DigNum (strict)"("DisabledEnum"=T2."Disabled and Grayed Out" ("Disabled")) -> ()  [unwired: 2 in, 2 out]
          }
          frame #2 {
            n980 = property on="R Go" class="Bool"("DisabledEnum"=T2."Disabled and Grayed Out" ("Disabled")) -> ()  [unwired: 2 in, 2 out]
          }
        }
      }
      event Application Instance Close? {
        n981 = event-data() -> ()  [unwired: 1 in, 4 out]
        n982 = event-data() -> ()  [unwired: 3 in, 1 out]
      }
      event "Stop": Mouse Down {
        n983 = event-data() -> ()  [unwired: 1 in, 7 out]
        n984 = flat-sequence {
          tunnel: [w1818] -> w1800
          tunnel: [w1817] -> w1799
          tunnel: w1798 -> [w1816]
          tunnel: w1797 -> [w1815]
          frame #0 {
            n985 = call "mDrive Send Command.vi"("error in (no error)"=w1815, "Command"=T1."Stop", "VISA resource name"=w1816) -> ("error out"=w1817:errorcluster, "VISA resource name out"=w1818:refnum<visa-resource-name>)  [unwired: 4 in, 1 out]
          }
        }
        n986 = flat-sequence {
          tunnel: w1804 -> [w1824]
          tunnel: w1803 -> [w1823]
          tunnel: [w1822] -> w1802
          tunnel: [w1821] -> w1801
          frame #0 {
            n987 = call "mDrive Send Command.vi"("error in (no error)"=w1823, "Command"=T1."Stop", "VISA resource name"=w1824) -> ("error out"=w1821:errorcluster, "VISA resource name out"=w1822:refnum<visa-resource-name>)  [unwired: 4 in, 1 out]
          }
        }
        n988 = flat-sequence {
          tunnel: [w1813] -> w1794
          tunnel: [w1812] -> w1793
          tunnel: w1796 -> [w1811]
          tunnel: w1795 -> [w1810]
          frame #0 {
            n989 = call "mDrive Send Command.vi"("error in (no error)"=w1810, "Command"=T1."Stop", "VISA resource name"=w1811) -> ("error out"=w1812:errorcluster, "VISA resource name out"=w1813:refnum<visa-resource-name>)  [unwired: 4 in, 1 out]
          }
        }
        n990 = flat-sequence {
          tunnel: w1792 -> [w1809]
          tunnel: w1791 -> [w1808]
          tunnel: [w1807] -> w1790
          tunnel: [w1805] -> _
          tunnel: [w1805] -> w1789
          frame #0 {
            n991 = call "mDrive Send Command.vi"("error in (no error)"=w1808, "Command"=T1."Stop", "VISA resource name"=w1809) -> ("error out"=w1805:errorcluster, "VISA resource name out"=w1807:refnum<visa-resource-name>)  [unwired: 4 in, 1 out]
          }
        }
      }
      event "Scan Cancel": Mouse Down {
        n992 = event-data() -> ()  [unwired: 1 in, 7 out]
        n993 = flat-sequence {
          tunnel: w1840 -> [w1879]
          tunnel: w1839 -> [w1878]
          tunnel: [w1881] -> w1842
          tunnel: [w1880] -> w1841
          tunnel: [w1888] -> w1837
          tunnel: [w1889] -> w1838
          tunnel: w1842 -> [w1889]
          tunnel: w1841 -> [w1888]
          frame #0 {
            n994 = call "mDrive Send Command.vi"("error in (no error)"=w1878, "Command"=T1."Stop", "VISA resource name"=w1879) -> ("error out"=w1880:errorcluster, "VISA resource name out"=w1881:refnum<visa-resource-name>)  [unwired: 4 in, 1 out]
          }
          frame #1 {
            n995 = property on="X Scan" class="Bool (strict)"("Value"=FALSE ("Slew Ready")) -> ()  [unwired: 2 in, 2 out]
            n996 = property on="X Scan Velocity SP steps/sec" class="DigNum (strict)"("DisabledEnum"=T2."Enabled" ("Disabled")) -> ()  [unwired: 2 in, 2 out]
            n997 = property on="X Scan Length SP steps" class="DigNum (strict)"("DisabledEnum"=T2."Enabled" ("Disabled")) -> ()  [unwired: 2 in, 2 out]
            n998 = property on="X Scan OK" class="Bool"("DisabledEnum"=T2."Enabled" ("Disabled")) -> ()  [unwired: 2 in, 2 out]
            n999 = property on="X Go" class="Bool"("DisabledEnum"=T2."Enabled" ("Disabled")) -> ()  [unwired: 2 in, 2 out]
            n1000 = property on="X Scan set" class="Bool"("DisabledEnum"=T2."Enabled" ("Disabled")) -> ()  [unwired: 2 in, 2 out]
          }
        }
        n1001 = flat-sequence {
          tunnel: w1848 -> [w1892]
          tunnel: w1847 -> [w1891]
          tunnel: [w1894] -> w1844
          tunnel: [w1893] -> w1843
          tunnel: [w1901] -> w1849
          tunnel: [w1902] -> w1850
          tunnel: w1844 -> [w1902]
          tunnel: w1843 -> [w1901]
          frame #0 {
            n1002 = call "mDrive Send Command.vi"("error in (no error)"=w1891, "Command"=T1."Stop", "VISA resource name"=w1892) -> ("error out"=w1893:errorcluster, "VISA resource name out"=w1894:refnum<visa-resource-name>)  [unwired: 4 in, 1 out]
          }
          frame #1 {
            n1003 = property on="Y Scan" class="Bool (strict)"("Value"=FALSE ("Slew Ready")) -> ()  [unwired: 2 in, 2 out]
            n1004 = property on="Y Scan Velocity SP steps/sec" class="DigNum (strict)"("DisabledEnum"=T2."Enabled" ("Disabled")) -> ()  [unwired: 2 in, 2 out]
            n1005 = property on="Y Scan Length SP steps" class="DigNum (strict)"("DisabledEnum"=T2."Enabled" ("Disabled")) -> ()  [unwired: 2 in, 2 out]
            n1006 = property on="Y Scan OK" class="Bool"("DisabledEnum"=T2."Enabled" ("Disabled")) -> ()  [unwired: 2 in, 2 out]
            n1007 = property on="Y Scan set" class="Bool"("DisabledEnum"=T2."Enabled" ("Disabled")) -> ()  [unwired: 2 in, 2 out]
            n1008 = property on="Y Go" class="Bool"("DisabledEnum"=T2."Enabled" ("Disabled")) -> ()  [unwired: 2 in, 2 out]
          }
        }
        n1009 = flat-sequence {
          tunnel: [w1868] -> w1836
          tunnel: [w1867] -> w1835
          tunnel: w1834 -> [w1865]
          tunnel: w1833 -> [w1864]
          tunnel: [w1875] -> w1831
          tunnel: [w1876] -> w1832
          tunnel: w1836 -> [w1876]
          tunnel: w1835 -> [w1875]
          frame #0 {
            n1010 = call "mDrive Send Command.vi"("error in (no error)"=w1864, "Command"=T1."Stop", "VISA resource name"=w1865) -> ("error out"=w1867:errorcluster, "VISA resource name out"=w1868:refnum<visa-resource-name>)  [unwired: 4 in, 1 out]
          }
          frame #1 {
            n1011 = property on="Z Scan" class="Bool (strict)"("Value"=FALSE ("Slew Ready")) -> ()  [unwired: 2 in, 2 out]
            n1012 = property on="Z Scan Velocity SP steps/sec" class="DigNum (strict)"("DisabledEnum"=T2."Enabled" ("Disabled")) -> ()  [unwired: 2 in, 2 out]
            n1013 = property on="Z Scan Length SP steps" class="DigNum (strict)"("DisabledEnum"=T2."Enabled" ("Disabled")) -> ()  [unwired: 2 in, 2 out]
            n1014 = property on="Z Scan OK" class="Bool"("DisabledEnum"=T2."Enabled" ("Disabled")) -> ()  [unwired: 2 in, 2 out]
            n1015 = property on="Z Go" class="Bool"("DisabledEnum"=T2."Enabled" ("Disabled")) -> ()  [unwired: 2 in, 2 out]
            n1016 = property on="Z Scan set" class="Bool"("DisabledEnum"=T2."Enabled" ("Disabled")) -> ()  [unwired: 2 in, 2 out]
          }
        }
        n1017 = flat-sequence {
          tunnel: [w1855] -> w1830
          tunnel: [w1854] -> w1829
          tunnel: w1828 -> [w1852]
          tunnel: w1827 -> [w1851]
          tunnel: [w1862] -> w1825
          tunnel: [w1863] -> w1826
          tunnel: w1830 -> [w1863]
          tunnel: w1829 -> [w1862]
          frame #0 {
            n1018 = call "mDrive Send Command.vi"("error in (no error)"=w1851, "Command"=T1."Stop", "VISA resource name"=w1852) -> ("error out"=w1854:errorcluster, "VISA resource name out"=w1855:refnum<visa-resource-name>)  [unwired: 4 in, 1 out]
          }
          frame #1 {
            n1019 = property on="R Scan" class="Bool (strict)"("Value"=FALSE ("Slew Ready")) -> ()  [unwired: 2 in, 2 out]
            n1020 = property on="R Scan Velocity SP steps/sec" class="DigNum (strict)"("DisabledEnum"=T2."Enabled" ("Disabled")) -> ()  [unwired: 2 in, 2 out]
            n1021 = property on="R Scan Length SP steps" class="DigNum (strict)"("DisabledEnum"=T2."Enabled" ("Disabled")) -> ()  [unwired: 2 in, 2 out]
            n1022 = property on="R Scan set" class="Bool"("DisabledEnum"=T2."Enabled" ("Disabled")) -> ()  [unwired: 2 in, 2 out]
            n1023 = property on="R Scan OK" class="Bool"("DisabledEnum"=T2."Enabled" ("Disabled")) -> ()  [unwired: 2 in, 2 out]
            n1024 = property on="R Go" class="Bool"("DisabledEnum"=T2."Enabled" ("Disabled")) -> ()  [unwired: 2 in, 2 out]
          }
        }
        n1025 = property on="Scan Cancel" class="Bool"("DisabledEnum"=T2."Disabled and Grayed Out" ("Disabled")) -> ()  [unwired: 2 in, 2 out]
        n1026 = property on="Scan Go" class="Bool"("DisabledEnum"=T2."Disabled and Grayed Out" ("Disabled")) -> ()  [unwired: 2 in, 2 out]
      }
      event "Scan Go": Mouse Up {
        n1027 = event-data() -> ()  [unwired: 1 in, 7 out]
        n1028 = flat-sequence {
          tunnel: [w1982] -> w1966
          tunnel: [w1980] -> w1959
          tunnel: [w1981] -> w1956
          tunnel: [w1975] -> w1955
          tunnel: [w1979] -> w1954
          tunnel: [w1978] -> w1953
          tunnel: [w1977] -> w1952
          tunnel: [w1976] -> w1951
          tunnel: w1930 -> [w1974]
          tunnel: [w1974] -> w1929
          tunnel: w1928 -> [w1973]
          tunnel: [w1973] -> w1927
          tunnel: w1926 -> [w1972]
          tunnel: [w1972] -> w1925
          tunnel: w1924 -> [w1971]
          tunnel: [w1971] -> w1923
          tunnel: w1922 -> [w1970]
          tunnel: [w1970] -> w1921
          tunnel: w1920 -> [w1969]
          tunnel: [w1969] -> w1919
          tunnel: [w1968] -> w1918
          tunnel: w1917 -> [w1968]
          tunnel: [w1967] -> w1916
          tunnel: w1915 -> [w1967]
          tunnel: [w2034] -> w1963
          tunnel: [w2033] -> w1961
          tunnel: w1966 -> [w2032]
          tunnel: w1959 -> [w2031]
          tunnel: [w2031] -> w1957
          tunnel: w1956 -> [w2030]
          tunnel: w1955 -> [w2019]
          tunnel: w1954 -> [w2029]
          tunnel: w1953 -> [w2025]
          tunnel: w1952 -> [w2022]
          tunnel: w1951 -> [w2028]
          tunnel: [w2027] -> w1949
          tunnel: [w2026] -> w1947
          tunnel: [w2025] -> w1944
          tunnel: [w2024] -> w1942
          tunnel: [w2023] -> w1940
          tunnel: [w2022] -> w1938
          tunnel: [w2021] -> w1936
          tunnel: [w2020] -> w1934
          tunnel: [w2019] -> w1933
          tunnel: w1929 -> [w2018]
          tunnel: w1927 -> [w2017]
          tunnel: w1925 -> [w2016]
          tunnel: w1923 -> [w2015]
          tunnel: w1921 -> [w2014]
          tunnel: w1919 -> [w2013]
          tunnel: w1918 -> [w2012]
          tunnel: w1916 -> [w2011]
          tunnel: w1963 -> [w2075]
          tunnel: [w2075] -> w1962
          tunnel: w1961 -> [w2074]
          tunnel: [w2074] -> w1960
          tunnel: [w2072] -> w1958
          tunnel: w1957 -> [w2072]
          tunnel: [w2071] -> w1950
          tunnel: w1949 -> [w2071]
          tunnel: [w2070] -> w1948
          tunnel: w1947 -> [w2070]
          tunnel: [w2069] -> w1946
          tunnel: [w2068] -> w1945
          tunnel: w1944 -> [w2068]
          tunnel: [w2067] -> w1943
          tunnel: w1942 -> [w2067]
          tunnel: [w2066] -> w1941
          tunnel: w1940 -> [w2066]
          tunnel: [w2065] -> w1939
          tunnel: w1938 -> [w2065]
          tunnel: [w2064] -> w1937
          tunnel: w1936 -> [w2064]
          tunnel: [w2063] -> w1935
          tunnel: w1934 -> [w2063]
          tunnel: w1933 -> [w2069]
          tunnel: w1962 -> [w2095]
          tunnel: [w2093] -> w1965
          tunnel: w1960 -> [w2094]
          tunnel: [w2092] -> w1964
          tunnel: w1958 -> [w2091]
          tunnel: w1950 -> [w2090]
          tunnel: w1948 -> [w2089]
          tunnel: w1946 -> [w2088]
          tunnel: w1945 -> [w2087]
          tunnel: w1943 -> [w2086]
          tunnel: w1941 -> [w2085]
          tunnel: w1939 -> [w2084]
          tunnel: w1937 -> [w2083]
          tunnel: w1935 -> [w2082]
          tunnel: [w2081] -> w1932
          tunnel: [w2080] -> w1931
          tunnel: [w2079] -> w1910
          tunnel: [w2078] -> w1907
          tunnel: [w2077] -> w1905
          tunnel: [w2076] -> w1903
          tunnel: w1965 -> [w2153]
          tunnel: w1964 -> [w2152]
          tunnel: [w2153] -> w1914
          tunnel: [w2152] -> w1913
          tunnel: [w2146] -> w1912
          tunnel: w1932 -> [w2146]
          tunnel: [w2145] -> w1911
          tunnel: w1931 -> [w2145]
          tunnel: w1910 -> [w2135]
          tunnel: [w2135] -> w1909
          tunnel: [w2134] -> w1908
          tunnel: w1907 -> [w2134]
          tunnel: [w2133] -> w1906
          tunnel: w1905 -> [w2133]
          tunnel: [w2132] -> w1904
          tunnel: w1903 -> [w2132]
          frame #0 {
            n1029 = property on="X Scan" class="Bool (strict)"() -> ("Value"=w1975:bool)  [unwired: 2 in, 2 out]
            n1030 = property on="Y Scan" class="Bool (strict)"() -> ("Value"=w1980:bool)  [unwired: 2 in, 2 out]
            n1031 = property on="Z Scan" class="Bool (strict)"() -> ("Value"=w1977:bool)  [unwired: 2 in, 2 out]
            n1032 = property on="R Scan" class="Bool (strict)"() -> ("Value"=w1978:bool)  [unwired: 2 in, 2 out]
            n1033 = case shown="True" w1975 {
              tunnel: ["" w1998] -> w1981
              frame False {
              }
              frame True {
                n1034 = property on="X Scan Length SP steps" class="DigNum (strict)"() -> ("Value"=w2003:i32)  [unwired: 2 in, 2 out]
                n1035 = Number To Decimal String(number=w2003) -> (decimal integer string=w2000:string)  [unwired: 1 in]
                n1036 = call <vilib>:"Space Constant.vi"() -> ("String"=w2001:string)
                n1037 = Concatenate Strings("MR", w2001, w2000, "\r") -> (w1998:string)
              }
            }
            n1038 = case shown="True" w1980 {
              tunnel: ["" w2005] -> w1982
              frame False {
              }
              frame True {
                n1039 = property on="Y Scan Length SP steps" class="DigNum (strict)"() -> ("Value"=w2010:i32)  [unwired: 2 in, 2 out]
                n1040 = Number To Decimal String(number=w2010) -> (decimal integer string=w2007:string)  [unwired: 1 in]
                n1041 = call <vilib>:"Space Constant.vi"() -> ("String"=w2008:string)
                n1042 = Concatenate Strings("MR", w2008, w2007, "\r") -> (w2005:string)
              }
            }
            n1043 = case shown="True" w1977 {
              tunnel: ["" w1991] -> w1979
              frame False {
              }
              frame True {
                n1044 = property on="Z Scan Length SP steps" class="DigNum (strict)"() -> ("Value"=w1996:i32)  [unwired: 2 in, 2 out]
                n1045 = Number To Decimal String(number=w1996) -> (decimal integer string=w1993:string)  [unwired: 1 in]
                n1046 = call <vilib>:"Space Constant.vi"() -> ("String"=w1994:string)
                n1047 = Concatenate Strings("MR", w1994, w1993, "\r") -> (w1991:string)
              }
            }
            n1048 = case shown="True" w1978 {
              tunnel: ["" w1984] -> w1976
              frame False {
              }
              frame True {
                n1049 = property on="R Scan Length SP steps" class="DigNum (strict)"() -> ("Value"=w1989:i32)  [unwired: 2 in, 2 out]
                n1050 = Number To Decimal String(number=w1989) -> (decimal integer string=w1986:string)  [unwired: 1 in]
                n1051 = call <vilib>:"Space Constant.vi"() -> ("String"=w1987:string)
                n1052 = Concatenate Strings("MR", w1987, w1986, "\r") -> (w1984:string)
              }
            }
          }
          frame #1 {
            n1053 = case shown="False" w2019 {
              tunnel: [w2050 w2055] -> w2027
              tunnel: [w2049 w2054] -> w2026
              tunnel: w2030 -> [_ w2053]
              tunnel: w2018 -> [w2050 w2052]
              tunnel: w2017 -> [w2049 w2051]
              frame False {
              }
              frame True {
                n1054 = VISA Write(VISA resource name=w2052, write buffer=w2053, error in (no error)=w2051) -> (VISA resource name out=w2055:refnum<visa-resource-name>, error out=w2054:errorcluster)  [unwired: 1 out]
              }
            }
            n1055 = case shown="False" w2031 {
              tunnel: [w2057 w2062] -> w2034
              tunnel: [w2056 w2061] -> w2033
              tunnel: w2032 -> [_ w2060]
              tunnel: w2016 -> [w2057 w2059]
              tunnel: w2015 -> [w2056 w2058]
              frame False {
              }
              frame True {
                n1056 = VISA Write(VISA resource name=w2059, write buffer=w2060, error in (no error)=w2058) -> (VISA resource name out=w2062:refnum<visa-resource-name>, error out=w2061:errorcluster)  [unwired: 1 out]
              }
            }
            n1057 = case shown="False" w2022 {
              tunnel: [w2043 w2048] -> w2021
              tunnel: [w2042 w2047] -> w2020
              tunnel: w2029 -> [_ w2046]
              tunnel: w2014 -> [w2043 w2045]
              tunnel: w2013 -> [w2042 w2044]
              frame False {
              }
              frame True {
                n1058 = VISA Write(VISA resource name=w2045, write buffer=w2046, error in (no error)=w2044) -> (VISA resource name out=w2048:refnum<visa-resource-name>, error out=w2047:errorcluster)  [unwired: 1 out]
              }
            }
            n1059 = case shown="False" w2025 {
              tunnel: [w2036 w2041] -> w2024
              tunnel: [w2035 w2040] -> w2023
              tunnel: w2028 -> [_ w2039]
              tunnel: w2012 -> [w2036 w2038]
              tunnel: w2011 -> [w2035 w2037]
              frame False {
              }
              frame True {
                n1060 = VISA Write(VISA resource name=w2038, write buffer=w2039, error in (no error)=w2037) -> (VISA resource name out=w2041:refnum<visa-resource-name>, error out=w2040:errorcluster)  [unwired: 1 out]
              }
            }
          }
          frame #2 {
            n1061 = call "Time Delay7"("Delay Time (s)"=0.1) -> ()  [unwired: 10 in, 1 out]
          }
          frame #3 {
            n1062 = case shown="True" w2088 {
              tunnel: w2090 -> [w2115 w2119]
              tunnel: w2089 -> [w2114 w2118]
              tunnel: [w2115 w2117] -> w2077
              tunnel: [w2114 w2116] -> w2076
              frame False {
              }
              frame True {
                n1063 = property class="Instr"(reference=w2119, error in=w2118) -> (reference out=w2121:refnum<visa-resource-name>, error out=w2120:errorcluster, "Serial Settings:Number of Bytes at Serial Port"=w2122:u32)
                n1064 = VISA Read(VISA resource name=w2121, byte count=w2122, error in (no error)=w2120) -> (VISA resource name out=w2117:refnum<visa-resource-name>, error out=w2116:errorcluster)  [unwired: 2 out]
              }
            }
            n1065 = case shown="True" w2091 {
              tunnel: w2095 -> [w2124 w2128]
              tunnel: w2094 -> [w2123 w2127]
              tunnel: [w2124 w2126] -> w2093
              tunnel: [w2123 w2125] -> w2092
              frame False {
              }
              frame True {
                n1066 = property class="Instr"(reference=w2128, error in=w2127) -> (reference out=w2130:refnum<visa-resource-name>, error out=w2129:errorcluster, "Serial Settings:Number of Bytes at Serial Port"=w2131:u32)
                n1067 = VISA Read(VISA resource name=w2130, byte count=w2131, error in (no error)=w2129) -> (VISA resource name out=w2126:refnum<visa-resource-name>, error out=w2125:errorcluster)  [unwired: 2 out]
              }
            }
            n1068 = case shown="True" w2084 {
              tunnel: w2083 -> [w2097 w2101]
              tunnel: w2082 -> [w2096 w2100]
              tunnel: [w2097 w2099] -> w2081
              tunnel: [w2096 w2098] -> w2080
              frame False {
              }
              frame True {
                n1069 = property class="Instr"(reference=w2101, error in=w2100) -> (reference out=w2103:refnum<visa-resource-name>, error out=w2102:errorcluster, "Serial Settings:Number of Bytes at Serial Port"=w2104:u32)
                n1070 = VISA Read(VISA resource name=w2103, byte count=w2104, error in (no error)=w2102) -> (VISA resource name out=w2099:refnum<visa-resource-name>, error out=w2098:errorcluster)  [unwired: 2 out]
              }
            }
            n1071 = case shown="True" w2087 {
              tunnel: w2086 -> [w2106 w2110]
              tunnel: w2085 -> [w2105 w2109]
              tunnel: [w2106 w2108] -> w2079
              tunnel: [w2105 w2107] -> w2078
              frame False {
              }
              frame True {
                n1072 = property class="Instr"(reference=w2110, error in=w2109) -> (reference out=w2112:refnum<visa-resource-name>, error out=w2111:errorcluster, "Serial Settings:Number of Bytes at Serial Port"=w2113:u32)
                n1073 = VISA Read(VISA resource name=w2112, byte count=w2113, error in (no error)=w2111) -> (VISA resource name out=w2108:refnum<visa-resource-name>, error out=w2107:errorcluster)  [unwired: 2 out]
              }
            }
          }
          frame #4 {
            n1074 = property on="Y Scan" class="Bool (strict)"("Val(Sgnl)"=FALSE ("Slew Ready 2")) -> ()  [unwired: 2 in, 2 out]
            n1075 = property on="X Scan" class="Bool (strict)"("Val(Sgnl)"=FALSE ("Slew Ready 2")) -> ()  [unwired: 2 in, 2 out]
            n1076 = property on="R Scan" class="Bool (strict)"("Val(Sgnl)"=FALSE ("Slew Ready 2")) -> ()  [unwired: 2 in, 2 out]
            n1077 = property on="Z Scan" class="Bool (strict)"("Val(Sgnl)"=FALSE ("Slew Ready 2")) -> ()  [unwired: 2 in, 2 out]
            n1078 = property on="Z Scan Velocity SP steps/sec" class="DigNum (strict)"("DisabledEnum"=T2."Enabled" ("Disabled")) -> ()  [unwired: 2 in, 2 out]
            n1079 = property on="R Scan Length SP steps" class="DigNum (strict)"("DisabledEnum"=T2."Enabled" ("Disabled")) -> ()  [unwired: 2 in, 2 out]
            n1080 = property on="X Scan Length SP steps" class="DigNum (strict)"("DisabledEnum"=T2."Enabled" ("Disabled")) -> ()  [unwired: 2 in, 2 out]
            n1081 = property on="R Scan Velocity SP steps/sec" class="DigNum (strict)"("DisabledEnum"=T2."Enabled" ("Disabled")) -> ()  [unwired: 2 in, 2 out]
            n1082 = property on="X Scan Velocity SP steps/sec" class="DigNum (strict)"("DisabledEnum"=T2."Enabled" ("Disabled")) -> ()  [unwired: 2 in, 2 out]
            n1083 = property on="Y Scan Length SP steps" class="DigNum (strict)"("DisabledEnum"=T2."Enabled" ("Disabled")) -> ()  [unwired: 2 in, 2 out]
            n1084 = property on="Z Scan Length SP steps" class="DigNum (strict)"("DisabledEnum"=T2."Enabled" ("Disabled")) -> ()  [unwired: 2 in, 2 out]
            n1085 = property on="Y Scan Selocity SP steps/sec" class="DigNum (strict)"("DisabledEnum"=T2."Enabled" ("Disabled")) -> ()  [unwired: 2 in, 2 out]
            n1086 = property on="Scan Cancel" class="Bool"("DisabledEnum"=T2."Disabled and Grayed Out" ("Disabled")) -> ()  [unwired: 2 in, 2 out]
            n1087 = property on="Scan Go" class="Bool"("DisabledEnum"=T2."Disabled and Grayed Out" ("Disabled")) -> ()  [unwired: 2 in, 2 out]
          }
        }
      }
      event "Reset": Mouse Down {
        n1088 = event-data() -> ()  [unwired: 1 in, 7 out]
        n1089 = flat-sequence {
          tunnel: [w2184] -> w2163
          tunnel: w2164 -> [w2187]
          tunnel: [w2186] -> w2162
          tunnel: w2165 -> [w2185]
          frame #0 {
            n1090 = property on="Reset X Motor Steps" class="DigNum (strict)"() -> ("Value"=w2188:i32)  [unwired: 2 in, 2 out]
            n1091 = Number To Decimal String(number=w2188) -> (decimal integer string=w2189:string)  [unwired: 1 in]
            n1092 = call "mDrive Send Command.vi"("error in (no error)"=w2187, "Extra"=w2189, "Command"=T1."Set Current Position", "VISA resource name"=w2185) -> ("error out"=w2186:errorcluster, "VISA resource name out"=w2184:refnum<visa-resource-name>)  [unwired: 3 in, 1 out]
          }
        }
        n1093 = flat-sequence {
          tunnel: w2169 -> [w2194]
          tunnel: w2168 -> [w2193]
          tunnel: [w2192] -> w2167
          tunnel: [w2191] -> w2166
          frame #0 {
            n1094 = property on="Reset Y Motor Steps" class="DigNum (strict)"() -> ("Value"=w2195:i32)  [unwired: 2 in, 2 out]
            n1095 = Number To Decimal String(number=w2195) -> (decimal integer string=w2196:string)  [unwired: 1 in]
            n1096 = call "mDrive Send Command.vi"("error in (no error)"=w2193, "Extra"=w2196, "Command"=T1."Set Current Position", "VISA resource name"=w2194) -> ("error out"=w2191:errorcluster, "VISA resource name out"=w2192:refnum<visa-resource-name>)  [unwired: 3 in, 1 out]
          }
        }
        n1097 = flat-sequence {
          tunnel: [w2171] -> w2157
          tunnel: [w2173] -> w2156
          tunnel: w2159 -> [w2172]
          tunnel: w2158 -> [w2170]
          frame #0 {
            n1098 = property on="Reset R Motor Steps" class="DigNum (strict)"() -> ("Value"=w2174:i32)  [unwired: 2 in, 2 out]
            n1099 = Number To Decimal String(number=w2174) -> (decimal integer string=w2175:string)  [unwired: 1 in]
            n1100 = call "mDrive Send Command.vi"("error in (no error)"=w2170, "Extra"=w2175, "Command"=T1."Set Current Position", "VISA resource name"=w2172) -> ("error out"=w2173:errorcluster, "VISA resource name out"=w2171:refnum<visa-resource-name>)  [unwired: 3 in, 1 out]
          }
        }
        n1101 = flat-sequence {
          tunnel: [w2180] -> w2155
          tunnel: [w2179] -> w2154
          tunnel: w2161 -> [w2178]
          tunnel: w2160 -> [w2177]
          frame #0 {
            n1102 = property on="Reset Z Motor Steps" class="DigNum (strict)"() -> ("Value"=w2181:i32)  [unwired: 2 in, 2 out]
            n1103 = Number To Decimal String(number=w2181) -> (decimal integer string=w2182:string)  [unwired: 1 in]
            n1104 = call "mDrive Send Command.vi"("error in (no error)"=w2177, "Extra"=w2182, "Command"=T1."Set Current Position", "VISA resource name"=w2178) -> ("error out"=w2179:errorcluster, "VISA resource name out"=w2180:refnum<visa-resource-name>)  [unwired: 3 in, 1 out]
          }
        }
      }
    }
    n1105 = property on="Preset positions" class="Ring (strict)"() -> ("Strings []"=w454:string[])  [unwired: 2 in, 2 out]
    n1106 = case shown="True" "Set Button" {
      tunnel: "Preset positions" -> [_ w520]
      frame False {
      }
      frame True {
        n1107 = property on="Presets" class="Arr (strict)"() -> ("Value"=w517:i32[][])  [unwired: 2 in, 2 out]
        n1108 = Index Array(array=w517, index (row)=w520) -> (element=w519:i32[])  [unwired: 1 in]
        n1109 = Array To Cluster(array=w519) -> (cluster=w518:T5)
        n1110 = Unbundle(w518) -> ("Value[0]"=w516:i32, "Value[1]"=w515:i32, "Value[2]"=w514:i32, "Value[3]"=w513:i32)  [unwired: 5 out]
        n1111 = property on="X Step SP" class="DigNum (strict)"("Val(Sgnl)"=w516) -> ()  [unwired: 2 in, 2 out]
        n1112 = property on="Y Step SP" class="DigNum (strict)"("Val(Sgnl)"=w515) -> ()  [unwired: 2 in, 2 out]
        n1113 = property on="Z Step SP" class="DigNum (strict)"("Val(Sgnl)"=w514) -> ()  [unwired: 2 in, 2 out]
        n1114 = property on="R Step SP" class="DigNum (strict)"("Val(Sgnl)"=w513) -> ()  [unwired: 2 in, 2 out]
      }
    }
    n1115 = case shown="True" "Add Button" {
      tunnel: w454 -> [_ w512]
      frame False {
      }
      frame True {
        n1116 = property on="X Step PV" class="DigNum (strict)"() -> ("Value"=w507:i32)  [unwired: 2 in, 2 out]
        n1117 = property on="Y Step PV" class="DigNum (strict)"() -> ("Value"=w506:i32)  [unwired: 2 in, 2 out]
        n1118 = property on="Z Step PV" class="DigNum (strict)"() -> ("Value"=w505:i32)  [unwired: 2 in, 2 out]
        n1119 = property on="R Step PV" class="DigNum (strict)"() -> ("Value"=w504:i32)  [unwired: 2 in, 2 out]
        n1120 = Build Array(w507, w506, w505, w504) -> (w510:i32[])
        n1121 = Build Array (concatenate)(w512, "String") -> (w511:string[])
        n1122 = property on="Preset positions" class="Ring (strict)"("Strings []"=w511) -> ()  [unwired: 2 in, 2 out]
        n1123 = property on="Presets" class="Arr (strict)"() -> ("Value"=w509:i32[][])  [unwired: 2 in, 2 out]
        n1124 = Build Array (concatenate)(w509, w510) -> (w503:i32[][])
        n1125 = property on="Presets" class="Arr (strict)"("Val(Sgnl)"=w503) -> ()  [unwired: 2 in, 2 out]
      }
    }
    n1126 = case shown="True" "Delete Button" {
      tunnel: w454 -> [_ w502]
      frame False {
      }
      frame True {
        n1127 = property on="Preset positions" class="Ring (strict)"() -> ("Value"=w500:i32)  [unwired: 2 in, 2 out]
        n1128 = Delete From Array(array=w502, index=w500) -> (array with subset deleted=w501:string[])  [unwired: 1 in, 1 out]
        n1129 = property on="Presets" class="Arr (strict)"() -> ("Value"=w499:i32[][])  [unwired: 2 in, 2 out]
        n1130 = property on="Preset positions" class="Ring (strict)"("Strings []"=w501) -> ()  [unwired: 2 in, 2 out]
        n1131 = Delete From Array(array=w499, index (row)=w500) -> (array with subset deleted=w498:i32[][])  [unwired: 2 in, 1 out]
        n1132 = property on="Presets" class="Arr (strict)"("Val(Sgnl)"=w498) -> ()  [unwired: 2 in, 2 out]
      }
    }
    n1133 = call "DigitalIO_sub_V5_MON.vi"() -> ("CL"=w450:bool, "OP"=w451:bool)  [unwired: 8 in]
    n1134 = property on="IV5OP" class="Bool (strict)"("Value"=w451) -> ()  [unwired: 2 in, 2 out]
    n1135 = property on="IV5CL" class="Bool (strict)"("Value"=w450) -> ()  [unwired: 2 in, 2 out]
  }
  n1136 = flat-sequence {
    tunnel: w90 -> [w2203]
    tunnel: w89 -> [w2201]
    tunnel: [w2198] -> w26
    frame #0 {
      n1137 = call "mDrive Send Command.vi"("error in (no error)"=w2201, "Extra"="P", "Command"=T1."Print Parameter", "VISA resource name"=w2203) -> ("error out"=w2200:errorcluster, "read buffer"=w2207:string, "VISA resource name out"=w2202:refnum<visa-resource-name>)  [unwired: 3 in]
      n1138 = call "mDrive Send Command.vi"("error in (no error)"=w2200, "Command"=T1."Stop", "VISA resource name"=w2202) -> ("error out"=w2209:errorcluster, "VISA resource name out"=w2210:refnum<visa-resource-name>)  [unwired: 4 in, 1 out]
      n1139 = Decimal String To Number(string=w2207, offset=0) -> (number=w2199:i32)  [unwired: 1 in, 1 out]
      n1140 = To Long Integer(number=w2199) -> (32bit integer=w2198:i32)
      n1141 = VISA Close(VISA resource name=w2210, error in (no error)=w2209) -> ()  [unwired: 1 out]
    }
  }
  n1142 = flat-sequence {
    tunnel: w30 -> [w2216]
    tunnel: w29 -> [w2214]
    tunnel: [w2211] -> w25
    frame #0 {
      n1143 = call "mDrive Send Command.vi"("error in (no error)"=w2214, "Extra"="P", "Command"=T1."Print Parameter", "VISA resource name"=w2216) -> ("error out"=w2213:errorcluster, "read buffer"=w2220:string, "VISA resource name out"=w2215:refnum<visa-resource-name>)  [unwired: 3 in]
      n1144 = call "mDrive Send Command.vi"("error in (no error)"=w2213, "Command"=T1."Stop", "VISA resource name"=w2215) -> ("error out"=w2222:errorcluster, "VISA resource name out"=w2223:refnum<visa-resource-name>)  [unwired: 4 in, 1 out]
      n1145 = Decimal String To Number(string=w2220, offset=0) -> (number=w2212:i32)  [unwired: 1 in, 1 out]
      n1146 = To Long Integer(number=w2212) -> (32bit integer=w2211:i32)
      n1147 = VISA Close(VISA resource name=w2223, error in (no error)=w2222) -> ()  [unwired: 1 out]
    }
  }
  n1148 = flat-sequence {
    tunnel: w32 -> [w2229]
    tunnel: w31 -> [w2227]
    tunnel: [w2224] -> w24
    frame #0 {
      n1149 = call "mDrive Send Command.vi"("error in (no error)"=w2227, "Extra"="P", "Command"=T1."Print Parameter", "VISA resource name"=w2229) -> ("error out"=w2226:errorcluster, "read buffer"=w2233:string, "VISA resource name out"=w2228:refnum<visa-resource-name>)  [unwired: 3 in]
      n1150 = call "mDrive Send Command.vi"("error in (no error)"=w2226, "Command"=T1."Stop", "VISA resource name"=w2228) -> ("error out"=w2235:errorcluster, "VISA resource name out"=w2236:refnum<visa-resource-name>)  [unwired: 4 in, 1 out]
      n1151 = Decimal String To Number(string=w2233, offset=0) -> (number=w2225:i32)  [unwired: 1 in, 1 out]
      n1152 = To Long Integer(number=w2225) -> (32bit integer=w2224:i32)
      n1153 = VISA Close(VISA resource name=w2236, error in (no error)=w2235) -> ()  [unwired: 1 out]
    }
  }
  n1154 = flat-sequence {
    tunnel: w28 -> [w2242]
    tunnel: w27 -> [w2240]
    tunnel: [w2237] -> w23
    frame #0 {
      n1155 = call "mDrive Send Command.vi"("error in (no error)"=w2240, "Extra"="P", "Command"=T1."Print Parameter", "VISA resource name"=w2242) -> ("error out"=w2239:errorcluster, "read buffer"=w2246:string, "VISA resource name out"=w2241:refnum<visa-resource-name>)  [unwired: 3 in]
      n1156 = call "mDrive Send Command.vi"("error in (no error)"=w2239, "Command"=T1."Stop", "VISA resource name"=w2241) -> ("error out"=w2248:errorcluster, "VISA resource name out"=w2249:refnum<visa-resource-name>)  [unwired: 4 in, 1 out]
      n1157 = Decimal String To Number(string=w2246, offset=0) -> (number=w2238:i32)  [unwired: 1 in, 1 out]
      n1158 = To Long Integer(number=w2238) -> (32bit integer=w2237:i32)
      n1159 = VISA Close(VISA resource name=w2249, error in (no error)=w2248) -> ()  [unwired: 1 out]
    }
  }
  n1160 = flat-sequence {
    tunnel: w26 -> [w2255]
    tunnel: w25 -> [w2254]
    tunnel: w24 -> [w2253]
    tunnel: w23 -> [w2252]
    frame #0 {
      n1161 = Build Array(w2255, w2254, w2253, w2252) -> (w2250:i32[])
      n1162 = call-poly <vilib>:"Write To Spreadsheet File.vi"("1D data"=w2250, "file path (dialog if empty)"=path "S:/SSE/IMS/POS.TXT") -> ()  [unwired: 6 in, 1 out]
    }
    frame #1 {
      n1163 = property on="Presets" class="Arr (strict)"() -> ("Value"=w2262:i32[][])  [unwired: 2 in, 2 out]
      n1164 = property on="Preset positions" class="Ring (strict)"() -> ("Strings []"=w2258:string[])  [unwired: 2 in, 2 out]
      n1165 = Number To Decimal String(number=w2262) -> (decimal integer string=w2256:string[][])  [unwired: 1 in]
      n1166 = Transpose 2D Array(2D array=w2256) -> (transposed array=w2257:string[][])
      n1167 = Build Array (concatenate)(w2258, w2257) -> (w2259:string[][])
      n1168 = Transpose 2D Array(2D array=w2259) -> (transposed array=w2260:string[][])
      n1169 = call-poly <vilib>:"Write To Spreadsheet File.vi"("2D data"=w2260, "file path (dialog if empty)"=path "S:/SSE/IMS/PRESET.TXT") -> ()  [unwired: 6 in, 1 out]
    }
  }
